vi "FIB MICROSCOPE VIEWER.vi"() -> ()   [LabVIEW 2018]
uses:
  <vilib>/userdefined/High Color/IMAQdx.ctl
  <vilib>/vision/driver/IMAQdx.llb/IMAQdx Attribute Type.ctl
  Mikrodaq/Microdaq FPGA Development/IBA METHODS.ctl
  <vilib>/vision/driver/IMAQdx.llb/IMAQdx Camera Control Mode.ctl
  <vilib>/vision/driver/IMAQdx.llb/IMAQdx Buffer Number Mode.ctl
  <vilib>/Utility/file.llb/Read From Spreadsheet File (string).vi
  <vilib>/Utility/file.llb/Write To Spreadsheet File (DBL).vi
  <vilib>/vision/driver/NI_Vision_Acquisition_Software.lvlib
  <resource>/objmgr/imaqdx.rc
  <vilib>/vision/NI_Vision_Development_Module.lvlib
panel:
  out "CURRENT ZOOM CAL":dbl
  in  "GOTO COMBO":bool=TRUE
  out "QUEU TOGGLE":bool[](array[boolean])
  out "SCAN LIST ARRAY":T2(array[cluster]) {"dQ" format="%_4g"; "DOSE NORM" items=["DWELL TIME", "TOTAL CHARGE", "STEPX"]; "SCAN ORIGIN"."Z" format="%_5g"; "SCAN ORIGIN"."Y" format="%_5g"; "SCAN ORIGIN"."X" format="%_5g"; "SCANNING"."X-AMP" format="%_4f"; "SCANNING"."dX" min=1e-07 max=9.999999999999999e-05 step=1e-07 format="%#_3g"; "SCANNING"."dY" min=1e-07 max=9.999999999999999e-05 step=1e-07 format="%#_3g"; "SCANNING"."Y-AMP" format="%_4f"; "MODE & METHOD"."SCANNING METH" items=["RASTER", "SNAKE RASTER", "SPIRAL RASTER"]; "MODE & METHOD"."SCAN MODE" items=["XY-BEAM", "STEP", "XY-STAGE", "POINT", "SHAPE"]; "Q" format="%_4g"}
  out "POINT":T3={"X"=-0.005539110651703474, "Y"=-0.004695478539077235, "Z"=0.0001} {"Z" format="%_4g"; "X" format="%#_4g"; "Y" format="%#_4g"}
  out "Horizontal Graduated Bar":sgl(slide) scale=0.0..1.0
  in  "SCANNING DIMENSIONS":cluster{"XPIXELS":i32, "YPIXELS":i32}={"XPIXELS"=51, "YPIXELS"=51}
  in  "BUFFERED PIXELS":u32
  out "EXT POINTS ROW":i32
  out "Image Area:Size:All Elements":cluster{"Width":u32, "Height":u32}
  out "NEW ROI":T4
  out "BEAM OFFSET":cluster{"X":dbl[unit], "Y":dbl[unit]}
  out "IMAGE YCENTRE":dbl
  out "IMAGE XCENTRE":dbl
  in  "BINNING":i64=1
  in  "MAPS":enum32{"PIXE", "PIGE"}(tab)
  in  "EXCHANGE":bool
  in  "RECORD AVI VIDEO":bool
  in  "QUESTAR":i32(ring) items=["HOLE", "ZOOM 1", "ZOOM 2", "ZOOM 3"]
  in  "SAMPLE HOLDER":u16(ring)=1 items=["SLIDE HOLDER #1", "GEOSTUB #1", "GEOSTUB #2", "TOMOSTAGE"]
  in  "SCALE BAR":bool
  in  "GRID I":bool
  in  "QUARTZ":bool
  in  "RUBY":bool
  in  "YAG":bool
  in  "YAP":bool
  out "TRANS POINT ARRAY":T5(array[cluster]) {"Z" format="%_4g"; "X" format="%_6g"; "Y" format="%_6f"}
  out "EXT POINTS ARRAY":T5(array[cluster]) {"Z" format="%_4g"; "X" format="%_6g"; "Y" format="%_6f"}
  in  "REFLECTIVITY":bool
  out "ANGLE 2":sgl=1.5516903
  in  "ANGLE":sgl format="%.2f"
  in  "EXPOSURE":dbl(slide)=106.26827541712952 min=1.0 max=2500.0 step=10.0 scale=5.0..5000.0 scale format="%#_3f"
  in  "SCAN QUEU ARRAY":T6(array[cluster]) {"SCANNING MODE AND METHOD"."SCANNING METH" items=["RASTER", "SNAKE RASTER", "SPIRAL RASTER"]; "SCANNING MODE AND METHOD"."SCAN MODE" items=["XY", "STEP", "SHAPE", "STAGE", "COMBO", "POINT", "LINE"]; "DOSE NORM" items=["DWELL TIME", "TOTAL CHARGE", "LIVE CHARGE", "STEPPER PIXELATION"]; "Q PER PULSE" items=["1pC", "0.1pC", "0.01pC"]; "BEAMSCANNING"."dX" min=1e-07 max=9.999999999999999e-05 step=1e-07 format="%_3g"; "BEAMSCANNING"."dY" min=1e-07 max=9.999999999999999e-05 step=1e-07 format="%_3g"; "IBA METHODS" items=["LEFT PIXE", "RIGHT PIXE", "PIGE", "RBS", "HS-IONOLUMINESCENCE", "PIL", "SECONDARY ELECTRONS", "NONE"]; "SCAN ORIGIN"."Z" format="%_6f"; "SCAN ORIGIN"."X" format="%_6f"; "SCAN ORIGIN"."Y" format="%_6f"}
  in  "TOMO POINT":bool
  out "REL XYZ STAGE":T7={"X"=0.005497, "Y"=0.00465, "Z"=-0.0001} {"Z" format="%#_6f"; "X" format="%#_6f"; "Y" format="%#_6f"}
  out "FIB SAMPLE":T8="CSIRO-SAMPLE" caption="Session Out"
  in  "Tab Control 2":T9(tab)
  out "SCAN COMPLETE":bool
  in  "GOTO SCAN ORIGIN":bool
  in  "POSITION":T3 {"Z" format="%_5g"; "Y" format="%_5g"; "X" format="%_5g"}
  in  "START":bool
  in  "PAUSE DATA COLLECTION":bool
  in  "Tab Control 4":T10(tab)
  out "SCAN ROW 2":i32
  in  "START SEQ":bool
  in  "LOAD NMP LIST":bool
  in  "SAVE LIST":bool
  in  "RESET POINTS":bool
  in  "MINUS POINT":bool
  in  "ADD POINT TO LIST":bool
  in  "ION ENERGY":dbl[unit]=4.80652926e-13 format="%_2g"
  in  "BEAM":i8(ring) items=["Protons", "Molecular Hydrogen", "Alpha", "Carbon"]
  in  "NAME":string="test"
  in  "USER":string="jslaird"
  in  "COMMENT":string
  out "SCAN LIST":string[][](table)
  in  "X":bool=TRUE
  in  "Y":bool=TRUE
  in  "Z":bool=TRUE
  in  "GOTO LIST POINT":bool
  in  "SET SCAN FROM LIST":bool
  out "SCAN ROW":i32
  in  "QUEU":bool
  in  "Q":dbl[unit]=2e-09 format="%#_4g"
  in  "DWELL":sgl[unit]=0.1
  in  "PIXEL DEPTH":bool
  in  "dQ":sgl[unit]=1e-10 format="%#_6f"
  in  "dt":sgl[unit]=0.1 caption="dDWELL"
  in  "MIN DWELL":sgl[unit]=0.1
  out "TIME":dbl[unit]=399.9999910593033
  out "CHARGE":dbl[unit]=1.5999999642372133e-06
  in  "LINE PASSES":i32=1
  in  "OVERSCAN":i32=1 min=1 max=100 step=1
  in  "OPTIMISE BEAM":bool
  in  "OBJECT RANGE":i32(ring) items=["100um", "150um", "200um", "250um", "300um", "500um ", "0-1mm Variable", "1mm Aperture", "2mm Aperture", "5mm Aperture", "OPEN"]
  out "Q per PIXEL":dbl[unit] format="%_3g"
  out "TOP  STOP":T3={"X"=-0.005999838337298367, "Y"=-0.004138182607217211, "Z"=9.999999747378752e-05} {"X" format="%_4g"; "Y" format="%#_4g"}
  out "BOTTOM START":T3={"X"=-0.005999838337298367, "Y"=-0.004138182607217211, "Z"=9.999999747378752e-05} {"X" format="%#_4g"; "Y" format="%#_4g"}
  out "DIRECTION":u8(ring) items=["MINUS", "PLUS"]
  out "XAMP":dbl[unit]=0.00044297647174286817 format="%_4g"
  out "XORIGIN":dbl[unit]=-0.02202153716924597 format="%_5g"
  in  "STOP":bool
  in  "START":bool
  out "BOTTOM STOP":T3={"X"=-0.005999838337298367, "Y"=-0.004138182607217211, "Z"=9.999999747378752e-05} {"X" format="%_4g"; "Y" format="%#_4g"}
  out "TOP START":T3={"X"=-0.005999838337298367, "Y"=-0.004138182607217211, "Z"=9.999999747378752e-05} {"X" format="%#_4g"; "Y" format="%#_4g"}
  out "YORIGIN":dbl[unit]
  out "YAMP":dbl[unit]=0.00044297647174286817 format="%_4g"
  out "XAMP":dbl[unit]=0.00044297647174286817 format="%_4g"
  out "XORIGIN":dbl[unit]=-0.02202153716924597 format="%_5g"
  out "YORIGIN":dbl[unit]
  out "YAMP":dbl[unit]=0.00044297647174286817 format="%_4g"
  in  "STOP ROI":bool
  in  "START ROI":bool
  out "BOTTOM RIGHT":T3={"X"=-0.005539110651703474, "Y"=-0.004695478539077235, "Z"=0.0001} {"Z" format="%#_5g"; "X" format="%#_5g"; "Y" format="%#_5g"}
  out "TOP LEFT":T3={"X"=-0.005539110651703474, "Y"=-0.004695478539077235, "Z"=0.0001} {"Z" format="%#_5g"; "X" format="%#_5g"; "Y" format="%#_5g"}
  in  "STAGE VELOCITIES":T11={"XS VEL"=0.002, "YS VEL"=0.002, "Z VEL"=0.001} {"XS VEL" format="%_2f"}
  in  "SCAN CALIBRATIONS":cluster{"XB CAL":dbl[unit], "YB CAL":dbl[unit]}={"XB CAL"=0.00035, "YB CAL"=9.999999999999999e-05}
  in  "SCANNING":T12={"X-AMP"=0.1, "dX"=1e-06, "Y-AMP"=9.999999999999999e-05, "dY"=5e-07, "X-SHIFT"=0.0, "Y-SHIFT"=0.0, "THETA"=0.0, "PHI"=0.0} {"X-AMP" format="%_4f"; "dX" min=1e-07 max=9.999999999999999e-05 step=1e-07 format="%#_3g"; "dY" min=1e-07 max=9.999999999999999e-05 step=1e-07 format="%#_3g"; "Y-AMP" format="%_4f"}
  in  "REPEAT LINE":bool
  in  "MODE & METHOD":cluster{"SCAN MODE":u16, "SCANNING METH":u16}={"SCAN MODE"=2, "SCANNING METH"=1} {"SCANNING METH" items=["RASTER", "SNAKE RASTER", "SPIRAL RASTER"]; "SCAN MODE" items=["XY-BEAM", "STEP", "XY-STAGE", "POINT", "SHAPE"]}
  in  "BEAM CENTRE":bool
  in  "CENTRE STAGE":bool
  in  "SHOW MIRROR":bool=TRUE
  in  "SHOW POSITION":bool=TRUE
  in  "CLEAR ROI":bool
  in  "SHOW BEAM":bool=TRUE
  in  "SHOW SCALE BAR":bool=TRUE
  in  "CAMERA CENTRE":bool=TRUE
  in  "Tab Control":T13(tab)
  in  "RELATIVE":bool
  in  "GOTO GEOSTUB #1 APERTURE":bool=TRUE
  in  "DEFINE APERTURE":bool=TRUE
  in  "RELATIVE MOVE":T3={"X"=-0.004777999999999999, "Y"=-0.0063197, "Z"=9.999999999999999e-05} {"Z" format="%#_5g"; "X" format="%#_5g"; "Y" format="%#_5g"}
  in  "WOBBLEZ":bool
  in  "DOWN":bool
  in  "UP":bool
  in  "DX":dbl[unit]=9.999999999999999e-06 format="%_4f"
  in  "SPEED":u16(ring)=1 items=["SNAIL PACE", "SLOW", "NORMAL", "FAST", "RAPID", "CUSTOM", ""]
  in  "LEFT":bool
  in  "RIGHT":bool
  in  "DZ":dbl[unit]=9.999999999999999e-06 format="%_3f"
  in  "DY":dbl[unit]=9.999999999999999e-06 format="%_3f"
  in  "OUT":bool
  in  "IN":bool
  in  "ABORT":bool
  in  "GOTO POSITION":T3={"X"=-0.004777999999999999, "Y"=-0.0063197, "Z"=9.999999999999999e-05} {"Z" format="%#_5g"; "X" format="%#_5g"; "Y" format="%#_5g"}
  out "SCAN ORIGIN":T3={"X"=-0.005539110651703474, "Y"=-0.004695478539077235, "Z"=0.0001} {"Z" format="%#_5g"; "X" format="%#_5g"; "Y" format="%#_5g"}
  out "LOST CONNECTION?":bool
  in  "BEAM  SCANNER":bool=TRUE
  in  "FARADAY CUP":bool
  in  "Tab Control 5":enum32{"EXTERNAL TRANSLATION", "NOTES"}(tab)
  in  "SET ACCURATE LANDMARK":bool
  in  "TRANS":bool
  out "NMP ORDER OK ?":bool
  in  "GOTOF2":bool
  in  "REF#1":T3={"X"=0.035034294595390356, "Y"=-0.0014485573931861046, "Z"=-0.0018100000000000002} {"Z" format="%#_5g"; "X" format="%#_5g"; "Y" format="%#_5g"}
  in  "REF#2":T3={"X"=0.011754294595390355, "Y"=-0.012118557393186105, "Z"=-0.0015600000000000002} {"Z" format="%#_5g"; "X" format="%#_5g"; "Y" format="%#_5g"}
  in  "GOTOF1":bool
  in  "SET FIDUCIAL 2":bool
  in  "SET FIDUCIAL 1":bool
  in  "LOAD":bool
  in  "SWAP REF#1/REF#2":bool
  in  "SCAN POINT LIST":path=path "C:/Users/jslaird/Dropbox/Working Data/Test Points on Pearce Gold.txt"
  out "EXTERNAL/TRANSLATED LIST":string[][](table)
  in  "GOTO LIST POINT 2":bool
  out "LANDMARKS FOR HOLDERS":T14(array[cluster])=[{"X"=0.0, "Y"=0.0, "Z"=0.0}, {"X"=-0.002142, "Y"=-0.00863, "Z"=0.00093}, {"X"=0.0, "Y"=0.0, "Z"=0.0}, {"X"=0.0, "Y"=0.0, "Z"=0.0}] {"Z" format="%_5g"; "Y" format="%_5g"; "X" format="%_5g"}
  out "XOFFSET":dbl[unit]
  out "YOFFSET":dbl[unit]
  in  "LOAD ROI":bool
  in  "DOSE NORM":i8(ring) items=["DWELL TIME", "TOTAL CHARGE", "STEPX"]
  in  "GLOBAL STOP":bool
  in  "BEAM CURRENT":dbl[unit]=1.0049748420715333e-12 format="%_4f"
  in  "USE CALIBRATION":bool
  in  "CALIBRATE VIEW":bool
  in  "LENGTH 2":bool
  in  "ROTATE VIEW":bool
  in  "SYMMETRY":bool
  in  "DSP ROI":T15
  in  "GAIN METHOD":u16(ring)=2 items=["OFF", "ONCE", "CONTINOUS"]
  in  "GAIN":sgl=1.0 min=0 max=31 step=1
  out "IP ADDRESS":string="192.168.1.10"
  out "CALIBRATION FACTOR":dbl=2.9930842685328876 format="%_4g"
  in  "CONFIGS":u16(ring) items=["MANUAL", "BEAM FOCUS", "SAMPLE VIEWING"]
  in  "IMAGE SYMMETRY":u32(ring)=2 items=["Horizontal", "Vertical", "CENTRAL", "1st Diagonal", "2nd Diagonal"]
  in  "HSCALEBAR POSITION TEXT":cluster{"X":i32, "Y":i32}={"X"=620, "Y"=995}
  in  "VSCALEBAR POSITION":cluster{"X":i32, "Y":i32}={"X"=50, "Y"=250}
  in  "HSCALEBAR POSITION":cluster{"X":i32, "Y":i32}={"X"=440, "Y"=970}
  in  "ZOOM CALIBRATION FACTORS":dbl[](array[numeric])=[1.0, 1.0, 0.8168558457268784, 1.0] format="%_4g"
  in  "ROI ZOOM":bool
  in  "ENABLE VIDEO LOOP":bool=TRUE
  in  "BRIGHT,CONT,GAMMA":cluster{"B":dbl, "C":dbl, "G":dbl}={"B"=250.0, "C"=67.0, "G"=1.6000000000000005} {"G" format="%_4g"; "C" format="%_4g"; "B" format="%_4g"}
  out "LENGTH":dbl=111.88537792376064
  in  "ENABLE STAGE AND DAQ LOOP":bool=TRUE
  out "XBCENTRE":sgl=679.0
  out "YBCENTRE":sgl=512.0
  out "BEAM TO STAGE OFFSETS":cluster{"X":dbl[unit], "Y":dbl[unit]}[](array[cluster])=[{"X"=0.0, "Y"=0.0}, {"X"=-0.00019428571428571433, "Y"=2.8571428571427717e-06}, {"X"=0.0, "Y"=0.0}, {"X"=0.0, "Y"=0.0}] {"X" format="%#_3g"; "Y" format="%#_3g"}
  out "MIRROR HOLE":T16={"Left"=478, "Top"=310, "Right"=546, "Bottom"=372}
  out "ERROR":string
  in  "AVI Path":path=path "C:/Users/jslaird/Desktop/test.avi"
  out "Attribute Information Array":T18(array[cluster])=[{"Attribute Type"=enum."DBL", "Readable"=TRUE, "Writable"=FALSE, "Attribute Name"="AcquisitionAttributes::AdvancedEthernet::BandwidthControl::ActualPeakBandwidth"}, {"Attribute Type"=enum."DBL", "Readable"=TRUE, "Writable"=TRUE, "Attribute Name"="AcquisitionAttributes::AdvancedEthernet::BandwidthControl::DesiredPeakBandwidth"}, {"Attribute Type"=enum."Enum", "Readable"=TRUE, "Writable"=TRUE, "Attribute Name"="AcquisitionAttributes::AdvancedEthernet::Controller::DestinationMode"}, {"Attribute Type"=enum."String", "Readable"=TRUE, "Writable"=TRUE, "Attribute Name"="AcquisitionAttributes::AdvancedEthernet::Controller::DestinationMulticastAddress"}, {"Attribute Type"=enum."Bool", "Readable"=TRUE, "Writable"=TRUE, "Attribute Name"="AcquisitionAttributes::AdvancedEthernet::EventParameters::EventsEnabled"}, {"Attribute Type"=enum."U32", "Readable"=TRUE, "Writable"=TRUE, "Attribute Name"="AcquisitionAttributes::AdvancedEthernet::EventParameters::MaxOutstandingEvents"}, {"Attribute Type"=enum."Bool", "Readable"=TRUE, "Writable"=TRUE, "Attribute Name"="AcquisitionAttributes::AdvancedEthernet::FirewallTraversal::Enabled"}, {"Attribute Type"=enum."U32", "Readable"=TRUE, "Writable"=TRUE, "Attribute Name"="AcquisitionAttributes::AdvancedEthernet::FirewallTraversal::KeepAliveTime"}, {"Attribute Type"=enum."Bool", "Readable"=TRUE, "Writable"=FALSE, "Attribute Name"="AcquisitionAttributes::AdvancedEthernet::FirewallTraversal::Supported"}, {"Attribute Type"=enum."U32", "Readable"=TRUE, "Writable"=TRUE, "Attribute Name"="AcquisitionAttributes::AdvancedEthernet::ResendParameters::MaxResendsPerPacket"}, {"Attribute Type"=enum."U32", "Readable"=TRUE, "Writable"=TRUE, "Attribute Name"="AcquisitionAttributes::AdvancedEthernet::ResendParameters::MemoryWindowSize"}, {"Attribute Type"=enum."U32", "Readable"=TRUE, "Writable"=TRUE, "Attribute Name"="AcquisitionAttributes::AdvancedEthernet::ResendParameters::MissingPacketTimeout"}, {"Attribute Type"=enum."U32", "Readable"=TRUE, "Writable"=TRUE, "Attribute Name"="AcquisitionAttributes::AdvancedEthernet::ResendParameters::NewPacketTimeout"}, {"Attribute Type"=enum."U32", "Readable"=TRUE, "Writable"=TRUE, "Attribute Name"="AcquisitionAttributes::AdvancedEthernet::ResendParameters::ResendBatchingPercentage"}, {"Attribute Type"=enum."U32", "Readable"=TRUE, "Writable"=TRUE, "Attribute Name"="AcquisitionAttributes::AdvancedEthernet::ResendParameters::ResendResponseTimeout"}, {"Attribute Type"=enum."U32", "Readable"=TRUE, "Writable"=TRUE, "Attribute Name"="AcquisitionAttributes::AdvancedEthernet::ResendParameters::ResendThresholdPercentage"}, {"Attribute Type"=enum."U32", "Readable"=TRUE, "Writable"=TRUE, "Attribute Name"="AcquisitionAttributes::AdvancedEthernet::ResendParameters::ResendTimerResolution"}, {"Attribute Type"=enum."Bool", "Readable"=TRUE, "Writable"=TRUE, "Attribute Name"="AcquisitionAttributes::AdvancedEthernet::ResendParameters::ResendsEnabled"}, {"Attribute Type"=enum."U32", "Readable"=TRUE, "Writable"=TRUE, "Attribute Name"="AcquisitionAttributes::AdvancedEthernet::TestPacketParameters::MaxTestPacketRetries"}, {"Attribute Type"=enum."Bool", "Readable"=TRUE, "Writable"=TRUE, "Attribute Name"="AcquisitionAttributes::AdvancedEthernet::TestPacketParameters::TestPacketEnabled"}, {"Attribute Type"=enum."U32", "Readable"=TRUE, "Writable"=TRUE, "Attribute Name"="AcquisitionAttributes::AdvancedEthernet::TestPacketParameters::TestPacketTimeout"}, {"Attribute Type"=enum."Enum", "Readable"=TRUE, "Writable"=TRUE, "Attribute Name"="CameraAttributes::GigE::StreamHold::StreamHoldEnable"}, {"Attribute Type"=enum."I64", "Readable"=TRUE, "Writable"=FALSE, "Attribute Name"="CameraAttributes::GigE::StreamHold::StreamHoldCapacity"}, {"Attribute Type"=enum."I64", "Readable"=TRUE, "Writable"=FALSE, "Attribute Name"="CameraAttributes::GigE::Timestamp::GevTimestampTickFrequency"}, {"Attribute Type"=enum."Command", "Readable"=FALSE, "Writable"=TRUE, "Attribute Name"="CameraAttributes::GigE::Timestamp::GevTimestampControlReset"}, {"Attribute Type"=enum."Enum", "Readable"=TRUE, "Writable"=TRUE, "Attribute Name"="CameraAttributes::GigE::PTP::PtpMode"}, {"Attribute Type"=enum."Enum", "Readable"=TRUE, "Writable"=FALSE, "Attribute Name"="CameraAttributes::GigE::PTP::PtpStatus"}, {"Attribute Type"=enum."I64", "Readable"=TRUE, "Writable"=TRUE, "Attribute Name"="CameraAttributes::GigE::PTP::PtpAcquisitionGateTime"}, {"Attribute Type"=enum."Enum", "Readable"=TRUE, "Writable"=TRUE, "Attribute Name"="CameraAttributes::Acquisition::Trigger::TriggerSelector"}, {"Attribute Type"=enum."Enum", "Readable"=TRUE, "Writable"=TRUE, "Attribute Name"="CameraAttributes::Acquisition::Trigger::TriggerMode"}, {"Attribute Type"=enum."Command", "Readable"=FALSE, "Writable"=TRUE, "Attribute Name"="CameraAttributes::Acquisition::Trigger::TriggerSoftware"}, {"Attribute Type"=enum."Enum", "Readable"=TRUE, "Writable"=TRUE, "Attribute Name"="CameraAttributes::Acquisition::Trigger::TriggerSource"}, {"Attribute Type"=enum."Enum", "Readable"=TRUE, "Writable"=TRUE, "Attribute Name"="CameraAttributes::Acquisition::Trigger::TriggerActivation"}, {"Attribute Type"=enum."Enum", "Readable"=TRUE, "Writable"=TRUE, "Attribute Name"="CameraAttributes::Acquisition::Trigger::TriggerOverlap"}, {"Attribute Type"=enum."DBL", "Readable"=TRUE, "Writable"=TRUE, "Attribute Name"="CameraAttributes::Acquisition::Trigger::TriggerDelayAbs"}, {"Attribute Type"=enum."I64", "Readable"=TRUE, "Writable"=TRUE, "Attribute Name"="CameraAttributes::Controls::DSPSubregion::DSPSubregionLeft"}, {"Attribute Type"=enum."I64", "Readable"=TRUE, "Writable"=TRUE, "Attribute Name"="CameraAttributes::Controls::DSPSubregion::DSPSubregionTop"}, {"Attribute Type"=enum."I64", "Readable"=TRUE, "Writable"=TRUE, "Attribute Name"="CameraAttributes::Controls::DSPSubregion::DSPSubregionRight"}, {"Attribute Type"=enum."I64", "Readable"=TRUE, "Writable"=TRUE, "Attribute Name"="CameraAttributes::Controls::DSPSubregion::DSPSubregionBottom"}, {"Attribute Type"=enum."Enum", "Readable"=TRUE, "Writable"=TRUE, "Attribute Name"="CameraAttributes::Controls::Exposure::ExposureMode"}, {"Attribute Type"=enum."DBL", "Readable"=TRUE, "Writable"=TRUE, "Attribute Name"="CameraAttributes::Controls::Exposure::ExposureTimeAbs"}, {"Attribute Type"=enum."Enum", "Readable"=TRUE, "Writable"=TRUE, "Attribute Name"="CameraAttributes::Controls::Exposure::ExposureAuto"}, {"Attribute Type"=enum."I64", "Readable"=TRUE, "Writable"=TRUE, "Attribute Name"="CameraAttributes::Controls::Exposure::ExposureAutoControl::ExposureAutoTarget"}, {"Attribute Type"=enum."Enum", "Readable"=TRUE, "Writable"=TRUE, "Attribute Name"="CameraAttributes::Controls::Exposure::ExposureAutoControl::ExposureAutoAlg"}, {"Attribute Type"=enum."I64", "Readable"=TRUE, "Writable"=TRUE, "Attribute Name"="CameraAttributes::Controls::Exposure::ExposureAutoControl::ExposureAutoMin"}, {"Attribute Type"=enum."I64", "Readable"=TRUE, "Writable"=TRUE, "Attribute Name"="CameraAttributes::Controls::Exposure::ExposureAutoControl::ExposureAutoMax"}, {"Attribute Type"=enum."I64", "Readable"=TRUE, "Writable"=TRUE, "Attribute Name"="CameraAttributes::Controls::Exposure::ExposureAutoControl::ExposureAutoRate"}, {"Attribute Type"=enum."I64", "Readable"=TRUE, "Writable"=TRUE, "Attribute Name"="CameraAttributes::Controls::Exposure::ExposureAutoControl::ExposureAutoOutliers"}, {"Attribute Type"=enum."I64", "Readable"=TRUE, "Writable"=TRUE, "Attribute Name"="CameraAttributes::Controls::Exposure::ExposureAutoControl::ExposureAutoAdjustTol"}, {"Attribute Type"=enum."Enum", "Readable"=TRUE, "Writable"=TRUE, "Attribute Name"="CameraAttributes::Controls::GainControl::GainSelector"}, {"Attribute Type"=enum."I64", "Readable"=TRUE, "Writable"=TRUE, "Attribute Name"="CameraAttributes::Controls::GainControl::GainRaw"}, {"Attribute Type"=enum."Enum", "Readable"=TRUE, "Writable"=TRUE, "Attribute Name"="CameraAttributes::Controls::GainControl::GainAuto"}, {"Attribute Type"=enum."I64", "Readable"=TRUE, "Writable"=TRUE, "Attribute Name"="CameraAttributes::Controls::GainControl::GainAutoControl::GainAutoTarget"}, {"Attribute Type"=enum."I64", "Readable"=TRUE, "Writable"=TRUE, "Attribute Name"="CameraAttributes::Controls::GainControl::GainAutoControl::GainAutoMin"}, {"Attribute Type"=enum."I64", "Readable"=TRUE, "Writable"=TRUE, "Attribute Name"="CameraAttributes::Controls::GainControl::GainAutoControl::GainAutoMax"}, {"Attribute Type"=enum."I64", "Readable"=TRUE, "Writable"=TRUE, "Attribute Name"="CameraAttributes::Controls::GainControl::GainAutoControl::GainAutoRate"}, {"Attribute Type"=enum."I64", "Readable"=TRUE, "Writable"=TRUE, "Attribute Name"="CameraAttributes::Controls::GainControl::GainAutoControl::GainAutoOutliers"}, {"Attribute Type"=enum."I64", "Readable"=TRUE, "Writable"=TRUE, "Attribute Name"="CameraAttributes::Controls::GainControl::GainAutoControl::GainAutoAdjustTol"}, {"Attribute Type"=enum."Enum", "Readable"=TRUE, "Writable"=TRUE, "Attribute Name"="CameraAttributes::Controls::BlackLevelControl::BlackLevelSelector"}, {"Attribute Type"=enum."Enum", "Readable"=TRUE, "Writable"=TRUE, "Attribute Name"="CameraAttributes::Controls::Iris::IrisMode"}, {"Attribute Type"=enum."I64", "Readable"=TRUE, "Writable"=TRUE, "Attribute Name"="CameraAttributes::Controls::Iris::IrisAutoTarget"}, {"Attribute Type"=enum."I64", "Readable"=TRUE, "Writable"=FALSE, "Attribute Name"="CameraAttributes::Controls::Iris::IrisVideoLevel"}, {"Attribute Type"=enum."I64", "Readable"=TRUE, "Writable"=TRUE, "Attribute Name"="CameraAttributes::Controls::Iris::IrisVideoLevelMin"}, {"Attribute Type"=enum."I64", "Readable"=TRUE, "Writable"=TRUE, "Attribute Name"="CameraAttributes::Controls::Iris::IrisVideoLevelMax"}, {"Attribute Type"=enum."I64", "Readable"=FALSE, "Writable"=FALSE, "Attribute Name"="CameraAttributes::Controls::LUTControl::LUTValue"}, {"Attribute Type"=enum."I64", "Readable"=TRUE, "Writable"=FALSE, "Attribute Name"="CameraAttributes::IO::SyncIn::SyncInLevels"}, {"Attribute Type"=enum."Enum", "Readable"=TRUE, "Writable"=TRUE, "Attribute Name"="CameraAttributes::IO::SyncIn::SyncInSelector"}, {"Attribute Type"=enum."I64", "Readable"=TRUE, "Writable"=TRUE, "Attribute Name"="CameraAttributes::IO::SyncIn::SyncInGlitchFilter"}, {"Attribute Type"=enum."I64", "Readable"=TRUE, "Writable"=TRUE, "Attribute Name"="CameraAttributes::IO::SyncOut::SyncOutLevels"}, {"Attribute Type"=enum."Enum", "Readable"=TRUE, "Writable"=TRUE, "Attribute Name"="CameraAttributes::IO::SyncOut::SyncOutSelector"}, {"Attribute Type"=enum."Enum", "Readable"=TRUE, "Writable"=TRUE, "Attribute Name"="CameraAttributes::IO::SyncOut::SyncOutSource"}, {"Attribute Type"=enum."Enum", "Readable"=TRUE, "Writable"=TRUE, "Attribute Name"="CameraAttributes::IO::SyncOut::SyncOutPolarity"}, {"Attribute Type"=enum."Enum", "Readable"=TRUE, "Writable"=TRUE, "Attribute Name"="CameraAttributes::IO::Strobe::StrobeSource"}, {"Attribute Type"=enum."Enum", "Readable"=TRUE, "Writable"=TRUE, "Attribute Name"="CameraAttributes::IO::Strobe::StrobeDurationMode"}, {"Attribute Type"=enum."I64", "Readable"=TRUE, "Writable"=TRUE, "Attribute Name"="CameraAttributes::IO::Strobe::StrobeDelay"}, {"Attribute Type"=enum."I64", "Readable"=TRUE, "Writable"=TRUE, "Attribute Name"="CameraAttributes::IO::Strobe::StrobeDuration"}, {"Attribute Type"=enum."I64", "Readable"=TRUE, "Writable"=FALSE, "Attribute Name"="CameraAttributes::EventControl::EventID::EventAcquisitionStart"}, {"Attribute Type"=enum."I64", "Readable"=TRUE, "Writable"=FALSE, "Attribute Name"="CameraAttributes::EventControl::EventID::EventAcquisitionEnd"}, {"Attribute Type"=enum."I64", "Readable"=TRUE, "Writable"=FALSE, "Attribute Name"="CameraAttributes::EventControl::EventID::EventFrameTrigger"}, {"Attribute Type"=enum."I64", "Readable"=TRUE, "Writable"=FALSE, "Attribute Name"="CameraAttributes::EventControl::EventID::EventExposureEnd"}, {"Attribute Type"=enum."I64", "Readable"=TRUE, "Writable"=FALSE, "Attribute Name"="CameraAttributes::EventControl::EventID::EventAcquisitionRecordTrigger"}, {"Attribute Type"=enum."I64", "Readable"=TRUE, "Writable"=FALSE, "Attribute Name"="CameraAttributes::EventControl::EventID::EventLine1RisingEdge"}, {"Attribute Type"=enum."I64", "Readable"=TRUE, "Writable"=FALSE, "Attribute Name"="CameraAttributes::EventControl::EventID::EventLine1FallingEdge"}, {"Attribute Type"=enum."I64", "Readable"=TRUE, "Writable"=FALSE, "Attribute Name"="CameraAttributes::EventControl::EventID::EventLine2RisingEdge"}, {"Attribute Type"=enum."I64", "Readable"=TRUE, "Writable"=FALSE, "Attribute Name"="CameraAttributes::EventControl::EventID::EventLine2FallingEdge"}, {"Attribute Type"=enum."I64", "Readable"=TRUE, "Writable"=FALSE, "Attribute Name"="CameraAttributes::EventControl::EventID::EventLine3RisingEdge"}, {"Attribute Type"=enum."I64", "Readable"=TRUE, "Writable"=FALSE, "Attribute Name"="CameraAttributes::EventControl::EventID::EventLine3FallingEdge"}, {"Attribute Type"=enum."I64", "Readable"=TRUE, "Writable"=FALSE, "Attribute Name"="CameraAttributes::EventControl::EventID::EventLine4RisingEdge"}, {"Attribute Type"=enum."I64", "Readable"=TRUE, "Writable"=FALSE, "Attribute Name"="CameraAttributes::EventControl::EventID::EventLine4FallingEdge"}, {"Attribute Type"=enum."I64", "Readable"=TRUE, "Writable"=FALSE, "Attribute Name"="CameraAttributes::EventControl::EventID::EventFrameTriggerReady"}, {"Attribute Type"=enum."I64", "Readable"=TRUE, "Writable"=FALSE, "Attribute Name"="CameraAttributes::EventControl::EventID::EventPtpSyncLost"}, {"Attribute Type"=enum."I64", "Readable"=TRUE, "Writable"=FALSE, "Attribute Name"="CameraAttributes::EventControl::EventID::EventPtpSyncLocked"}, {"Attribute Type"=enum."I64", "Readable"=TRUE, "Writable"=FALSE, "Attribute Name"="CameraAttributes::EventControl::EventID::EventOverflow"}, {"Attribute Type"=enum."I64", "Readable"=TRUE, "Writable"=FALSE, "Attribute Name"="CameraAttributes::EventControl::EventID::EventError"}, {"Attribute Type"=enum."U32", "Readable"=TRUE, "Writable"=TRUE, "Attribute Name"="AcquisitionAttributes::AdvancedGenicam::CommandTimeout"}, {"Attribute Type"=enum."Bool", "Readable"=TRUE, "Writable"=TRUE, "Attribute Name"="AcquisitionAttributes::AdvancedGenicam::IgnoreCameraValidationErrors"}, {"Attribute Type"=enum."Enum", "Readable"=TRUE, "Writable"=TRUE, "Attribute Name"="AcquisitionAttributes::Bayer::Algorithm"}, {"Attribute Type"=enum."DBL", "Readable"=TRUE, "Writable"=TRUE, "Attribute Name"="AcquisitionAttributes::Bayer::GainB"}, {"Attribute Type"=enum."DBL", "Readable"=TRUE, "Writable"=TRUE, "Attribute Name"="AcquisitionAttributes::Bayer::GainG"}, {"Attribute Type"=enum."DBL", "Readable"=TRUE, "Writable"=TRUE, "Attribute Name"="AcquisitionAttributes::Bayer::GainR"}, {"Attribute Type"=enum."Enum", "Readable"=TRUE, "Writable"=TRUE, "Attribute Name"="AcquisitionAttributes::Bayer::Pattern"}, {"Attribute Type"=enum."Bool", "Readable"=TRUE, "Writable"=TRUE, "Attribute Name"="AcquisitionAttributes::ChunkDataDecoding::ChunkDataDecodingEnabled"}, {"Attribute Type"=enum."U32", "Readable"=TRUE, "Writable"=TRUE, "Attribute Name"="AcquisitionAttributes::ChunkDataDecoding::MaximumChunkCopySize"}, {"Attribute Type"=enum."I64", "Readable"=TRUE, "Writable"=FALSE, "Attribute Name"="CameraAttributes::Info::FirmwareVerMajor"}, {"Attribute Type"=enum."I64", "Readable"=TRUE, "Writable"=FALSE, "Attribute Name"="CameraAttributes::Info::FirmwareVerMinor"}, {"Attribute Type"=enum."I64", "Readable"=TRUE, "Writable"=FALSE, "Attribute Name"="CameraAttributes::Info::FirmwareVerBuild"}, {"Attribute Type"=enum."Enum", "Readable"=TRUE, "Writable"=FALSE, "Attribute Name"="CameraAttributes::Info::SensorType"}, {"Attribute Type"=enum."I64", "Readable"=TRUE, "Writable"=FALSE, "Attribute Name"="CameraAttributes::Info::SensorBits"}, {"Attribute Type"=enum."String", "Readable"=TRUE, "Writable"=FALSE, "Attribute Name"="CameraAttributes::Info::DeviceVendorName"}, {"Attribute Type"=enum."String", "Readable"=TRUE, "Writable"=FALSE, "Attribute Name"="CameraAttributes::Info::DeviceModelName"}, {"Attribute Type"=enum."String", "Readable"=TRUE, "Writable"=FALSE, "Attribute Name"="CameraAttributes::Info::DeviceFirmwareVersion"}, {"Attribute Type"=enum."String", "Readable"=TRUE, "Writable"=FALSE, "Attribute Name"="CameraAttributes::Info::DeviceID"}, {"Attribute Type"=enum."String", "Readable"=TRUE, "Writable"=FALSE, "Attribute Name"="CameraAttributes::Info::DevicePartNumber"}, {"Attribute Type"=enum."Enum", "Readable"=TRUE, "Writable"=FALSE, "Attribute Name"="CameraAttributes::Info::DeviceScanType"}, {"Attribute Type"=enum."I64", "Readable"=TRUE, "Writable"=TRUE, "Attribute Name"="CameraAttributes::GigE::StreamBytesPerSecond"}, {"Attribute Type"=enum."Enum", "Readable"=TRUE, "Writable"=TRUE, "Attribute Name"="CameraAttributes::GigE::BandwidthControlMode"}, {"Attribute Type"=enum."Bool", "Readable"=TRUE, "Writable"=TRUE, "Attribute Name"="CameraAttributes::GigE::ChunkModeActive"}, {"Attribute Type"=enum."I64", "Readable"=TRUE, "Writable"=FALSE, "Attribute Name"="CameraAttributes::GigE::PayloadSize"}, {"Attribute Type"=enum."I64", "Readable"=TRUE, "Writable"=FALSE, "Attribute Name"="CameraAttributes::GigE::NonImagePayloadSize"}, {"Attribute Type"=enum."Bool", "Readable"=TRUE, "Writable"=TRUE, "Attribute Name"="CameraAttributes::GigE::StreamFrameRateConstrain"}, {"Attribute Type"=enum."Enum", "Readable"=TRUE, "Writable"=TRUE, "Attribute Name"="CameraAttributes::Acquisition::AcquisitionMode"}, {"Attribute Type"=enum."I64", "Readable"=TRUE, "Writable"=TRUE, "Attribute Name"="CameraAttributes::Acquisition::AcquisitionFrameCount"}, {"Attribute Type"=enum."DBL", "Readable"=TRUE, "Writable"=TRUE, "Attribute Name"="CameraAttributes::Acquisition::AcquisitionFrameRateAbs"}, {"Attribute Type"=enum."DBL", "Readable"=TRUE, "Writable"=FALSE, "Attribute Name"="CameraAttributes::Acquisition::AcquisitionFrameRateLimit"}, {"Attribute Type"=enum."I64", "Readable"=TRUE, "Writable"=TRUE, "Attribute Name"="CameraAttributes::Acquisition::RecorderPreEventCount"}, {"Attribute Type"=enum."I64", "Readable"=TRUE, "Writable"=FALSE, "Attribute Name"="CameraAttributes::ImageMode::SensorWidth"}, {"Attribute Type"=enum."I64", "Readable"=TRUE, "Writable"=FALSE, "Attribute Name"="CameraAttributes::ImageMode::SensorHeight"}, {"Attribute Type"=enum."I64", "Readable"=TRUE, "Writable"=TRUE, "Attribute Name"="CameraAttributes::ImageMode::BinningHorizontal"}, {"Attribute Type"=enum."I64", "Readable"=TRUE, "Writable"=TRUE, "Attribute Name"="CameraAttributes::ImageMode::BinningVertical"}, {"Attribute Type"=enum."I64", "Readable"=TRUE, "Writable"=FALSE, "Attribute Name"="CameraAttributes::ImageFormat::WidthMax"}, {"Attribute Type"=enum."I64", "Readable"=TRUE, "Writable"=FALSE, "Attribute Name"="CameraAttributes::ImageFormat::HeightMax"}, {"Attribute Type"=enum."Enum", "Readable"=TRUE, "Writable"=TRUE, "Attribute Name"="CameraAttributes::ImageFormat::PixelFormat"}, {"Attribute Type"=enum."I64", "Readable"=TRUE, "Writable"=TRUE, "Attribute Name"="CameraAttributes::ImageFormat::Width"}, {"Attribute Type"=enum."I64", "Readable"=TRUE, "Writable"=TRUE, "Attribute Name"="CameraAttributes::ImageFormat::Height"}, {"Attribute Type"=enum."I64", "Readable"=TRUE, "Writable"=TRUE, "Attribute Name"="CameraAttributes::ImageFormat::OffsetX"}, {"Attribute Type"=enum."I64", "Readable"=TRUE, "Writable"=TRUE, "Attribute Name"="CameraAttributes::ImageFormat::OffsetY"}, {"Attribute Type"=enum."I64", "Readable"=TRUE, "Writable"=FALSE, "Attribute Name"="CameraAttributes::ImageFormat::ImageSize"}, {"Attribute Type"=enum."Enum", "Readable"=TRUE, "Writable"=TRUE, "Attribute Name"="CameraAttributes::EventControl::EventSelector"}, {"Attribute Type"=enum."Enum", "Readable"=TRUE, "Writable"=TRUE, "Attribute Name"="CameraAttributes::EventControl::EventNotification"}, {"Attribute Type"=enum."I64", "Readable"=TRUE, "Writable"=TRUE, "Attribute Name"="CameraAttributes::EventControl::EventsEnable1"}, {"Attribute Type"=enum."Enum", "Readable"=TRUE, "Writable"=TRUE, "Attribute Name"="CameraAttributes::SavedUserSets::UserSetSelector"}, {"Attribute Type"=enum."Command", "Readable"=FALSE, "Writable"=TRUE, "Attribute Name"="CameraAttributes::SavedUserSets::UserSetLoad"}, {"Attribute Type"=enum."Command", "Readable"=FALSE, "Writable"=TRUE, "Attribute Name"="CameraAttributes::SavedUserSets::UserSetSave"}, {"Attribute Type"=enum."Enum", "Readable"=TRUE, "Writable"=TRUE, "Attribute Name"="CameraAttributes::SavedUserSets::UserSetDefaultSelector"}, {"Attribute Type"=enum."Enum", "Readable"=TRUE, "Writable"=TRUE, "Attribute Name"="AcquisitionAttributes::BitsPerPixel"}, {"Attribute Type"=enum."Enum", "Readable"=TRUE, "Writable"=TRUE, "Attribute Name"="AcquisitionAttributes::ImageDecoderCopyMode"}, {"Attribute Type"=enum."Enum", "Readable"=TRUE, "Writable"=TRUE, "Attribute Name"="AcquisitionAttributes::IncompleteBufferMode"}, {"Attribute Type"=enum."Enum", "Readable"=TRUE, "Writable"=TRUE, "Attribute Name"="AcquisitionAttributes::OutputImageType"}, {"Attribute Type"=enum."Enum", "Readable"=TRUE, "Writable"=TRUE, "Attribute Name"="AcquisitionAttributes::OverwriteMode"}, {"Attribute Type"=enum."U32", "Readable"=TRUE, "Writable"=TRUE, "Attribute Name"="AcquisitionAttributes::PacketSize"}, {"Attribute Type"=enum."Enum", "Readable"=TRUE, "Writable"=TRUE, "Attribute Name"="AcquisitionAttributes::ReceiveTimestampMode"}, {"Attribute Type"=enum."Bool", "Readable"=TRUE, "Writable"=TRUE, "Attribute Name"="AcquisitionAttributes::ShiftPixelBits"}, {"Attribute Type"=enum."Bool", "Readable"=TRUE, "Writable"=TRUE, "Attribute Name"="AcquisitionAttributes::SwapPixelBytes"}, {"Attribute Type"=enum."U32", "Readable"=TRUE, "Writable"=TRUE, "Attribute Name"="AcquisitionAttributes::Timeout"}, {"Attribute Type"=enum."U32", "Readable"=TRUE, "Writable"=FALSE, "Attribute Name"="CameraInformation::BaseAddress"}, {"Attribute Type"=enum."Enum", "Readable"=TRUE, "Writable"=FALSE, "Attribute Name"="CameraInformation::BusType"}, {"Attribute Type"=enum."String", "Readable"=TRUE, "Writable"=FALSE, "Attribute Name"="CameraInformation::HostIPAddress"}, {"Attribute Type"=enum."String", "Readable"=TRUE, "Writable"=FALSE, "Attribute Name"="CameraInformation::HostMACAddress"}, {"Attribute Type"=enum."String", "Readable"=TRUE, "Writable"=FALSE, "Attribute Name"="CameraInformation::IPAddress"}, {"Attribute Type"=enum."String", "Readable"=TRUE, "Writable"=FALSE, "Attribute Name"="CameraInformation::ModelName"}, {"Attribute Type"=enum."String", "Readable"=TRUE, "Writable"=FALSE, "Attribute Name"="CameraInformation::PrimaryURLString"}, {"Attribute Type"=enum."String", "Readable"=TRUE, "Writable"=FALSE, "Attribute Name"="CameraInformation::SecondaryURLString"}, {"Attribute Type"=enum."U32", "Readable"=TRUE, "Writable"=FALSE, "Attribute Name"="CameraInformation::SerialNumberHigh"}, {"Attribute Type"=enum."U32", "Readable"=TRUE, "Writable"=FALSE, "Attribute Name"="CameraInformation::SerialNumberLow"}, {"Attribute Type"=enum."String", "Readable"=TRUE, "Writable"=FALSE, "Attribute Name"="CameraInformation::VendorName"}, {"Attribute Type"=enum."Bool", "Readable"=TRUE, "Writable"=FALSE, "Attribute Name"="StatusInformation::AcqInProgress"}, {"Attribute Type"=enum."I64", "Readable"=TRUE, "Writable"=FALSE, "Attribute Name"="StatusInformation::HandledEventCount"}, {"Attribute Type"=enum."I64", "Readable"=TRUE, "Writable"=FALSE, "Attribute Name"="StatusInformation::IncompleteBufferCount"}, {"Attribute Type"=enum."I64", "Readable"=TRUE, "Writable"=FALSE, "Attribute Name"="StatusInformation::LastBufferCount"}, {"Attribute Type"=enum."U32", "Readable"=TRUE, "Writable"=FALSE, "Attribute Name"="StatusInformation::LastBufferNumber"}, {"Attribute Type"=enum."I64", "Readable"=TRUE, "Writable"=FALSE, "Attribute Name"="StatusInformation::LostBufferCount"}, {"Attribute Type"=enum."I64", "Readable"=TRUE, "Writable"=FALSE, "Attribute Name"="StatusInformation::LostEventCount"}, {"Attribute Type"=enum."I64", "Readable"=TRUE, "Writable"=FALSE, "Attribute Name"="StatusInformation::LostPacketCount"}, {"Attribute Type"=enum."I64", "Readable"=TRUE, "Writable"=FALSE, "Attribute Name"="StatusInformation::ReceivedResendPackets"}, {"Attribute Type"=enum."I64", "Readable"=TRUE, "Writable"=FALSE, "Attribute Name"="StatusInformation::RequestedResendPacketCount"}]
  in  "BEAM CENTRE MARK":cluster{"L":i32, "T":i32, "R":i32, "B":i32}[](array[cluster])=[{"L"=674, "T"=517, "R"=684, "B"=507}, {"L"=640, "T"=479, "R"=660, "B"=459}, {"L"=591, "T"=438, "R"=611, "B"=418}, {"L"=669, "T"=529, "R"=689, "B"=509}]
  out "YC":dbl[unit]
  out "XC":dbl[unit]
  out "BOTTOMY":i32=341
  out "BOTTOMX":i32=512
  out "TOPX":i32=512
  out "TOPY":i32=341
  out "Contours":T19(array[cluster])=[{"Contour Type"=0, "ROI Type"=3, "Points"=[478, 310, 546, 372]}]
  out "CENTRE CAMERA FOV":T20={"Numeric Control"=677, "Numeric Control"=510}
  in  "SCAN ROI":T4={"Global Rectangle"=[682, 277, 710, 307], "Contours"=[{"Contour Type"=0, "ROI Type"=3, "Points"=[682, 277, 710, 307]}]}
  out "ActualPeakBandwidth":dbl=1000.0
  out "YCENTRE":sgl=488.0
  out "XCENTRE":sgl=612.0
  out "IMAGE XPIXELS":u32=1360
  out "IMAGE YPIXELS":u32=1024
  in  "QUEU PATH":path
  out "VI REFERENCE":refnum<vi>
  out "DisplayName":string
  out "VSCALEBAR":u32[][](array[colorbox])
  out "HSCALEBAR":u32[][](array[colorbox])
  out "MICROSCOPE":T21(plugin-control)
  # "0.1pC ---MAX i ~ 30nA"
  # "0.01pC ---MAX i ~ 3nA"
  # "per pass"
  # "LHS = X1 (x,y) < XII (x,y) for both x and y"
  # "RHS"
  # "LHS"
  # "+Xs"
  # "+Ys"
  # "+Ys"
  # "+Xs"
  # "+Zs"
  # "um/pixel"
  # "Zoom 2 cal on 1000 mesh"
  # "Zero distance b/w ZERO on GeLi \ni.e electrical touch is at -3.257mm"
types:
  T1 = typedef "IBA METHODS.ctl" = cluster{"CHARGE":bool, "PIXE":bool, "PIGE":bool, "RBS":bool, "IBIC":bool, "HSIL":bool}
  T2 = cluster{"POINT":string, "COMMENT":string, "DWELL":sgl[unit], "LINE PASSES":i32, "Q":dbl[unit], "MODE & METHOD":cluster{"SCAN MODE":u16, "SCANNING METH":u16}, "IBA CHANNELS 2":T1, "OVERSCAN ":i32, "SCANNING":cluster{"X-AMP":dbl[unit], "dX":dbl[unit], "Y-AMP":dbl[unit], "dY":dbl[unit], "X-SHIFT":dbl[unit], "Y-SHIFT":dbl[unit], "THETA":dbl, "PHI":dbl}, "SCAN ORIGIN ":cluster{"X":dbl[unit], "Y":dbl[unit], "Z":dbl[unit]}, "PIXEL DEPTH":bool, "DOSE NORM":i8, "dQ":dbl[unit], "dt":sgl[unit], "FLY MODE":bool}[]
  T3 = cluster{"X":dbl[unit], "Y":dbl[unit], "Z":dbl[unit]}
  T4 = cluster{"Global Rectangle":i32[], "Contours":cluster{"Contour Type":u32, "ROI Type":u32, "Points":i32[]}[]}
  T5 = cluster{"POINT":string, "X":dbl[unit], "Y":dbl[unit], "Z":dbl[unit], "COMMENT":string}[]
  T6 = cluster{"NAME":string, "IBA METHODS":i8[], "SCAN ORIGIN":cluster{"X":dbl[unit], "Y":dbl[unit], "Z":dbl[unit]}, " STAGE SCANNING":cluster{"X-AMP":dbl[unit], "Y-AMP":dbl[unit], "dY":dbl[unit], "dX":dbl[unit], "Y-SHIFT":dbl[unit], "X-SHIFT":dbl[unit]}, "BEAMSCANNING":cluster{"X-AMP":dbl[unit], "dX":dbl[unit], "Y-AMP":dbl[unit], "dY":dbl[unit], "X-SHIFT":dbl[unit], "Y-SHIFT":dbl[unit], "CORR":bool, "THETA":dbl, "PHI":dbl, "X I":i32, "Y I":i32}, "COMMENT":string, "Q PER PULSE":u16, "DWELL":sgl[unit], "Q PER PIXEL":dbl[unit], "DOSE NORM":i8, "NO PASSES":i32, "SCANNING MODE AND METHOD":cluster{"SCAN MODE":u16, "SCANNING METH":u16}}[]
  T7 = cluster{"X":sgl[unit], "Y":sgl[unit], "Z":sgl[unit]}
  T8 = typedef "IMAQdx.ctl" = refnum<k21>
  T9 = enum32{"MIKRODAQ", "CAMERA", "STAGE DEFINITIONS"}
  T10 = enum32{"SCAN LIST", "MODES", "STEP", "ROI", "SCAN PARAMETERS"}
  T11 = cluster{"XS VEL":sgl[unit], "YS VEL":sgl[unit], "Z VEL":sgl[unit]}
  T12 = cluster{"X-AMP":dbl[unit], "dX":dbl[unit], "Y-AMP":dbl[unit], "dY":dbl[unit], "X-SHIFT":dbl[unit], "Y-SHIFT":dbl[unit], "THETA":dbl, "PHI":dbl}
  T13 = enum32{"XYZ STAGE ", "GEOMETRY", "RRULER CALIBRATION"}
  T14 = cluster{"X":dbl[unit], "Y":dbl[unit], "Z":dbl[unit]}[]
  T15 = cluster{"LEFT":u32, "RIGHT":u32, "TOP":u32, "BOTTOM":u32}
  T16 = cluster{"Left":i32, "Top":i32, "Right":i32, "Bottom":i32}
  T17 = typedef "NI_Vision_Acquisition_Software.lvlib/IMAQdx Attribute Type.ctl" = enum32{"U32", "I64", "DBL", "String", "Enum", "Bool", "Command"}
  T18 = cluster{"Attribute Type":T17, "Readable":bool, "Writable":bool, "Attribute Name":string}[]
  T19 = cluster{"Contour Type":u32, "ROI Type":u32, "Points":i32[]}[]
  T20 = cluster{"Numeric Control":i32, "Numeric Control":i32}
  T21 = typedef "IMAQ Image.ctl" = refnum<image>
  T22 = typedef "NI_Vision_Acquisition_Software.lvlib/IMAQdx Camera Control Mode.ctl" = enum32{"Controller", "Listener"}
  T23 = typedef "NI_Vision_Acquisition_Software.lvlib/IMAQdx Buffer Number Mode.ctl" = enum32{"Next", "Last", "Buffer Number", "Every", "Last New"}
  T24 = typedef "Image Unit" = enum32{"Undefined", "Angström", "Micrometer", "Millimeter", "Centimeter", "Meter", "Kilometer", "Microinch", "Inch", "Feet", "Nautical miles", "Standard miles", "Steps"}
  T25 = cluster{"Desired Font (Application)":enum16{"User-specified Font", "Application Font", "System Font", "Dialog Font"}, "[User-specified Font]":cluster{"Font Name":string, "Size":i16, "Strikeout?":bool, "Italic?":bool, "Underline?":bool, "Outline?":bool, "Shadow?":bool, "Bold?":bool, "Rotation Angle":dbl}, "Horizontal Alignment":i16, "Vertical Alignment":i16}
  T26 = enum16{"None", "On Hover", "On Key Focus", "On Hover or Key Focus"}
  T27 = enum8{"Enabled", "Disabled", "Disabled and Grayed Out"}
  T28 = typedef "LVAllMonitorsDisplayTypeDef.ctl" = cluster{"Bounds":cluster{"Left":i16, "Top":i16, "Right":i16, "Bottom":i16}, "Depth":i16}[]
  T29 = cluster{"Disp.AllMonitors[0]":cluster{"Bounds":cluster{"Left":i16, "Top":i16, "Right":i16, "Bottom":i16}, "Depth":i16}, "Disp.AllMonitors[1]":cluster{"Bounds":cluster{"Left":i16, "Top":i16, "Right":i16, "Bottom":i16}, "Depth":i16}, "Disp.AllMonitors[2]":cluster{"Bounds":cluster{"Left":i16, "Top":i16, "Right":i16, "Bottom":i16}, "Depth":i16}, "Disp.AllMonitors[3]":cluster{"Bounds":cluster{"Left":i16, "Top":i16, "Right":i16, "Bottom":i16}, "Depth":i16}, "Disp.AllMonitors[4]":cluster{"Bounds":cluster{"Left":i16, "Top":i16, "Right":i16, "Bottom":i16}, "Depth":i16}, "Disp.AllMonitors[5]":cluster{"Bounds":cluster{"Left":i16, "Top":i16, "Right":i16, "Bottom":i16}, "Depth":i16}, "Disp.AllMonitors[6]":cluster{"Bounds":cluster{"Left":i16, "Top":i16, "Right":i16, "Bottom":i16}, "Depth":i16}, "Disp.AllMonitors[7]":cluster{"Bounds":cluster{"Left":i16, "Top":i16, "Right":i16, "Bottom":i16}, "Depth":i16}, "Disp.AllMonitors[8]":cluster{"Bounds":cluster{"Left":i16, "Top":i16, "Right":i16, "Bottom":i16}, "Depth":i16}}
  T30 = cluster{"Bounds":cluster{"Left":i16, "Top":i16, "Right":i16, "Bottom":i16}, "Depth":i16}
  T31 = cluster{"Left":i16, "Top":i16, "Right":i16, "Bottom":i16}
  T32 = typedef "Image Type" = u32
  T33 = cluster{"Attribute Type":T17, "Readable":bool, "Writable":bool, "Attribute Name":string}
  T34 = typedef "IMAQ AVI2 Refnum.ctl" = refnum<k20>
  T35 = cluster{"CALI FACTOR ":dbl, "CALI FACTOR ":dbl, "Unit":T24}
  T36 = cluster{"Contour Type":u32, "ROI Type":u32, "Points":i32[]}
  T37 = cluster{"Numeric Control":i32, "Numeric Control":i32, "Numeric Control":i32, "Numeric Control":i32}
  T38 = typedef "LVRowAndColumnTypeDef.ctl" = cluster{"Row":i32, "Column":i32}
  T39 = cluster{"POINT":string, "COMMENT":string, "DWELL":sgl[unit], "LINE PASSES":i32, "Q":dbl[unit], "MODE & METHOD":cluster{"SCAN MODE":u16, "SCANNING METH":u16}, "IBA CHANNELS 2":T1, "OVERSCAN ":i32, "SCANNING":cluster{"X-AMP":dbl[unit], "dX":dbl[unit], "Y-AMP":dbl[unit], "dY":dbl[unit], "X-SHIFT":dbl[unit], "Y-SHIFT":dbl[unit], "THETA":dbl, "PHI":dbl}, "SCAN ORIGIN ":cluster{"X":dbl[unit], "Y":dbl[unit], "Z":dbl[unit]}, "PIXEL DEPTH":bool, "DOSE NORM":i8, "dQ":dbl[unit], "dt":sgl[unit], "FLY MODE":bool}
  T40 = cluster{"POINT":string, "X":dbl[unit], "Y":dbl[unit], "Z":dbl[unit], "COMMENT":string}
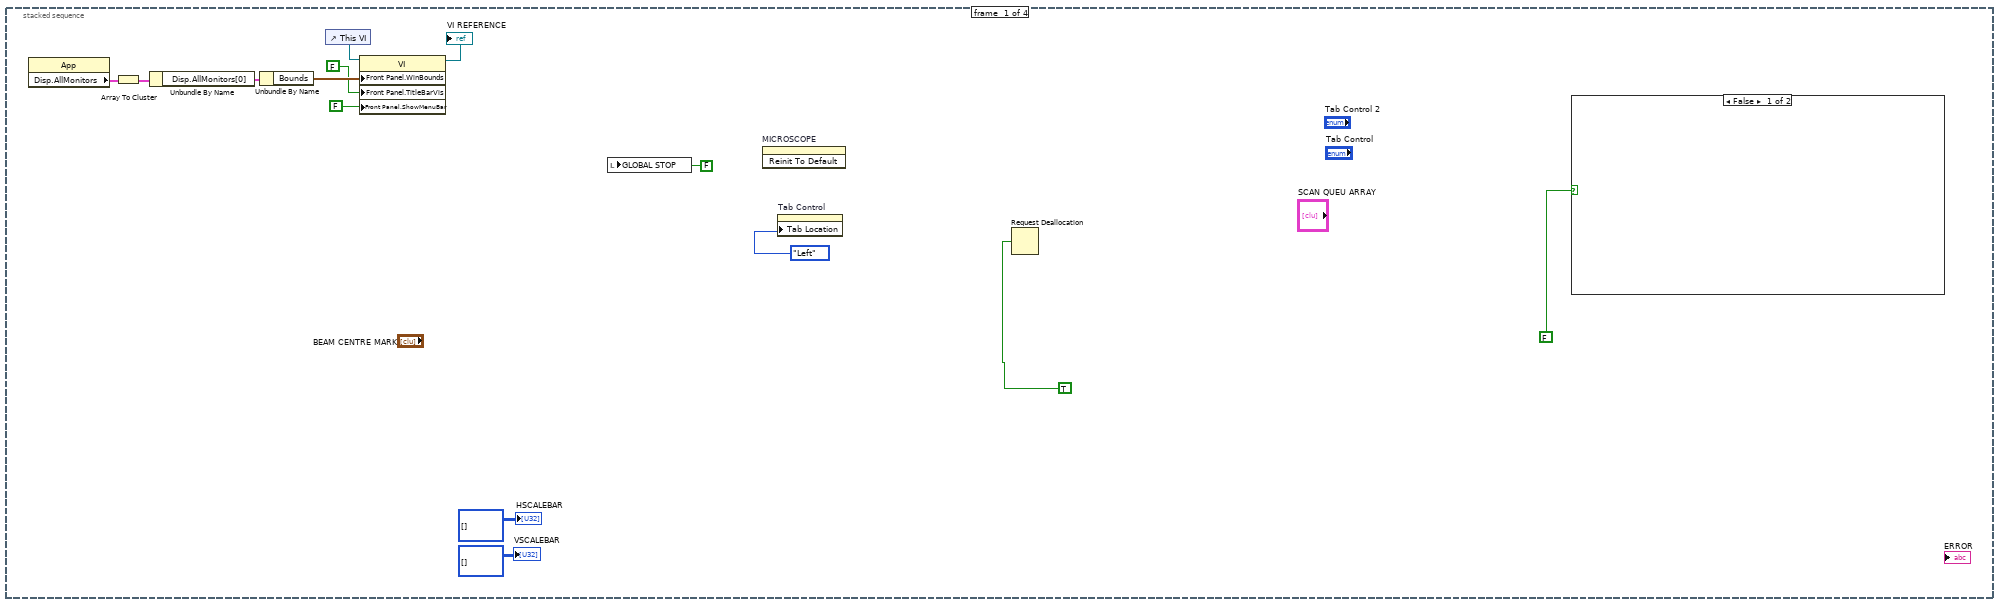
[diagram p2: hidden frame]
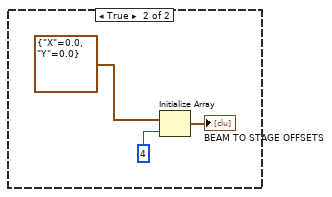
[diagram p3: hidden frame]
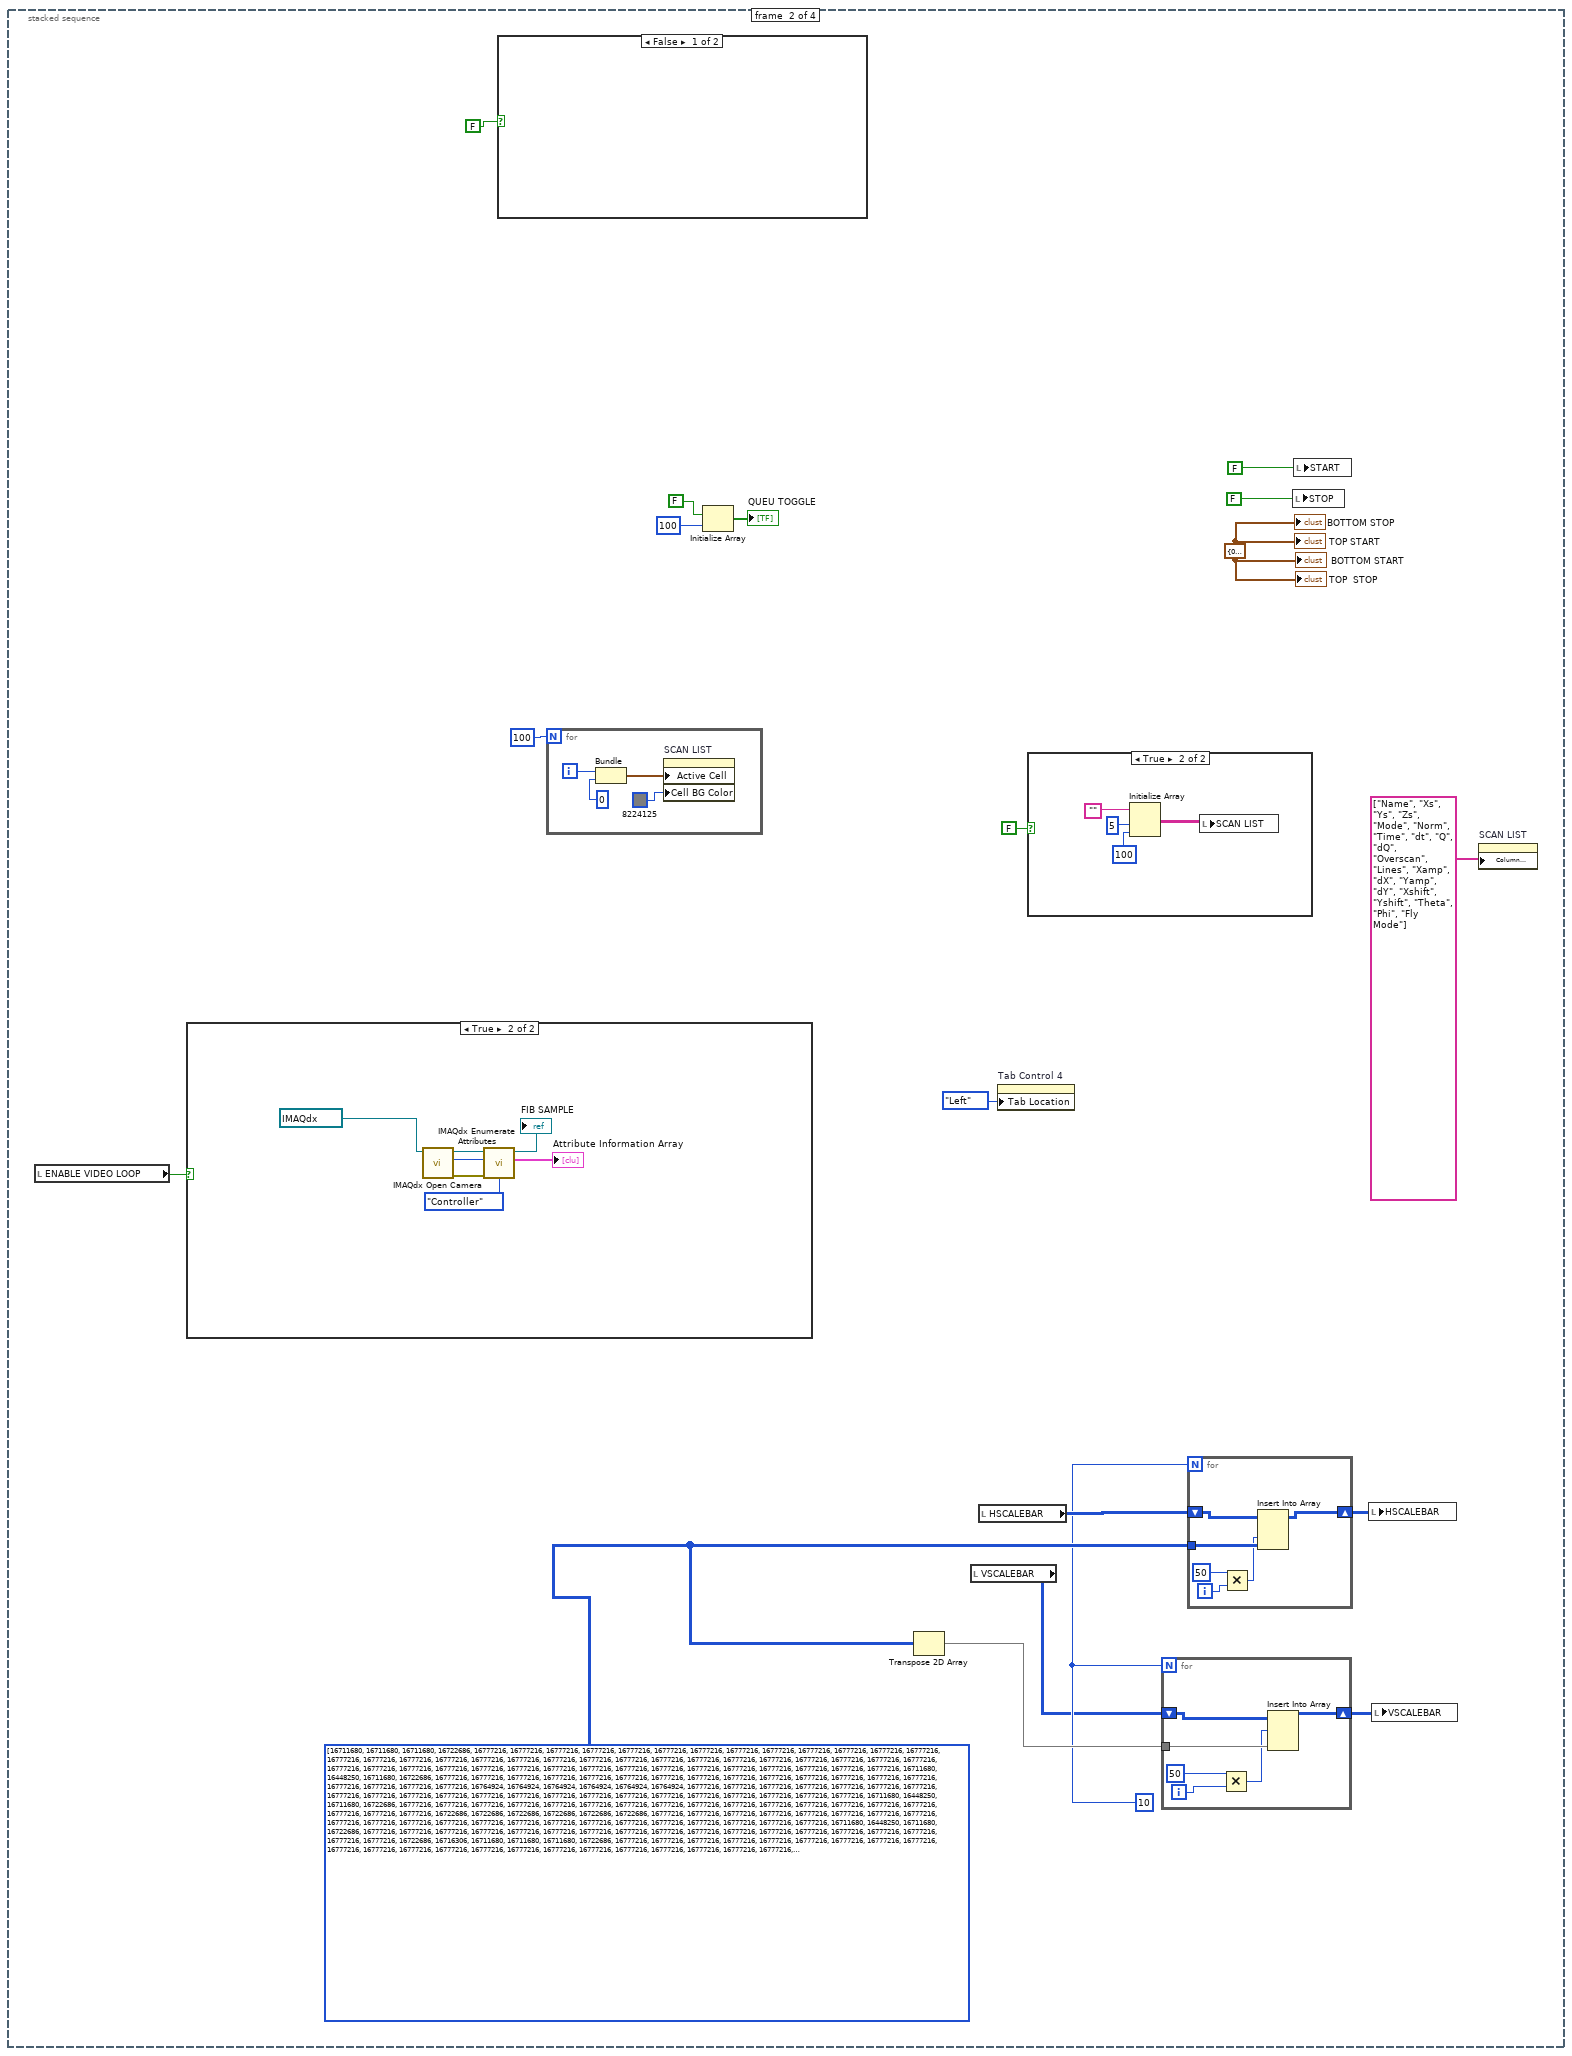
[diagram p4: hidden frame]
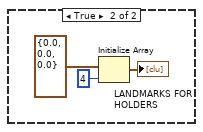
[diagram p6: hidden frame]
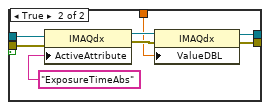
[diagram p9: hidden frame]
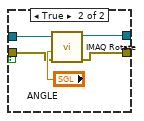
[diagram p12: hidden frame]
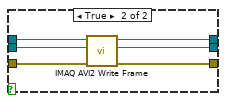
[diagram p15: hidden frame]
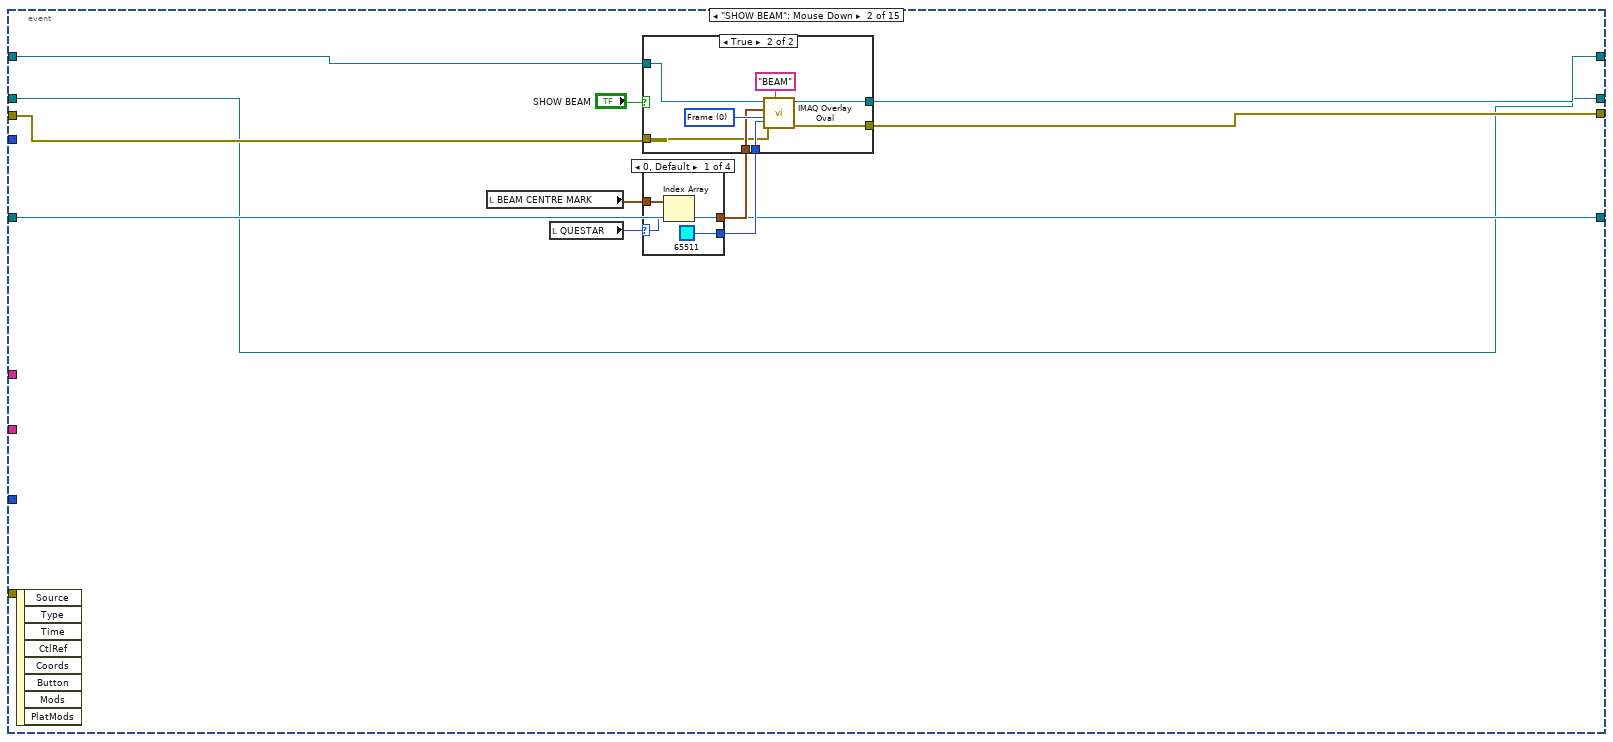
[diagram p16: hidden frame]
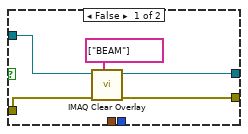
[diagram p17: hidden frame]
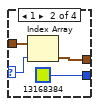
[diagram p18: hidden frame]
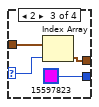
[diagram p19: hidden frame]
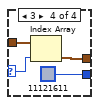
[diagram p20: hidden frame]
diagram:
  n1 = stacked-sequence {
    frame #0 {
      n2 = property class="App"() -> ("Disp.AllMonitors"=w11:T28)  [unwired: 2 in, 2 out]
      n3 = Array To Cluster(array=w11) -> (cluster=w10:T29)
      n4 = Unbundle By Name(w10) -> ("Disp.AllMonitors[0]"=w5:T30)
      n5 = Unbundle By Name(w5) -> ("Bounds"=w8:T31)
      n6 = control-ref of="This VI"() -> (w9:refnum<vi>)
      n7 = property class="VI"(reference=w9, "Front Panel.WinBounds"=w8, "Front Panel.TitleBarVis"=FALSE ("Front Panel Window:Title Bar Visible"), "Front Panel.ShowMenuBar"=FALSE ("Front Panel Window:Show Menu Bar")) -> (reference out=→"VI REFERENCE":refnum<vi>)  [unwired: 1 in, 1 out]
      n8 = local write "GLOBAL STOP"(FALSE ("GLOBAL STOP")) -> ()
      n9 = invoke on="MICROSCOPE" class="ImageControl" method="Reinit To Default"() -> ()  [unwired: 3 in, 3 out]
      n10 = property on="Tab Control" class="TabCtl (strict)"("Tab Location"=enum32{"Top", "Bottom", "Left", "Right"}."Left") -> ()  [unwired: 2 in, 2 out]
      n11 = Request Deallocation(TRUE ("flag")) -> ()
      n12 = case shown="False" FALSE {
        frame False {
        }
        frame True {
          n13 = Initialize Array(cluster{"X":dbl[unit], "Y":dbl[unit]} {"X"=0.0, "Y"=0.0}, 4 ("dimension size")) -> (→"BEAM TO STAGE OFFSETS":cluster{"X":dbl[unit], "Y":dbl[unit]}[])
        }
      }
      "HSCALEBAR" <- u32[][] [] ("SCALEBAR")
      "VSCALEBAR" <- u32[][] [] ("SCALEBAR")
    }
    frame #1 {
      w28 = T3 {"X"=0.0, "Y"=0.0, "Z"=0.0} ("TOP START")
      w32 = 10
      w34 = u32[][] [[16711680, 16711680, 16711680, 16722686, 16777216, 16777216, 16777216, 16777216, 16777216, 16777216, 16777216, 16777216, 16777216, 16777216, 16777216, 16777216, 16777216, 16777216, 16777216, 16777216, 16777216, 16777216, 16777216, 16777216, 16777216, 16777216, 16777216, 16777216, 16777216, 16777216, 16777216, 16777216, 16777216, 16777216, 16777216, 16777216, 16777216, 16777216, 16777216, 16777216, 16777216, 16777216, 16777216, 16777216, 16777216, 16777216, 16777216, 16777216, 16777216, 16777216], [16711680, 16448250, 16711680, 16722686, 16777216, 16777216, 16777216, 16777216, 16777216, 16777216, 16777216, 16777216, 16777216, 16777216, 16777216, 16777216, 16777216, 16777216, 16777216, 16777216, 16777216, 16777216, 16764924, 16764924, 16764924, 16764924, 16764924, 16764924, 16777216, 16777216, 16777216, 16777216, 16777216, 16777216, 16777216, 16777216, 16777216, 16777216, 16777216, 16777216, 16777216, 16777216, 16777216, 16777216, 16777216, 16777216, 16777216, 16777216, 16777216, 16777216], [16711680, 16448250, 16711680, 16722686, 16777216, 16777216, 16777216, 16777216, 16777216, 16777216, 16777216, 16777216, 16777216, 16777216, 16777216, 16777216, 16777216, 16777216, 16777216, 16777216, 16777216, 16777216, 16722686, 16722686, 16722686, 16722686, 16722686, 16722686, 16777216, 16777216, 16777216, 16777216, 16777216, 16777216, 16777216, 16777216, 16777216, 16777216, 16777216, 16777216, 16777216, 16777216, 16777216, 16777216, 16777216, 16777216, 16777216, 16777216, 16777216, 16777216], [16711680, 16448250, 16711680, 16722686, 16777216, 16777216, 16777216, 16777216, 16777216, 16777216, 16777216, 16777216, 16777216, 16777216, 16777216, 16777216, 16777216, 16777216, 16777216, 16777216, 16777216, 16777216, 16722686, 16716306, 16711680, 16711680, 16711680, 16722686, 16777216, 16777216, 16777216, 16777216, 16777216, 16777216, 16777216, 16777216, 16777216, 16777216, 16777216, 16777216, 16777216, 16777216, 16777216, 16777216, 16777216, 16777216, 16777216, 16777216, 16777216, 16777216], [16711680, 16448250, 16711680, 16722686, 16777216, 16777216, 16777216, 16777216, 16777216, 16777216, 16777216, 16777216, 16777216, 16777216, 16777216, 16777216, 16777216, 16777216, 16777216, 16777216, 16777216, 16777216, 16722686, 16716306, 16448250, 16448250, 16711680, 16722686, 16777216, 16777216, 16777216, 16777216, 16777216, 16777216, 16777216, 16777216, 16777216, 16777216, 16777216, 16777216, 16777216, 16777216, 16777216, 16777216, 16777216, 16777216, 16777216, 16777216, 16777216, 16777216], [16711680, 16448250, 16711680, 16722686, 16722686, 16722686, 16722686, 16722686, 16722686, 16722686, 16722686, 16722686, 16722686, 16722686, 16722686, 16722686, 16722686, 16722686, 16722686, 16722686, 16722686, 16722686, 16722686, 16711680, 16448250, 16448250, 16711680, 16722686, 16722686, 16722686, 16722686, 16722686, 16722686, 16722686, 16722686, 16722686, 16722686, 16722686, 16722686, 16722686, 16722686, 16722686, 16722686, 16722686, 16722686, 16722686, 16722686, 16722686, 16722686, 16722686], [16711680, 16448250, 16711680, 16711680, 16711680, 16716306, 16716306, 16716306, 16711680, 16711680, 16711680, 16711680, 16711680, 16711680, 16711680, 16711680, 16711680, 16711680, 16711680, 16711680, 16711680, 16711680, 16711680, 16711680, 16448250, 16448250, 16711680, 16711680, 16711680, 16711680, 16711680, 16711680, 16711680, 16711680, 16711680, 16711680, 16711680, 16711680, 16711680, 16711680, 16711680, 16711680, 16711680, 16711680, 16711680, 16711680, 16711680, 16711680, 16711680, 16711680], [16711680, 16448250, 16448250, 16448250, 16448250, 16448250, 16448250, 16448250, 16448250, 16448250, 16448250, 16448250, 16448250, 16448250, 16448250, 16448250, 16448250, 16448250, 16448250, 16448250, 16448250, 16448250, 16448250, 16448250, 16448250, 16448250, 16448250, 16448250, 16448250, 16448250, 16448250, 16448250, 16448250, 16448250, 16448250, 16448250, 16448250, 16448250, 16448250, 16448250, 16448250, 16448250, 16448250, 16448250, 16448250, 16448250, 16448250, 16448250, 16448250, 16448250], [16711680, 16448250, 16448250, 16448250, 16448250, 16448250, 16448250, 16448250, 16448250, 16448250, 16448250, 16448250, 16448250, 16448250, 16448250, 16448250, 16448250, 16448250, 16448250, 16448250, 16448250, 16448250, 16448250, 16448250, 16448250, 16448250, 16448250, 16448250, 16448250, 16448250, 16448250, 16448250, 16448250, 16448250, 16448250, 16448250, 16448250, 16448250, 16448250, 16448250, 16448250, 16448250, 16448250, 16448250, 16448250, 16448250, 16448250, 16448250, 16448250, 16448250], [16711680, 16448250, 16711680, 16716306, 16716306, 16716306, 16716306, 16716306, 16711680, 16711680, 16711680, 16711680, 16711680, 16711680, 16711680, 16711680, 16711680, 16711680, 16711680, 16711680, 16711680, 16711680, 16711680, 16711680, 16448250, 16448250, 16711680, 16711680, 16711680, 16711680, 16711680, 16711680, 16711680, 16711680, 16711680, 16711680, 16711680, 16711680, 16711680, 16711680, 16711680, 16711680, 16711680, 16711680, 16711680, 16711680, 16711680, 16711680, 16711680, 16711680], [16711680, 16448250, 16711680, 16722686, 16722686, 16722686, 16722686, 16722686, 16722686, 16722686, 16722686, 16722686, 16722686, 16722686, 16722686, 16722686, 16722686, 16722686, 16722686, 16722686, 16722686, 16722686, 16722686, 16711680, 16448250, 16448250, 16711680, 16722686, 16722686, 16722686, 16722686, 16722686, 16722686, 16722686, 16722686, 16722686, 16722686, 16722686, 16722686, 16722686, 16722686, 16722686, 16722686, 16722686, 16722686, 16722686, 16722686, 16722686, 16722686, 16722686], [16711680, 16448250, 16711680, 16722686, 16777216, 16777216, 16777216, 16777216, 16777216, 16777216, 16777216, 16777216, 16777216, 16777216, 16777216, 16777216, 16777216, 16777216, 16777216, 16777216, 16777216, 16777216, 16722686, 16711680, 16448250, 16448250, 16711680, 16722686, 16777216, 16777216, 16777216, 16777216, 16777216, 16777216, 16777216, 16777216, 16777216, 16777216, 16777216, 16777216, 16777216, 16777216, 16777216, 16777216, 16777216, 16777216, 16777216, 16777216, 16777216, 16777216], [16711680, 16448250, 16711680, 16722686, 16777216, 16777216, 16777216, 16777216, 16777216, 16777216, 16777216, 16777216, 16777216, 16777216, 16777216, 16777216, 16777216, 16777216, 16777216, 16777216, 16777216, 16777216, 16722686, 16711680, 16711680, 16711680, 16711680, 16722686, 16777216, 16777216, 16777216, 16777216, 16777216, 16777216, 16777216, 16777216, 16777216, 16777216, 16777216, 16777216, 16777216, 16777216, 16777216, 16777216, 16777216, 16777216, 16777216, 16777216, 16777216, 16777216], [16711680, 16448250, 16711680, 16722686, 16777216, 16777216, 16777216, 16777216, 16777216, 16777216, 16777216, 16777216, 16777216, 16777216, 16777216, 16777216, 16777216, 16777216, 16777216, 16777216, 16777216, 16777216, 16722686, 16722686, 16722686, 16722686, 16722686, 16722686, 16777216, 16777216, 16777216, 16777216, 16777216, 16777216, 16777216, 16777216, 16777216, 16777216, 16777216, 16777216, 16777216, 16777216, 16777216, 16777216, 16777216, 16777216, 16777216, 16777216, 16777216, 16777216], [16711680, 16448250, 16711680, 16722686, 16777216, 16777216, 16777216, 16777216, 16777216, 16777216, 16777216, 16777216, 16777216, 16777216, 16777216, 16777216, 16777216, 16777216, 16777216, 16777216, 16777216, 16777216, 16764924, 16764924, 16764924, 16764924, 16764924, 16764924, 16777216, 16777216, 16777216, 16777216, 16777216, 16777216, 16777216, 16777216, 16777216, 16777216, 16777216, 16777216, 16777216, 16777216, 16777216, 16777216, 16777216, 16777216, 16777216, 16777216, 16777216, 16777216], [16711680, 16448250, 16711680, 16722686, 16777216, 16777216, 16777216, 16777216, 16777216, 16777216, 16777216, 16777216, 16777216, 16777216, 16777216, 16777216, 16777216, 16777216, 16777216, 16777216, 16777216, 16777216, 16777216, 16777216, 16777216, 16777216, 16777216, 16777216, 16777216, 16777216, 16777216, 16777216, 16777216, 16777216, 16777216, 16777216, 16777216, 16777216, 16777216, 16777216, 16777216, 16777216, 16777216, 16777216, 16777216, 16777216, 16777216, 16777216, 16777216, 16777216], [16711680, 16711680, 16711680, 16722686, 16777216, 16777216, 16777216, 16777216, 16777216, 16777216, 16777216, 16777216, 16777216, 16777216, 16777216, 16777216, 16777216, 16777216, 16777216, 16777216, 16777216, 16777216, 16777216, 16777216, 16777216, 16777216, 16777216, 16777216, 16777216, 16777216, 16777216, 16777216, 16777216, 16777216, 16777216, 16777216, 16777216, 16777216, 16777216, 16777216, 16777216, 16777216, 16777216, 16777216, 16777216, 16777216, 16777216, 16777216, 16777216, 16777216], [16764924, 16764924, 16764924, 16764924, 16777216, 16777216, 16777216, 16777216, 16777216, 16777216, 16777216, 16777216, 16777216, 16777216, 16777216, 16777216, 16777216, 16777216, 16777216, 16777216, 16777216, 16777216, 16777216, 16777216, 16777216, 16777216, 16777216, 16777216, 16777216, 16777216, 16777216, 16777216, 16777216, 16777216, 16777216, 16777216, 16777216, 16777216, 16777216, 16777216, 16777216, 16777216, 16777216, 16777216, 16777216, 16777216, 16777216, 16777216, 16777216, 16777216]] ("Bitmap")
      n14 = local read "ENABLE VIDEO LOOP"() -> (w18:bool)
      n15 = case shown="True" w18 {
        frame False {
        }
        frame True {
          n16 = call <vilib>:"IMAQdx Open Camera.vi"("Camera Control Mode"=IMAQdx_Camera_Control_Mode."Controller", "Session In"=T8 "MAKO") -> ("error out"=w42:errorcluster, "Session Out"=w41:T8)  [unwired: 8 in]
          n17 = call <vilib>:"IMAQdx Enumerate Attributes.vi"("error in"=w42, "Session In"=w41) -> ("Attribute Information Array"=→"Attribute Information Array":T18, "Session Out"=→"FIB SAMPLE":T8)  [unwired: 7 in, 1 out]
        }
      }
      n18 = case shown="False" FALSE {
        frame False {
        }
        frame True {
          n19 = Initialize Array(T3 {"X"=0.0, "Y"=0.0, "Z"=0.0} ("APERTURE POSITION"), 4 ("dimension size")) -> (→"LANDMARKS FOR HOLDERS":T14)
        }
      }
      n20 = for {
        N: 100 -> [_]
        i -> [w45]
        n21 = Bundle(w45, 0) -> (w46:cluster{i32, i32})  [unwired: 1 in]
        n22 = property on="SCAN LIST" class="Tbl (strict)"("Active Cell"=w46, "Cell BG Color"=u32 8224125) -> ()  [unwired: 2 in, 2 out]
      }
      n23 = Initialize Array(FALSE, 100 ("dimension size")) -> (→"QUEU TOGGLE":bool[])
      n24 = Transpose 2D Array(2D array=w34) -> (transposed array=w33:u32[][])
      n25 = local read "VSCALEBAR"() -> (w31:u32[][])
      n26 = local read "HSCALEBAR"() -> (w36:u32[][])
      n27 = property on="Tab Control 4" class="TabCtl (strict)"("Tab Location"=enum32{"Top", "Bottom", "Left", "Right"}."Left") -> ()  [unwired: 2 in, 2 out]
      n28 = case shown="True" FALSE {
        frame False {
        }
        frame True {
          n29 = Initialize Array("", 5 ("dimension size"), 100 ("dimension size")) -> (w50:string[][])
          n30 = local write "SCAN LIST"(w50) -> ()
        }
      }
      n31 = for {
        N: w32 -> [_]
        shift-right: [w58] -> w30
        shift-left: w31 -> [w59]
        tunnel: w33 -> [w55]
        i -> [w57]
        n32 = Multiply(x=50, y=w57) -> (x*y=w54:i32)
        n33 = Insert Into Array(array=w59, index (row)=w54, new element=w55) -> (w58:u32[][])  [unwired: 1 in]
      }
      n34 = for {
        N: w32 -> [_]
        shift-right: [w64] -> w35
        shift-left: w36 -> [w65]
        tunnel: w34 -> [w61]
        i -> [w63]
        n35 = Multiply(x=50, y=w63) -> (x*y=w60:i32)
        n36 = Insert Into Array(array=w65, index (col)=w60, new element=w61) -> (w64:u32[][])  [unwired: 1 in]
      }
      n37 = local write "STOP"(FALSE ("STOP")) -> ()
      n38 = local write "START"(FALSE ("START")) -> ()
      n39 = local write "HSCALEBAR"(w35) -> ()
      n40 = local write "VSCALEBAR"(w30) -> ()
      n41 = property on="SCAN LIST" class="Tbl (strict)"("Column Headers[]"=string[] ["Name", "Xs", "Ys", "Zs", "Mode", "Norm", "Time", "dt", "Q", "dQ", "Overscan", "Lines", "Xamp", "dX", "Yamp", "dY", "Xshift", "Yshift", "Theta", "Phi", "Fly Mode"] ("Column Header Strings[]")) -> ()  [unwired: 2 in, 2 out]
      "TOP START" <- w28
      "BOTTOM START" <- w28
      "TOP  STOP" <- w28
      "BOTTOM STOP" <- w28
    }
    frame #2 {
      n42 = case shown="True" "ENABLE VIDEO LOOP" {
        frame False {
        }
        frame True {
          w78 = 2.0
          w86 = u32[][] [[16777216, 16777216, 16777216, 16777216, 16777216, 16777216, 16777216, 16777216, 16777216, 16777216, 16777216, 12189440, 16777216, 16777216, 16777216, 16777216, 16777216, 16777216, 16777216, 16777216, 16777216, 16777216, 16777216], [16777216, 16777216, 16777216, 16777216, 16777216, 16777216, 16777216, 16777216, 16777216, 16777216, 16777216, 12189440, 16777216, 16777216, 16777216, 16777216, 16777216, 16777216, 16777216, 16777216, 16777216, 16777216, 16777216], [16777216, 16777216, 16777216, 16777216, 16777216, 16777216, 16777216, 16777216, 16777216, 16777216, 15859456, 12189440, 15859456, 16777216, 16777216, 16777216, 16777216, 16777216, 16777216, 16777216, 16777216, 16777216, 16777216], [16777216, 16777216, 16777216, 16777216, 16777216, 16777216, 16777216, 16777216, 16777216, 16777216, 15859456, 12189440, 15859456, 16777216, 16777216, 16777216, 16777216, 16777216, 16777216, 16777216, 16777216, 16777216, 16777216], [16777216, 16777216, 16777216, 16777216, 16777216, 16777216, 16777216, 16777216, 16777216, 16777216, 15859456, 12189440, 15859456, 16777216, 16777216, 16777216, 16777216, 16777216, 16777216, 16777216, 16777216, 16777216, 16777216], [16777216, 16777216, 16777216, 16777216, 16777216, 16777216, 16777216, 16777216, 16777216, 16777216, 15859456, 12189440, 15859456, 16777216, 16777216, 16777216, 16777216, 16777216, 16777216, 16777216, 16777216, 16777216, 16777216], [16777216, 16777216, 16777216, 16777216, 16777216, 16777216, 16777216, 16777216, 16777216, 16777216, 15859456, 12189440, 15859456, 16777216, 16777216, 16777216, 16777216, 16777216, 16777216, 16777216, 16777216, 16777216, 16777216], [16777216, 16777216, 16777216, 16777216, 16777216, 16777216, 16777216, 16777216, 16777216, 16777216, 16777216, 12189440, 16777216, 16777216, 16777216, 16777216, 16777216, 16777216, 16777216, 16777216, 16777216, 16777216, 16777216], [16777216, 16777216, 16777216, 16777216, 16777216, 16777216, 16777216, 16777216, 12189440, 16777216, 16777216, 12189440, 16777216, 16777216, 12189440, 16777216, 16777216, 16777216, 16777216, 16777216, 16777216, 16777216, 16777216], [16777216, 16777216, 16777216, 16777216, 16777216, 16777216, 16777216, 16777216, 16777216, 12189440, 16777216, 12189440, 16777216, 12189440, 16777216, 16777216, 16777216, 16777216, 16777216, 16777216, 16777216, 16777216, 16777216], [16777216, 16777216, 15859456, 15859456, 15859456, 15859456, 15859456, 16777216, 16777216, 16777216, 16777216, 12189440, 16777216, 16777216, 16777216, 16777216, 15859456, 15859456, 15859456, 15859456, 15859456, 16777216, 16777216], [12189440, 12189440, 12189440, 12189440, 12189440, 12189440, 12189440, 12189440, 12189440, 12189440, 12189440, 12189440, 12189440, 12189440, 12189440, 12189440, 12189440, 12189440, 12189440, 12189440, 12189440, 12189440, 12189440], [16777216, 16777216, 15859456, 15859456, 15859456, 15859456, 15859456, 16777216, 16777216, 16777216, 16777216, 12189440, 16777216, 16777216, 16777216, 16777216, 15859456, 15859456, 15859456, 15859456, 15859456, 16777216, 16777216], [16777216, 16777216, 16777216, 16777216, 16777216, 16777216, 16777216, 16777216, 16777216, 12189440, 16777216, 12189440, 16777216, 12189440, 16777216, 16777216, 16777216, 16777216, 16777216, 16777216, 16777216, 16777216, 16777216], [16777216, 16777216, 16777216, 16777216, 16777216, 16777216, 16777216, 16777216, 12189440, 16777216, 16777216, 12189440, 16777216, 16777216, 12189440, 16777216, 16777216, 16777216, 16777216, 16777216, 16777216, 16777216, 16777216], [16777216, 16777216, 16777216, 16777216, 16777216, 16777216, 16777216, 16777216, 16777216, 16777216, 16777216, 12189440, 16777216, 16777216, 16777216, 16777216, 16777216, 16777216, 16777216, 16777216, 16777216, 16777216, 16777216], [16777216, 16777216, 16777216, 16777216, 16777216, 16777216, 16777216, 16777216, 16777216, 16777216, 15859456, 12189440, 15859456, 16777216, 16777216, 16777216, 16777216, 16777216, 16777216, 16777216, 16777216, 16777216, 16777216], [16777216, 16777216, 16777216, 16777216, 16777216, 16777216, 16777216, 16777216, 16777216, 16777216, 15859456, 12189440, 15859456, 16777216, 16777216, 16777216, 16777216, 16777216, 16777216, 16777216, 16777216, 16777216, 16777216], [16777216, 16777216, 16777216, 16777216, 16777216, 16777216, 16777216, 16777216, 16777216, 16777216, 15859456, 12189440, 15859456, 16777216, 16777216, 16777216, 16777216, 16777216, 16777216, 16777216, 16777216, 16777216, 16777216], [16777216, 16777216, 16777216, 16777216, 16777216, 16777216, 16777216, 16777216, 16777216, 16777216, 15859456, 12189440, 15859456, 16777216, 16777216, 16777216, 16777216, 16777216, 16777216, 16777216, 16777216, 16777216, 16777216], [16777216, 16777216, 16777216, 16777216, 16777216, 16777216, 16777216, 16777216, 16777216, 16777216, 15859456, 12189440, 15859456, 16777216, 16777216, 16777216, 16777216, 16777216, 16777216, 16777216, 16777216, 16777216, 16777216], [16777216, 16777216, 16777216, 16777216, 16777216, 16777216, 16777216, 16777216, 16777216, 16777216, 16777216, 12189440, 16777216, 16777216, 16777216, 16777216, 16777216, 16777216, 16777216, 16777216, 16777216, 16777216, 16777216], [16777216, 16777216, 16777216, 16777216, 16777216, 16777216, 16777216, 16777216, 16777216, 16777216, 16777216, 12189440, 16777216, 16777216, 16777216, 16777216, 16777216, 16777216, 16777216, 16777216, 16777216, 16777216, 16777216]] ("Bitmap")
          w91 = T32 4 items=["Grayscale (U8)", "Grayscale (I16)", "Grayscale (SGL)", "Complex (CSG)", "RGB (U32)", "HSL (U32)", "RGB (U64)", "Grayscale (U16)"] ("Image Type")
          w103 = 2.0
          w112 = sgl 0.95 ("x")
          # "VIDEO EVENT LOOP"
          n43 = local read "FIB SAMPLE"() -> (w131:T8)
          n44 = property class="IMAQdx"(reference=w131) -> (reference out=w99:T8, "ActualPeakBandwidth"=→"ActualPeakBandwidth":dbl)  [unwired: 1 in, 1 out]
          n45 = property class="IMAQdx"(reference=w99) -> (reference out=w152:T8, error out=w151:errorcluster, "DisplayName"=→"DisplayName":string)  [unwired: 1 in]
          n46 = property class="IMAQdx"(reference=w152, error in=w151) -> (reference out=w83:T8, error out=w82:errorcluster, "IPAddress"=→"IP ADDRESS":string, "Width"=w77:u32, "Height"=w76:u32)
          "IMAGE XPIXELS" <- w77
          "IMAGE YPIXELS" <- w76
          n47 = Multiply(x=w77, y=w112) -> (x*y=w110:sgl)
          n48 = Multiply(x=w76, y=w112) -> (x*y=w111:sgl)
          n49 = To Double Precision Float(number=w77) -> (double precision float=w80:dbl)
          n50 = To Double Precision Float(number=w76) -> (double precision float=w79:dbl)
          n51 = Bundle(w110, w111) -> ()  [unwired: 1 in, 1 out]
          n52 = property class="IMAQdx"(reference=w83, error in=w82, "ActiveAttribute"="GainAuto") -> (reference out=w117:T8, error out=w116:errorcluster)
          n53 = Divide(x=w79, y=w78) -> (x/y=→"IMAGE YCENTRE":dbl)
          n54 = Divide(x=w80, y=w78) -> (x/y=→"IMAGE XCENTRE":dbl)
          n55 = property class="IMAQdx"(reference=w117, error in=w116, "ValueU32"="GAIN METHOD") -> (reference out=w115:T8, error out=w114:errorcluster)
          n56 = case shown="True" FALSE {
            frame False {
            }
            frame True {
              n57 = property on="MICROSCOPE" class="ImageControl"() -> ("Image Area Size"=→"Image Area:Size:All Elements":cluster{"Width":u32, "Height":u32})  [unwired: 2 in, 2 out]
            }
          }
          n58 = property class="IMAQdx"(reference=w115, error in=w114, "ActiveAttribute"="GainRaw") -> (reference out=w121:T8, error out=w120:errorcluster)
          n59 = property class="IMAQdx"(reference=w121, error in=w120, "ValueDBL"="GAIN") -> (reference out=w146:T8, error out=w145:errorcluster)
          n60 = property class="IMAQdx"(reference=w146, error in=w145, "ActiveAttribute"="ExposureAuto") -> (reference out=w144:T8, error out=w143:errorcluster)
          n61 = property class="IMAQdx"(reference=w144, error in=w143, "ValueU32"=u32 1) -> (reference out=w141:T8, error out=w140:errorcluster)
          n62 = case shown="0, Default" "CONFIGS" {
            tunnel: [10.0 ("EXPOSURE TIME") 20.0 ("EXPOSURE TIME") 5.0 ("EXPOSURE TIME")] -> w147
            tunnel: "EXPOSURE" -> [_ _ _]
            frame 0, Default {
            }
            frame 1 {
            }
            frame 2 {
            }
          }
          n63 = local write "EXPOSURE"(w147) -> ()
          n64 = local read "IMAGE YPIXELS"() -> (w104:u32)
          n65 = local read "IMAGE XPIXELS"() -> (w105:u32)
          n66 = Multiply(x=1000.0, y=w147) -> (x*y=w139:dbl)
          n67 = case shown="False" FALSE {
            tunnel: w141 -> [w164 w171]
            tunnel: w140 -> [w163 w170]
            tunnel: w139 -> [_ w167]
            tunnel: [w164 w166] -> w135
            tunnel: [w163 w165] -> w134
            frame False {
            }
            frame True {
              n68 = property class="IMAQdx"(reference=w171, error in=w170, "ActiveAttribute"="ExposureTimeAbs") -> (reference out=w169:T8, error out=w168:errorcluster)
              n69 = property class="IMAQdx"(reference=w169, error in=w168, "ValueDBL"=w167) -> (reference out=w166:T8, error out=w165:errorcluster)
            }
          }
          n70 = property class="IMAQdx"(reference=w135, error in=w134, "ActiveAttribute"="GainAuto") -> (reference out=w137:T8, error out=w136:errorcluster)
          n71 = property class="IMAQdx"(reference=w137, error in=w136, "ValueU32"=u32 2) -> (reference out=w133:T8, error out=w132:errorcluster)
          n72 = call <vilib>:"IMAQdx Configure Grab.vi"("error in"=w132, "Session In"=w133) -> ("error out"=w160:errorcluster, "Session Out"=w158:T8)  [unwired: 8 in]
          n73 = Divide(x=w105, y=w103) -> (x/y=w102:dbl)
          n74 = Divide(x=w104, y=w103) -> (x/y=w101:dbl)
          n75 = To Long Integer(number=w102) -> (32bit integer=w97:i32)
          n76 = To Long Integer(number=w101) -> (32bit integer=w95:i32)
          n77 = case shown="True" FALSE {
            tunnel: w158 -> [w629 w633]
            tunnel: [w629 w632] -> w72
            tunnel: w160 -> [w628 w631]
            tunnel: [w628 w630] -> w71
            frame False {
            }
            frame True {
              n78 = call <vilib>:"IMAQdx Read Attributes.vi"("error in"=w631, "Session In"=w633) -> ("error out"=w630:errorcluster, "Session Out"=w632:T8)  [unwired: 8 in]
            }
          }
          n79 = Subtract(x=w97, y=3) -> (x-y=w93:i32)
          n80 = Subtract(x=w95, y=2) -> (x-y=w94:i32)
          n81 = local read "Attribute Information Array"() -> (w130:T18)
          n82 = Index Array(array=w130, index #1=127 ("index"), index #2=128 ("index")) -> (element #1=w128:T33, element #2=w125:T33)
          n83 = Bundle(w93, w94) -> (w89:cluster{i32, i32})  [unwired: 1 in]
          "CENTRE CAMERA FOV" <- w89
          n84 = call "IMAQ Create"("Image Name"="TARGET", "Image Type"=w91, "error in (no error)"=w71) -> ("New Image"=w88:T21, "error out"=w81:errorcluster)  [unwired: 2 in]
          n85 = Unbundle(w128) -> ("Attribute Name"=w127:string)  [unwired: 3 out]
          n86 = Unbundle(w125) -> ("Attribute Name"=w124:string)  [unwired: 3 out]
          n87 = call "IMAQ AVI2 Create"("Quality"=1, "AVI Path"="AVI Path") -> ("error out"=w107:errorcluster, "AVI Refnum"=w106:T34)  [unwired: 8 in]
          n88 = call "IMAQ Overlay Bitmap"("Group"="FEATURES", "error in (no error)"=w81, "Bitmap"=w86, "Top Left Point"=w89, "Image"=w88) -> ("error out"=w85:errorcluster, "Image Out"=w73:T21)  [unwired: 5 in]
          n89 = call <vilib>:"IMAQdx Start Acquisition.vi"("error in"=w71, "Session In"=w72) -> ("Session Out"=w70:T8)  [unwired: 8 in, 1 out]
          n90 = while {
            tunnel: [w188] -> w162
            tunnel: w85 -> [w175]
            shift-right: [w187] -> w161
            shift-left: w70 -> [w176]
            tunnel: w127 -> [w186]
            tunnel: w124 -> [w185]
            tunnel: w107 -> [w183]
            shift-right: [w182] -> w87
            shift-left: w106 -> [w184]
            shift-right: [w180] -> w100
            shift-left: w73 -> [w181]
            tunnel: w86 -> [w177]
            i -> [w179]
            stop <- w174 stop-if-true
            n91 = event shown="[0] Timeout" {
              selector: _ -> [_ _ _ _ _ _ _ _ _ _ _ _ _ _ _]
              dyn-events: _ -> [_ _ _ _ _ _ _ _ _ _ _ _ _ _ _]
              timeout: 10 -> [_ _ _ _ _ _ _ _ _ _ _ _ _ _ _]
              tunnel: [w202 w270 w307 w359 w387 w417 w421 w434 w468 w505 w529 w546 w550 _ w618] -> w188
              tunnel: [w199 w267 w311 w363 w389 w418 w429 w435 w484 w506 w530 w547 w551 w566 w620] -> w187
              tunnel: w181 -> [w196 w273 w310 w362 w386 w420 w431 w437 w472 _ w536 w538 w549 w565 w619]
              tunnel: w176 -> [w197 w267 w311 w363 w389 w418 w429 w435 w484 w526 w532 w541 w563 w566 w620]
              tunnel: w175 -> [w201 w272 w309 w361 w385 w417 w422 w434 w470 w525 w531 w540 w562 _ w618]
              tunnel: [w189 w271 w308 w360 w388 w419 w426 w436 w469 _ w536 w538 w549 w565 w619] -> w180
              tunnel: w186 -> [_ _ _ _ _ _ _ _ _ _ _ _ _ _ _]
              tunnel: w185 -> [_ _ _ _ _ _ _ _ _ _ _ _ _ _ _]
              tunnel: w184 -> [w218 w268 w312 w364 w390 w416 w430 w432 w474 w499 w527 w537 w558 w564 w597]
              tunnel: w183 -> [_ _ _ _ _ _ _ _ _ _ _ _ _ _ _]
              tunnel: [w203 w268 w312 w364 w390 w416 w430 w432 w474 w499 w527 w537 w558 w564 w597] -> w182
              tunnel: w179 -> [_ _ _ _ _ _ _ _ _ _ _ _ _ _ _]
              tunnel: w177 -> [_ _ _ _ _ w415 _ _ _ _ _ _ _ _ _]
              event Timeout {
                n92 = event-data() -> ()  [unwired: 1 in, 2 out]
                n93 = local read "ZOOM CALIBRATION FACTORS"() -> (w223:dbl[])
                n94 = call <vilib>:"IMAQdx Get Image2.vi"("Timeout (ms)"=5000, "Buffer Number Mode (Next)"=IMAQdx_Buffer_Number_Mode."Next", "error in"=w201, "Image In"=w196, "Session In"=w197) -> ("error out"=w200:errorcluster, "Image Out"=w198:T21, "Session Out"=w199:T8)  [unwired: 3 in, 1 out]
                n95 = property on="ANGLE" class="DigNum (strict)"("Visible"="ROTATE VIEW") -> ()  [unwired: 2 in, 2 out]
                n96 = Index Array(array=w223, index="QUESTAR") -> (element=w213:dbl)
                n97 = case shown="False" "ROTATE VIEW" {
                  tunnel: w198 -> [w237 w241]
                  tunnel: w200 -> [w236 w240]
                  tunnel: [w236 w239] -> w208
                  tunnel: [w237 w238] -> w207
                  frame False {
                  }
                  frame True {
                    n98 = call "IMAQ Rotate"("error in (no error)"=w240, "Angle (degrees)"="ANGLE", "Image Src"=w241) -> ("error out"=w239:errorcluster, "Image Dst Out"=w238:T21)  [unwired: 7 in]
                  }
                }
                n99 = local write "CALIBRATION FACTOR"(w213) -> ()
                n100 = case shown="True" "SYMMETRY" {
                  tunnel: w207 -> [w251 w256]
                  tunnel: w208 -> [w250 w255]
                  tunnel: "IMAGE SYMMETRY" -> [_ w254]
                  tunnel: [w251 w253] -> w210
                  tunnel: [w250 w252] -> w209
                  frame False {
                  }
                  frame True {
                    n101 = call "IMAQ Symmetry"("error in (no error)"=w255, "Type of Symmetry"=w254, "Image Src"=w256) -> ("error out"=w252:errorcluster, "Image Dst Out"=w253:T21)  [unwired: 2 in]
                  }
                }
                n102 = Bundle("CALI FACTOR"=w213, "CALI FACTOR"=w213, "Unit"=Image_Unit."Micrometer") -> (w212:T35)  [unwired: 1 in]
                n103 = property on="MICROSCOPE" class="ImageControl"() -> ("ROI"=w220:T4)  [unwired: 2 in, 2 out]
                n104 = Unbundle By Name(w220) -> ("Contours"=→"Contours":T19)
                n105 = case shown="True" "USE CALIBRATION" {
                  tunnel: [w244 w248] -> w216
                  tunnel: w210 -> [w244 w249]
                  tunnel: [w243 w247] -> w215
                  tunnel: w209 -> [w243 w246]
                  tunnel: w212 -> [_ w245]
                  frame False {
                  }
                  frame True {
                    n106 = call "IMAQ Set Simple Calibration2"("error in (no error)"=w246, "Pixel Distances"=w245, "Image"=w249) -> ("error out"=w247:errorcluster, "Calibration Template Image"=w248:T21)  [unwired: 7 in]
                  }
                }
                n107 = case shown="False" "RECORD AVI VIDEO" {
                  tunnel: w218 -> [w259 w265]
                  tunnel: [w259 w264] -> w193
                  tunnel: w216 -> [w258 w263]
                  tunnel: [w258 w260] -> w192
                  tunnel: [w257 w262] -> w194
                  tunnel: w215 -> [w257 w261]
                  frame False {
                  }
                  frame True {
                    n108 = call "IMAQ AVI2 Write Frame"("error in (no error)"=w261, "Image"=w263, "AVI Refnum"=w265) -> ("error out"=w262:errorcluster, "Image Out (duplicate)"=w260:T21, "AVI Refnum (duplicate)"=w264:T34)  [unwired: 6 in]
                  }
                }
                n109 = property on="BRIGHT,CONT,GAMMA" class="Clust (strict)"("Visible"="REFLECTIVITY") -> ()  [unwired: 2 in, 2 out]
                n110 = case shown="True" "REFLECTIVITY" {
                  tunnel: w192 -> [w226 w231]
                  tunnel: [w226 w233] -> w189
                  tunnel: "BRIGHT,CONT,GAMMA" -> [_ w232]
                  tunnel: w193 -> [w225 w230]
                  tunnel: [w225 w230] -> w203
                  tunnel: w194 -> [w224 w229]
                  tunnel: [w224 w227] -> w202
                  frame False {
                  }
                  frame True {
                    w235 = T32 0 items=["Grayscale (U8)", "Grayscale (I16)", "Grayscale (SGL)", "Complex (CSG)", "RGB (U32)", "HSL (U32)", "RGB (U64)", "Grayscale (U16)"] ("Image Type")
                    n111 = call "IMAQ Cast Image"("Image Type"=w235, "error in (no error)"=w229, "Image Src"=w231) -> ("error out"=w228:errorcluster, "Image Dst Out"=w234:T21)  [unwired: 7 in]
                    n112 = call "IMAQ BCGLookup"("Image Src"=w234, "BCG Values"=w232, "error in (no error)"=w228) -> ("Image Dst Out"=w233:T21, "error out"=w227:errorcluster)  [unwired: 4 in]
                  }
                }
                "MICROSCOPE" <- w189
              }
              event "SHOW BEAM": Mouse Down {
                n113 = event-data() -> ()  [unwired: 1 in, 8 out]
                n114 = local read "BEAM CENTRE MARK"() -> (w275:cluster{"L":i32, "T":i32, "R":i32, "B":i32}[])
                n115 = local read "QUESTAR"() -> (w266:i32)
                n116 = case shown="0, Default" w266 {
                  selector: w266 -> [w291 w295 w300 w303]
                  tunnel: [u32 65511 ("Color") u32 13168384 ("Color") u32 15597823 ("Color") u32 11121611 ("Color")] -> w276
                  tunnel: w275 -> [w292 w296 w299 w304]
                  tunnel: [w290 w294 w298 w302] -> w274
                  frame 0, Default {
                    n117 = Index Array(array=w292, index=w291) -> (element=w290:cluster{"L":i32, "T":i32, "R":i32, "B":i32})
                  }
                  frame 1 {
                    n118 = Index Array(array=w296, index=w295) -> (element=w294:cluster{"L":i32, "T":i32, "R":i32, "B":i32})
                  }
                  frame 2 {
                    n119 = Index Array(array=w299, index=w300) -> (element=w298:cluster{"L":i32, "T":i32, "R":i32, "B":i32})
                  }
                  frame 3 {
                    n120 = Index Array(array=w304, index=w303) -> (element=w302:cluster{"L":i32, "T":i32, "R":i32, "B":i32})
                  }
                }
                n121 = case shown="True" "SHOW BEAM" {
                  tunnel: [w280 w289] -> w271
                  tunnel: w276 -> [_ w287]
                  tunnel: w274 -> [_ w286]
                  tunnel: [w279 w285] -> w270
                  tunnel: w273 -> [w281 w283]
                  tunnel: w272 -> [w278 w282]
                  frame False {
                    n122 = call "IMAQ Clear Overlay"("Groups"=string[] ["BEAM"], "error in (no error)"=w278, "Image"=w281) -> ("error out"=w279:errorcluster, "Image Out"=w280:T21)  [unwired: 7 in]
                  }
                  frame True {
                    w288 = u32 0 items=["Frame", "Fill"] ("Drawing Mode (Frame)")
                    n123 = call "IMAQ Overlay Oval"("Color"=w287, "Group"="BEAM", "error in (no error)"=w282, "Drawing Mode (Frame)"=w288, "Bounding Rectangle"=w286, "Image"=w283) -> ("error out"=w285:errorcluster, "Image Out"=w289:T21)  [unwired: 4 in]
                  }
                }
              }
              event "SHOW POSITION": Mouse Down {
                n124 = event-data() -> ()  [unwired: 1 in, 8 out]
                n125 = local read "SHOW POSITION"() -> (w306:bool)
                n126 = case shown="True" w306 {
                  tunnel: w310 -> [w317 w321]
                  tunnel: [w316 w320] -> w308
                  tunnel: w309 -> [w314 w319]
                  tunnel: [w313 w318] -> w307
                  frame False {
                    n127 = call "IMAQ Clear Overlay"("Groups"=string[] ["SCAN POSITION"], "error in (no error)"=w314, "Image"=w317) -> ("error out"=w313:errorcluster, "Image Out"=w316:T21)  [unwired: 7 in]
                  }
                  frame True {
                    n128 = stacked-sequence {
                      tunnel: w321 -> [_ w338]
                      tunnel: [_ w332] -> w320
                      tunnel: w319 -> [_ w327]
                      tunnel: [_ w326] -> w318
                      frame #0 {
                        n129 = Wait (ms)(milliseconds to wait=u32 150 ("millisecond timer value")) -> ()  [unwired: 1 out]
                      }
                      frame #1 {
                        n130 = Number To Fractional String(number=0.0, precision (6)=i16 4) -> (F-format string=w336:string)  [unwired: 2 in]
                        n131 = Number To Fractional String(number=0.0, precision (6)=i16 4) -> (F-format string=w337:string)  [unwired: 2 in]
                        n132 = call <vilib>:"Space Constant.vi"() -> ("String"=w335:string)
                        n133 = Concatenate Strings(w337, w335, w336) -> (w334:string)
                        n134 = call "IMAQ Overlay Text"("BG Color (Transparent)"=u32 16747264, "Group"="SCAN POSITION", "Font, Size & Style"=T25 {"Desired Font (Application)"=enum."Application Font", "[User-specified Font]"={"Font Name"="", "Size"=64, "Strikeout?"=FALSE, "Italic?"=FALSE, "Underline?"=FALSE, "Outline?"=FALSE, "Shadow?"=FALSE, "Bold?"=FALSE, "Rotation Angle"=0.0}, "Horizontal Alignment"=1, "Vertical Alignment"=2}, "error in (no error)"=w327, "String"=w334, "Origin"=cluster{"X":i32, "Y":i32} {"X"=0, "Y"=0}, "Image"=w338) -> ("error out"=w326:errorcluster, "Image Out"=w332:T21)  [unwired: 3 in]
                      }
                    }
                  }
                }
              }
              event "SET FIDUCIAL 1", "SET FIDUCIAL 2": Mouse Down {
                n135 = event-data() -> ()  [unwired: 1 in, 8 out]
                n136 = local read "SET FIDUCIAL 1"() -> (w358:bool)
                n137 = case shown="True" w358 {
                  tunnel: ["2 = " "1 = "] -> w357
                  tunnel: [w365 w367] -> w344
                  frame False {
                    n138 = local read "REF#2"() -> (w365:T3)
                  }
                  frame True {
                    n139 = local read "REF#1"() -> (w367:T3)
                  }
                }
                n140 = Unbundle(w344) -> ("X"=w356:dbl[unit], "Y"=w354:dbl[unit])  [unwired: 1 out]
                n141 = node(w356) -> (w355:dbl)
                n142 = node(w354) -> (w353:dbl)
                n143 = Number To Fractional String(number=w353, precision (6)=i16 4) -> (F-format string=w351:string)  [unwired: 2 in]
                n144 = Number To Fractional String(number=w355, precision (6)=i16 4) -> (F-format string=w352:string)  [unwired: 2 in]
                n145 = call <vilib>:"Space Constant.vi"() -> ("String"=w350:string)
                n146 = Concatenate Strings(w352, w350, w351) -> (w342:string)
                n147 = Concatenate Strings("REF" ("Group"), w357, w342) -> (w341:string)
                n148 = call "IMAQ Overlay Text"("BG Color (Transparent)"=u32 16777216, "Group"="FIDUCIALS", "Text Color (black)"=u32 16496895, "Font, Size & Style"=T25 {"Desired Font (Application)"=enum."Application Font", "[User-specified Font]"={"Font Name"="", "Size"=86, "Strikeout?"=FALSE, "Italic?"=FALSE, "Underline?"=FALSE, "Outline?"=FALSE, "Shadow?"=FALSE, "Bold?"=FALSE, "Rotation Angle"=0.0}, "Horizontal Alignment"=0, "Vertical Alignment"=2}, "error in (no error)"=w361, "String"=w341, "Origin"=cluster{"X":i32, "Y":i32} {"X"=0, "Y"=0}, "Image"=w362) -> ("error out"=w359:errorcluster, "Image Out"=w360:T21)  [unwired: 2 in]
              }
              event "SHOW SCALE BAR": Mouse Down {
                n149 = event-data() -> ()  [unwired: 1 in, 8 out]
                n150 = local read "ZOOM CALIBRATION FACTORS"() -> (w373:dbl[])
                n151 = local read "QUESTAR"() -> (w372:i32)
                n152 = Index Array(array=w373, index=w372) -> (element=w371:dbl)
                n153 = Multiply(x=500.0, y=w371) -> (x*y=w376:dbl)
                n154 = Divide(x=w376, y=1000.0) -> (x/y=w374:dbl)
                n155 = Number To Fractional String(number=w374, width (-)=i16 2, precision (6)=i16 2) -> (F-format string=w380:string)  [unwired: 1 in]
                n156 = Concatenate Strings(w380, " mm") -> (w370:string)
                n157 = case shown="True" "SHOW SCALE BAR" {
                  tunnel: w385 -> [w394 w412]
                  tunnel: w370 -> [_ w410]
                  tunnel: [w393 w402] -> w387
                  tunnel: [w395 w401] -> w388
                  tunnel: "HSCALEBAR POSITION" -> [_ w400]
                  tunnel: "VSCALEBAR POSITION" -> [_ w399]
                  tunnel: "HSCALEBAR POSITION TEXT" -> [_ w398]
                  tunnel: w386 -> [w391 w396]
                  frame False {
                    n158 = call "IMAQ Clear Overlay"("Groups"=string[] ["SCALE"], "error in (no error)"=w394, "Image"=w391) -> ("error out"=w393:errorcluster, "Image Out"=w395:T21)  [unwired: 7 in]
                  }
                  frame True {
                    w397 = "SCALE" ("Group")
                    n159 = local read "HSCALEBAR"() -> (w411:u32[][])
                    n160 = call "IMAQ Overlay Bitmap"("Group"=w397, "error in (no error)"=w412, "Bitmap"=w411, "Top Left Point"=w400, "Image"=w396) -> ("error out"=w407:errorcluster, "Image Out"=w408:T21)  [unwired: 5 in]
                    n161 = local read "VSCALEBAR"() -> (w406:u32[][])
                    n162 = call "IMAQ Overlay Bitmap"("Group"=w397, "error in (no error)"=w407, "Bitmap"=w406, "Top Left Point"=w399, "Image"=w408) -> ("error out"=w404:errorcluster, "Image Out"=w405:T21)  [unwired: 5 in]
                    n163 = call "IMAQ Overlay Text"("Group"=w397, "Text Color (black)"=u32 16722686, "Font, Size & Style"=T25 {"Desired Font (Application)"=enum."User-specified Font", "[User-specified Font]"={"Font Name"="calibri", "Size"=48, "Strikeout?"=FALSE, "Italic?"=FALSE, "Underline?"=FALSE, "Outline?"=FALSE, "Shadow?"=FALSE, "Bold?"=FALSE, "Rotation Angle"=0.0}, "Horizontal Alignment"=0, "Vertical Alignment"=0}, "error in (no error)"=w404, "String"=w410, "Origin"=w398, "Image"=w405) -> ("error out"=w402:errorcluster, "Image Out"=w401:T21)  [unwired: 3 in]
                  }
                }
              }
              event "CAMERA CENTRE": Mouse Down {
                n164 = event-data() -> ()  [unwired: 1 in, 8 out]
                n165 = local read "CENTRE CAMERA FOV"() -> (w413:T20)
                n166 = call "IMAQ Overlay Bitmap"("Group"="FEATURES", "Bitmap"=w415, "Top Left Point"=w413, "Image"=w420) -> ("Image Out"=w419:T21)  [unwired: 6 in, 1 out]
              }
              event "CLEAR ROI": Mouse Down {
                n167 = event-data() -> ()  [unwired: 1 in, 8 out]
                n168 = call "IMAQ Clear Overlay"("Groups"=string[] ["SCAN SHAPES"], "error in (no error)"=w422, "Image"=w431) -> ("error out"=w424:errorcluster, "Image Out"=w427:T21)  [unwired: 7 in]
                n169 = call "IMAQ Clear Overlay"("Groups"=string[] ["FIDUCIALS"], "error in (no error)"=w424, "Image"=w427) -> ("error out"=w423:errorcluster, "Image Out"=w426:T21)  [unwired: 7 in]
                n170 = call <vilib>:"Clear Errors.vi"("error in (no error)"=w423) -> ("error out"=w421:errorcluster)  [unwired: 5 in, 1 out]
              }
              event "LOAD ROI": Mouse Down {
                n171 = event-data() -> ()  [unwired: 1 in, 8 out]
                n172 = flat-sequence {
                  tunnel: w437 -> [w439]
                  tunnel: [w439] -> w433
                  tunnel: [w442] -> w436
                  tunnel: w433 -> [w443]
                  frame #0 {
                    n173 = Wait (ms)(milliseconds to wait=u32 200) -> ()  [unwired: 1 out]
                  }
                  frame #1 {
                    n174 = local read "SCAN ROI"() -> (w440:T4)
                    n175 = Unbundle By Name(w440) -> ("Contours"=w441:T19)
                    n176 = for {
                      shift-right: [w450] -> w442
                      shift-left: w443 -> [w451]
                      tunnel: w441 -> [w449] mode=indexing
                      tunnel: w440 -> [w445]
                      n177 = Unbundle By Name(w449) -> ("ROI Type"=w447:u32, "Points"=w444:i32[])
                      n178 = Equal?(x=w447, y=u32 3) -> (x = y?=w448:bool)
                      n179 = case shown="True" w448 {
                        tunnel: w451 -> [w452 w466]
                        tunnel: [w452 w462] -> w450
                        tunnel: w445 -> [_ w465]
                        tunnel: w444 -> [_ w460]
                        frame False {
                        }
                        frame True {
                          w461 = "SCAN SHAPES" ("Group")
                          n180 = Index Array(array=w460, index #1=0 ("index"), index #2=1 ("index")) -> (element #1=w457:i32, element #2=w456:i32)
                          n181 = call "IMAQ Overlay ROI"("Group"=w461, "ROI Descriptor"=w465, "Image"=w466) -> ("error out"=w463:errorcluster, "Image Out"=w464:T21)  [unwired: 7 in]
                          n182 = Bundle("Numeric Control"=w457, "Numeric Control"=w456) -> (w455:T20)  [unwired: 1 in]
                          n183 = local read "NAME"() -> (w454:string)
                          n184 = call "IMAQ Overlay Text"("Group"=w461, "Text Color (black)"=u32 16496895, "error in (no error)"=w463, "String"=w454, "Origin"=w455, "Image"=w464) -> ("Image Out"=w462:T21)  [unwired: 4 in, 1 out]
                        }
                      }
                    }
                  }
                }
              }
              event "SHOW MIRROR": Mouse Down {
                n185 = event-data() -> ()  [unwired: 1 in, 7 out]
                n186 = local read "Contours"() -> (w473:T19)
                n187 = Index Array(array=w473, index=0) -> (element=w486:T36)
                n188 = Unbundle By Name(w486) -> ("Points"=w479:i32[])
                n189 = Index Array(array=w479, index #1=0 ("index"), index #2=1 ("index"), index #3=2 ("index"), index #4=3 ("index")) -> (element #1=w483:i32, element #2=w482:i32, element #3=w481:i32, element #4=w480:i32)
                n190 = Bundle("Numeric Control"=w483, "Numeric Control"=w482, "Numeric Control"=w481, "Numeric Control"=w480) -> (w467:T37)  [unwired: 1 in]
                "MIRROR HOLE" <- w467
                n191 = case shown="False" "SHOW MIRROR" {
                  tunnel: [w490 w498] -> w469
                  tunnel: w472 -> [w491 w495]
                  tunnel: w470 -> [w489 w496]
                  tunnel: [w488 w497] -> w468
                  tunnel: w467 -> [_ w493]
                  frame False {
                    n192 = call "IMAQ Clear Overlay"("Groups"=string[] ["MIRROR"], "error in (no error)"=w489, "Image"=w491) -> ("error out"=w488:errorcluster, "Image Out"=w490:T21)  [unwired: 7 in]
                  }
                  frame True {
                    w494 = u32 0 items=["Frame", "Fill"] ("Drawing Mode (Frame)")
                    n193 = call "IMAQ Overlay Oval"("Group"="MIRROR", "error in (no error)"=w496, "Drawing Mode (Frame)"=w494, "Bounding Rectangle"=w493, "Image"=w495) -> ("error out"=w497:errorcluster, "Image Out"=w498:T21)  [unwired: 5 in]
                  }
                }
              }
              event "ROI ZOOM": Value Change {
                n194 = event-data() -> ()  [unwired: 1 in, 5 out]
                n195 = property class="IMAQdx"(reference=w526, error in=w525, "ActiveAttribute"="DSPSubregionBottom") -> (reference out=w523:T8, error out=w522:errorcluster)
                n196 = Unbundle By Name("DSP ROI") -> ("LEFT"=w501:u32, "RIGHT"=w500:u32, "TOP"=w502:u32, "BOTTOM"=w503:u32)
                n197 = property class="IMAQdx"(reference=w523, error in=w522, "ValueU32"=w503) -> (reference out=w512:T8, error out=w511:errorcluster)
                n198 = property class="IMAQdx"(reference=w512, error in=w511, "ActiveAttribute"="DSPSubregionTop") -> (reference out=w520:T8, error out=w519:errorcluster)
                n199 = property class="IMAQdx"(reference=w520, error in=w519, "ValueU32"=w502) -> (reference out=w510:T8, error out=w509:errorcluster)
                n200 = property class="IMAQdx"(reference=w510, error in=w509, "ActiveAttribute"="DSPSubregionLeft") -> (reference out=w517:T8, error out=w516:errorcluster)
                n201 = property class="IMAQdx"(reference=w517, error in=w516, "ValueU32"=w501) -> (reference out=w508:T8, error out=w507:errorcluster)
                n202 = property class="IMAQdx"(reference=w508, error in=w507, "ActiveAttribute"="DSPSubregionRight") -> (reference out=w514:T8, error out=w513:errorcluster)
                n203 = property class="IMAQdx"(reference=w514, error in=w513, "ValueU32"=w500) -> (reference out=w506:T8, error out=w505:errorcluster)
              }
              event "GAIN": Value Change {
                n204 = event-data() -> ()  [unwired: 1 in, 5 out]
                n205 = property class="IMAQdx"(reference=w532, error in=w531, "ActiveAttribute"="Gain") -> (reference out=w535:T8, error out=w534:errorcluster)
                n206 = local read "GAIN"() -> (w528:sgl)
                n207 = property class="IMAQdx"(reference=w535, error in=w534, "ValueDBL"=w528) -> (reference out=w530:T8, error out=w529:errorcluster)
              }
              event "EXPOSURE": Value Change {
                n208 = event-data() -> ("OldVal"=w548:dbl)  [unwired: 1 in, 5 out]
                n209 = property class="IMAQdx"(reference=w541, error in=w540, "ActiveAttribute"="ExposureTimeAbs") -> (reference out=w543:T8, error out=w542:errorcluster)
                n210 = Multiply(x=w548, y=1000.0) -> (x*y=w545:dbl)
                n211 = property class="IMAQdx"(reference=w543, error in=w542, "ValueDBL"=w545) -> (reference out=w547:T8, error out=w546:errorcluster)
              }
              event "BINNING": Value Change {
                n212 = event-data() -> ()  [unwired: 1 in, 6 out]
                n213 = property class="IMAQdx"(reference=w563, error in=w562, "ActiveAttribute"="CameraAttributes::ImageMode::BinningVertical") -> (reference out=w561:T8, error out=w560:errorcluster)
                n214 = property class="IMAQdx"(reference=w561, error in=w560, "ValueI64"="BINNING") -> (reference out=w555:T8, error out=w554:errorcluster)
                n215 = property class="IMAQdx"(reference=w555, error in=w554, "ActiveAttribute"="CameraAttributes::ImageMode::BinningHorizontal") -> (reference out=w557:T8, error out=w556:errorcluster)
                n216 = property class="IMAQdx"(reference=w557, error in=w556, "ValueI64"="BINNING") -> (reference out=w551:T8, error out=w550:errorcluster)
              }
              event "CALIBRATE VIEW": Mouse Down {
                n217 = event-data() -> ()  [unwired: 1 in, 7 out]
                n218 = stacked-sequence {
                  seq-local: [w567 _] -> [_ w572]
                  frame #0 {
                    # "Microscope CalibrationReal Space Distance"
                    n219 = call "Microscope Calibration"() -> ("Distance"=w567:dbl)  [unwired: 17 in, 2 out]
                  }
                  frame #1 {
                    n220 = property on="MICROSCOPE" class="ImageControl"() -> ("ROI"=w593:T4)  [unwired: 2 in, 2 out]
                    n221 = Unbundle By Name(w593) -> ("Contours"=w595:T19)
                    n222 = local read "ZOOM CALIBRATION FACTORS"() -> (w570:dbl[])
                    n223 = Index Array(array=w595, index=0) -> (element=w594:T36)
                    n224 = Unbundle By Name(w594) -> ("Points"=w592:i32[])
                    n225 = To Single Precision Float(number=w592) -> (single precision float=w582:sgl[])
                    n226 = Index Array(array=w582, index #1=0 ("index"), index #2=2 ("index"), index #3=1 ("index"), index #4=3 ("index")) -> (element #1=w586:sgl, element #2=w585:sgl, element #3=w584:sgl, element #4=w583:sgl)
                    n227 = local read "QUESTAR"() -> (w587:i32)
                    n228 = Subtract(x=w586, y=w585) -> (x-y=w580:sgl)
                    n229 = Subtract(x=w584, y=w583) -> (x-y=w579:sgl)
                    n230 = Absolute Value(x=w580) -> (abs(x)=w575:sgl)
                    n231 = Absolute Value(x=w579) -> (abs(x)=w574:sgl)
                    n232 = Divide(x=w575, y=w574) -> (x/y=w581:sgl)
                    n233 = Multiply(x=w575, y=w575) -> (x*y=w577:sgl)
                    n234 = Multiply(x=w574, y=w574) -> (x*y=w576:sgl)
                    n235 = Inverse Tangent(1:w581) -> (0:→"ANGLE 2":sgl)
                    n236 = Add(x=w577, y=w576) -> (x+y=w573:sgl)
                    n237 = Square Root(x=w573) -> (sqrt(x)=w571:sgl)
                    n238 = Divide(x=w572, y=w571) -> (x/y=w569:dbl)
                    "CALIBRATION FACTOR" <- w569
                    n239 = Replace Array Subset(array=w570, new element=w569, index=w587) -> (w568:dbl[])
                    n240 = local write "ZOOM CALIBRATION FACTORS"(w568) -> ()
                  }
                }
              }
              event "LENGTH 2": Mouse Down {
                n241 = event-data() -> ()  [unwired: 1 in, 7 out]
                n242 = property on="MICROSCOPE" class="ImageControl"() -> ("ROI"=w621:T4)  [unwired: 2 in, 2 out]
                n243 = Unbundle By Name(w621) -> ("Contours"=w623:T19)
                n244 = Index Array(array=w623, index=0) -> (element=w624:T36)
                n245 = Unbundle By Name(w624) -> ("Points"=w617:i32[])
                n246 = Index Array(array=w617, index #1=0 ("index"), index #2=1 ("index"), index #3=2 ("index"), index #4=3 ("index")) -> (element #1=w612:i32, element #2=w610:i32, element #3=w611:i32, element #4=w609:i32)
                n247 = Subtract(x=w610, y=w609) -> (x-y=w607:i32)
                n248 = Subtract(x=w612, y=w611) -> (x-y=w608:i32)
                n249 = Absolute Value(x=w608) -> (abs(x)=w606:i32)
                n250 = Absolute Value(x=w607) -> (abs(x)=w605:i32)
                n251 = local read "CALIBRATION FACTOR"() -> (w600:dbl)
                n252 = Multiply(x=w606, y=w606) -> (x*y=w604:i32)
                n253 = Multiply(x=w605, y=w605) -> (x*y=w602:i32)
                n254 = Add(x=w604, y=w602) -> (x+y=w603:i32)
                n255 = To Double Precision Float(number=w603) -> (double precision float=w601:dbl)
                n256 = Square Root(x=w601) -> (sqrt(x)=w599:dbl)
                n257 = Multiply(x=w599, y=w600) -> (x*y=→"LENGTH":dbl)
              }
            }
            n258 = local read "GLOBAL STOP"() -> (w174:bool)
          }
          n259 = call "IMAQ AVI2 Close"("AVI Refnum"=w87) -> ()  [unwired: 10 in, 1 out]
          n260 = call <vilib>:"IMAQdx Close Camera.vi"("error in"=w162, "Session In"=w161) -> ("error out"=w154:errorcluster)  [unwired: 9 in]
          n261 = call "IMAQ Dispose"("All Images? (No)"=TRUE, "Image"=w100, "error in (no error)"=w154) -> ()  [unwired: 3 in, 1 out]
        }
      }
      n262 = case shown="True" "ENABLE STAGE AND DAQ LOOP" {
        frame False {
        }
        frame True {
          # "STAGE AND SCAN LOOP (SLOWER)"
          n263 = property on="REL XYZ STAGE" class="Clust (strict)"("Visible"=FALSE) -> ()  [unwired: 2 in, 2 out]
          n264 = while {
            shift-right: [w641] -> _
            shift-left: u32 0 -> [w643]
            tunnel: "QUEU PATH" -> [w642]
            shift-right: [w640] -> _
            shift-left: i16 0 -> [w639]
            stop <- w638 stop-if-true
            n265 = event shown="[12] \"START SEQ\": Mouse Down" {
              selector: _ -> [_ _ _ _ _ _ _ _ _ _ _ _ _ _ _ _ _ _ _ _ _ _ _ _ _ _ _ _ _ _ _ _ _ _ _ _ _ _ _ _ _ _ _ _]
              dyn-events: _ -> [_ _ _ _ _ _ _ _ _ _ _ _ _ _ _ _ _ _ _ _ _ _ _ _ _ _ _ _ _ _ _ _ _ _ _ _ _ _ _ _ _ _ _ _]
              timeout: 100 -> [_ _ _ _ _ _ _ _ _ _ _ _ _ _ _ _ _ _ _ _ _ _ _ _ _ _ _ _ _ _ _ _ _ _ _ _ _ _ _ _ _ _ _ _]
              tunnel: [w709 _ _ w775 w827 w862 w865 w904 w918 w939 w1014 w1037 w1043 w1083 w1086 w1114 _ w1273 _ _ _ _ _ _ _ _ w1319 w1323 w1328 w1330 w1331 w1335 w1339 w1348 w1349 w1364 w1372 w1382 w1390 w1398 w1407 w1410 _ _] -> w641
              tunnel: w643 -> [w709 _ _ w775 w827 w862 w865 w904 w918 w939 w1014 w1037 w1043 w1083 w1086 w1114 _ w1273 _ _ _ _ _ _ _ _ w1319 w1323 w1328 w1330 w1331 w1335 w1339 w1348 w1349 w1364 w1372 w1382 w1390 w1398 w1407 w1410 _ _]
              tunnel: w642 -> [_ _ _ _ _ _ _ _ _ _ _ _ _ _ _ _ _ _ _ _ _ _ _ _ _ _ _ _ _ _ _ _ _ _ _ _ _ _ _ _ _ _ _ _]
              tunnel: [w697 _ w757 _ _ _ _ _ _ _ _ w1028 w1040 w1080 _ _ w1240 w1272 _ _ _ _ _ _ _ _ _ _ _ _ _ _ _ _ _ _ _ _ _ _ _ _ _ _] -> w640
              tunnel: w639 -> [w696 _ w757 _ _ _ _ _ _ _ _ w1028 w1040 w1080 _ _ w1240 w1272 _ _ _ _ _ _ _ _ _ _ _ _ _ _ _ _ _ _ _ _ _ _ _ _ _ _]
              event Timeout {
                w671 = 1
                w706 = TRUE ("Visible")
                w707 = TRUE ("Visible")
                n266 = event-data() -> ()  [unwired: 1 in, 2 out]
                n267 = property on="EXTERNAL/TRANSLATED LIST" class="Tbl (strict)"() -> ("Selection Start"=w669:T38)  [unwired: 2 in, 2 out]
                n268 = property on="SCAN LIST" class="Tbl (strict)"() -> ("Selection Start"=w675:T38)  [unwired: 2 in, 2 out]
                n269 = Unbundle By Name(w675) -> ("Row"=→"SCAN ROW":i32)
                n270 = Unbundle By Name(w669) -> ("Row"=→"EXT POINTS ROW":i32)
                n271 = property on="IN" class="Bool (strict)"("Visible"=w707) -> ()  [unwired: 2 in, 2 out]
                n272 = property on="OUT" class="Bool (strict)"("Visible"=w707) -> ()  [unwired: 2 in, 2 out]
                n273 = property on="MICROSCOPE" class="ImageControl"() -> ("ROI"=w691:T4)  [unwired: 2 in, 2 out]
                n274 = local write "SCAN ROI"(w691) -> ()
                n275 = property on="RIGHT" class="Bool (strict)"("Visible"=w706) -> ()  [unwired: 2 in, 2 out]
                n276 = property on="LEFT" class="Bool (strict)"("Visible"=w706) -> ()  [unwired: 2 in, 2 out]
                n277 = property on="DOWN" class="Bool (strict)"("Visible"=w706) -> ()  [unwired: 2 in, 2 out]
                n278 = property on="UP" class="Bool (strict)"("Visible"=w706) -> ()  [unwired: 2 in, 2 out]
                n279 = property on="SCAN ROI" class="Clust (strict)"() -> ("Value"=w690:T4)  [unwired: 2 in, 2 out]
                n280 = property on="NEW ROI" class="Clust (strict)"("Val(Sgnl)"=w690) -> ()  [unwired: 2 in, 2 out]
                n281 = property on="SCANNING METH" class="Ring (strict)"("DisabledEnum"=T27."Enabled" ("Disabled")) -> ()  [unwired: 2 in, 2 out]
                n282 = local read "BEAM TO STAGE OFFSETS"() -> (w698:cluster{"X":dbl[unit], "Y":dbl[unit]}[])
                n283 = local read "QUESTAR"() -> (w658:i32)
                n284 = Compound Arithmetic op=MULTIPLY("Q", "LINE PASSES", "OVERSCAN") -> (→"Q per PIXEL":dbl[unit])
                n285 = Index Array(array="ZOOM CALIBRATION FACTORS", index=w658) -> (element=→"CURRENT ZOOM CAL":dbl)
                n286 = Index Array(array=w698, index=w658) -> (element=→"BEAM OFFSET":cluster{"X":dbl[unit], "Y":dbl[unit]})
                n287 = Unbundle By Name("MODE & METHOD") -> ("SCAN MODE"=w663:u16)
                n288 = Unbundle By Name("SCANNING") -> ("X-AMP"=w689:dbl[unit], "dX"=w688:dbl[unit], "Y-AMP"=w687:dbl[unit], "dY"=w686:dbl[unit])
                n289 = case shown="1" w663 {
                  tunnel: "SCANNING DIMENSIONS" -> [w715 w717 w720]
                  tunnel: [w714 w716 w719] -> w665
                  frame 0, Default {
                    n290 = Unbundle By Name(w715) -> ("XPIXELS"=w714:i32)
                  }
                  frame 1 {
                    n291 = Unbundle By Name(w717) -> ("YPIXELS"=w716:i32)
                  }
                  frame 2 {
                    w718 = i8 2 items=["DWELL TIME", "TOTAL CHARGE", "STEPX"] ("DOSE NORM")
                    n292 = local write "DOSE NORM"(w718) -> ()
                    n293 = Unbundle By Name(w720) -> ("XPIXELS"=w719:i32)
                  }
                }
                n294 = Divide(x=w687, y=w686) -> (x/y=w684:dbl)
                n295 = Divide(x=w689, y=w688) -> (x/y=w685:dbl)
                n296 = Round To Nearest(number=w684) -> (nearest integer value=w682:dbl)
                n297 = Round To Nearest(number=w685) -> (nearest integer value=w683:dbl)
                n298 = Multiply(x=w683, y=w682) -> (x*y=w681:dbl)
                n299 = case shown="False" "PIXEL DEPTH" {
                  tunnel: [FALSE ("Visible") TRUE ("Visible")] -> w703
                  frame False {
                    n300 = local read "DWELL"() -> (w725:sgl[unit])
                    n301 = local read "Q"() -> (w724:dbl[unit])
                    n302 = local write "dt"(w725) -> ()
                    n303 = local write "dQ"(w724) -> ()
                  }
                  frame True {
                  }
                }
                n304 = case shown="2" "SPEED" {
                  tunnel: [dbl[unit] 1e-06 ("DX") dbl[unit] 9.999999999999999e-06 ("DX") dbl[unit] 9.999999999999999e-05 ("DX") dbl[unit] 0.0005 ("DX") dbl[unit] 0.002 ("DX") "DX"] -> w712
                  tunnel: [dbl[unit] 1e-06 ("DY") dbl[unit] 9.999999999999999e-06 ("DY") dbl[unit] 9.999999999999999e-05 ("DY") dbl[unit] 0.0005 ("DY") dbl[unit] 0.002 ("DY") "DY"] -> w711
                  tunnel: [dbl[unit] 1e-06 ("DZ") dbl[unit] 9.999999999999999e-06 ("DZ") dbl[unit] 9.999999999999999e-05 ("DZ") dbl[unit] 9.999999999999999e-05 ("DZ") dbl[unit] 0.00025 ("DZ") "DZ"] -> w710
                  frame 0, Default {
                  }
                  frame 1 {
                  }
                  frame 2 {
                  }
                  frame 3 {
                  }
                  frame 4 {
                  }
                  frame 5 {
                  }
                }
                n305 = Unbundle By Name("POSITION") -> ("X"=w655:dbl[unit], "Y"=w654:dbl[unit], "Z"=w653:dbl[unit])
                n306 = Multiply(x=w681, y="DWELL") -> (x*y=w680:dbl[unit])
                "TIME" <- w680
                n307 = call "Show_Cursor.vi"("show?"=TRUE) -> ()
                n308 = Multiply(x=w680, y="BEAM CURRENT") -> (x*y=→"CHARGE":dbl[unit])
                n309 = node(w655) -> (w652:dbl)
                n310 = node(w654) -> (w651:dbl)
                n311 = node(w653) -> (w650:dbl)
                n312 = Divide(x="BUFFERED PIXELS", y=w665) -> (x/y=→"Horizontal Graduated Bar":dbl)
                n313 = local write "DX"(w712) -> ()
                n314 = local write "DY"(w711) -> ()
                n315 = local write "DZ"(w710) -> ()
                n316 = Equal To 0?(x=w652) -> (x = 0?=w649:bool)
                n317 = Equal To 0?(x=w651) -> (x = 0?=w648:bool)
                n318 = Equal To 0?(x=w650) -> (x = 0?=w647:bool)
                n319 = Compound Arithmetic op=AND(w649, w648, w647) -> (w646:bool)
                "LOST CONNECTION?" <- w646
                n320 = property on="dQ" class="DigNum (strict)"("Visible"=w703) -> ()  [unwired: 2 in, 2 out]
                n321 = property on="dt" class="DigNum (strict)"("Visible"=w703) -> ()  [unwired: 2 in, 2 out]
                n322 = property on="EXPOSURE" class="Slide (strict)"("BuiltInMouseWheelSupport"=T26."On Hover or Key Focus" ("Built-In Mouse Wheel Support")) -> ()  [unwired: 2 in, 2 out]
                n323 = Boolean To (0,1)(Boolean=w646) -> (0, 1=w645:i16)
                n324 = local read "BEAM CURRENT"() -> (w702:dbl[unit])
                n325 = Add(x=w645, y=w696) -> (x+y=w697:i16)
                n326 = property on="SCAN LIST" class="Tbl (strict)"("SmoothHScroll"=TRUE ("Smooth Horizontal Scrolling")) -> ()  [unwired: 2 in, 2 out]
                n327 = Bundle(w671, w671) -> (w672:cluster{i32, i32})  [unwired: 1 in]
                n328 = node(w702) -> (w701:dbl)
                n329 = property on="SCAN LIST" class="Tbl (strict)"("Selection Color"=u32 6618880, "Selection Size"=w672) -> ()  [unwired: 2 in, 2 out]
                n330 = Equal To 0?(x=w701) -> (x = 0?=w699:bool)
                n331 = case shown="True" w699 {
                  tunnel: [FALSE TRUE] -> w700
                  frame False {
                  }
                  frame True {
                  }
                }
                n332 = property on="BEAM CURRENT" class="DigNum (strict)"("Blinking"=w700) -> ()  [unwired: 2 in, 2 out]
              }
              event "SAMPLE HOLDER": Mouse Down {
                n333 = event-data() -> ()  [unwired: 1 in, 8 out]
                n334 = case shown="2" "SAMPLE HOLDER" {
                  tunnel: [FALSE TRUE FALSE FALSE] -> w745
                  frame 0, Default {
                  }
                  frame 1 {
                  }
                  frame 2 {
                  }
                  frame 3 {
                  }
                }
                n335 = property on="SCALE BAR" class="Bool (strict)"("Visible"=w745) -> ()  [unwired: 2 in, 2 out]
                n336 = property on="RUBY" class="Bool (strict)"("Visible"=w745) -> ()  [unwired: 2 in, 2 out]
                n337 = property on="YAG" class="Bool (strict)"("Visible"=w745) -> ()  [unwired: 2 in, 2 out]
                n338 = property on="YAP" class="Bool (strict)"("Visible"=w745) -> ()  [unwired: 2 in, 2 out]
              }
              event "MODE & METHOD.SCAN MODE": Value Change {
                n339 = event-data() -> ("NewVal"=w756:u16)  [unwired: 1 in, 5 out]
                n340 = case shown="4" w756 {
                  tunnel: [3 2 3 0 0] -> w755
                  tunnel: [w760 w763 w767 w770 w773] -> w754
                  tunnel: [w760 w763 w767 w770 w773] -> w753
                  tunnel: [TRUE w763 TRUE w770 w773] -> w752
                  tunnel: [w760 w763 w767 w770 w773] -> w751
                  frame 0, Default {
                    w758 = u32 3 items=["No Selection", "Point", "Line", "Rectangle", "Oval", "Polygon", "Freehand Region", "Annulus", "Zoom", "Pan", "Broken Line", "Freehand Line", "Rotated Rectangle"] ("Tool (Point)")
                    w760 = FALSE
                    n341 = call "IMAQ WindToolsSelect"("Tool (Point)"=w758) -> ()  [unwired: 4 in, 2 out]
                  }
                  frame 1 {
                    w762 = u32 2 items=["No Selection", "Point", "Line", "Rectangle", "Oval", "Polygon", "Freehand Region", "Annulus", "Zoom", "Pan", "Broken Line", "Freehand Line", "Rotated Rectangle"] ("Tool (Point)")
                    w763 = FALSE
                    n342 = call "IMAQ WindToolsSelect"("Tool (Point)"=w762) -> ()  [unwired: 4 in, 2 out]
                  }
                  frame 2 {
                    w765 = u32 3 items=["No Selection", "Point", "Line", "Rectangle", "Oval", "Polygon", "Freehand Region", "Annulus", "Zoom", "Pan", "Broken Line", "Freehand Line", "Rotated Rectangle"] ("Tool (Point)")
                    w767 = FALSE
                    n343 = call "IMAQ WindToolsSelect"("Tool (Point)"=w765) -> ()  [unwired: 4 in, 2 out]
                  }
                  frame 4 {
                    w769 = u32 5 items=["No Selection", "Point", "Line", "Rectangle", "Oval", "Polygon", "Freehand Region", "Annulus", "Zoom", "Pan", "Broken Line", "Freehand Line", "Rotated Rectangle"] ("Tool (Point)")
                    w770 = FALSE
                    n344 = call "IMAQ WindToolsSelect"("Tool (Point)"=w769) -> ()  [unwired: 4 in, 2 out]
                  }
                  frame 3 {
                    w772 = u32 1 items=["No Selection", "Point", "Line", "Rectangle", "Oval", "Polygon", "Freehand Region", "Annulus", "Zoom", "Pan", "Broken Line", "Freehand Line", "Rotated Rectangle"] ("Tool (Point)")
                    w773 = FALSE
                    n345 = call "IMAQ WindToolsSelect"("Tool (Point)"=w772) -> ()  [unwired: 4 in, 2 out]
                  }
                }
                n346 = property on="MICROSCOPE" class="ImageControl"("Polygon Tool Button Visible"=w754, "Polyline Tool Button Visible"=w753, "Rectangle Tool Button Visible"=w752, "Rotated Rectangle Tool Button Visible"=w751) -> ()  [unwired: 2 in, 2 out]
                n347 = local write "Tab Control 4"(w755) -> ()
              }
              event "BEAM CENTRE": Mouse Down {
                n348 = event-data() -> ()  [unwired: 1 in, 7 out]
                n349 = stacked-sequence {
                  frame #0 {
                    n350 = property on="MICROSCOPE" class="ImageControl"() -> ("ROI"=w778:T4)  [unwired: 2 in, 2 out]
                    n351 = Unbundle By Name(w778) -> ("Contours"=w776:T19)
                    n352 = Array Size(array=w776) -> (size(s)=w777:i32)
                    n353 = for {
                      N: w777 -> [_]
                      tunnel: w776 -> [w785]
                      i -> [w784]
                      n354 = Index Array(array=w785, index=w784) -> (element=w783:T36)
                      n355 = Unbundle(w783) -> ("Contour Type"=w782:u32, "Points"=w781:i32[])  [unwired: 1 out]
                      n356 = Equal?(x=u32 0, y=w782) -> (x = y?=w780:bool)
                      n357 = case shown="True" w780 {
                        tunnel: w781 -> [_ w794]
                        frame False {
                          n358 = local write "XBCENTRE"(sgl 0.0 ("XCENTRE")) -> ()
                          n359 = local write "YBCENTRE"(sgl 0.0 ("YCENTRE")) -> ()
                        }
                        frame True {
                          n360 = Index Array(array=w794, index #1=0 ("index"), index #2=1 ("index")) -> (element #1=w791:i32, element #2=w790:i32)
                          n361 = To Single Precision Float(number=w791) -> (single precision float=→"XBCENTRE":sgl)
                          n362 = To Single Precision Float(number=w790) -> (single precision float=→"YBCENTRE":sgl)
                        }
                      }
                    }
                  }
                  frame #1 {
                    w816 = 5 ("y")
                    # "+ve x offset means Xb is right of Xc\n+ve y offset means Yb is below Yc"
                    # "Convert to Stage Space"
                    # "Image Space"
                    # "Beam centre is referenced to middle of camera FOV"
                    # "OFFSETS"
                    n363 = local read "CURRENT ZOOM CAL"() -> (w795:dbl)
                    n364 = node(w795) -> (w811:dbl[unit])
                    n365 = local read "IMAGE XCENTRE"() -> (w797:dbl)
                    n366 = local read "IMAGE YCENTRE"() -> (w796:dbl)
                    n367 = Multiply(x=w797, y=w795) -> (x*y=w813:dbl)
                    n368 = Multiply(x=w796, y=w795) -> (x*y=w812:dbl)
                    n369 = node(w813) -> (w803:dbl[unit])
                    "XC" <- w803
                    n370 = node(w812) -> (w801:dbl[unit])
                    "YC" <- w801
                    n371 = local read "XBCENTRE"() -> (w807:sgl)
                    n372 = local read "YBCENTRE"() -> (w806:sgl)
                    n373 = Multiply(x=w807, y=w811) -> (x*y=w804:dbl[unit])
                    n374 = Multiply(x=w806, y=w811) -> (x*y=w802:dbl[unit])
                    n375 = Subtract(x=w804, y=w803) -> (x-y=w799:dbl[unit])
                    n376 = Subtract(x=w802, y=w801) -> (x-y=w800:dbl[unit])
                    n377 = Add(x=w806, y=w816) -> (x+y=w818:sgl)
                    n378 = Subtract(x=w806, y=w816) -> (x-y=w820:sgl)
                    n379 = Add(x=w807, y=w816) -> (x+y=w819:sgl)
                    n380 = Subtract(x=w807, y=w816) -> (x-y=w817:sgl)
                    n381 = Negate(x=w800) -> (-x=w798:dbl[unit])
                    n382 = local read "BEAM CENTRE MARK"() -> (w815:cluster{"L":i32, "T":i32, "R":i32, "B":i32}[])
                    n383 = local read "BEAM TO STAGE OFFSETS"() -> (w810:cluster{"X":dbl[unit], "Y":dbl[unit]}[])
                    n384 = Bundle(w817, w818, w819, w820) -> (w821:cluster{sgl, sgl, sgl, sgl})  [unwired: 1 in]
                    n385 = Bundle(w799, w798) -> (w808:cluster{dbl[unit], dbl[unit]})  [unwired: 1 in]
                    n386 = local read "QUESTAR"() -> (w805:i32)
                    n387 = Replace Array Subset(array=w810, new element=w808, index=w805) -> (w809:cluster{"X":dbl[unit], "Y":dbl[unit]}[])
                    n388 = local write "BEAM TO STAGE OFFSETS"(w809) -> ()
                    n389 = Replace Array Subset(array=w815, new element=w821, index=w805) -> (w814:cluster{"L":i32, "T":i32, "R":i32, "B":i32}[])
                    n390 = local write "BEAM CENTRE MARK"(w814) -> ()
                  }
                }
              }
              event "LOAD NMP LIST": Value Change {
                n391 = event-data() -> ()  [unwired: 1 in, 6 out]
                n392 = call-poly <vilib>:"Read From Spreadsheet File.vi"("transpose (no:F)"=FALSE) -> ("all rows"=w825:string[][])  [unwired: 6 in, 4 out]
                n393 = local read "SCAN LIST ARRAY"() -> (w824:T2)
                n394 = Index Array(array=w824, index=0) -> (element=w822:T39)
                n395 = for {
                  tunnel: w825 -> [w841] mode=indexing
                  tunnel: w822 -> [w828]
                  n396 = Index Array(array=w841, index #1=0 ("index"), index #2=1 ("index"), index #3=2 ("index"), index #4=3 ("index")) -> (element #2=w839:string, element #3=w838:string, element #4=w834:string)  [unwired: 1 in, 2 out]
                  n397 = Fract/Exp String To Number(string=w839) -> (number=w833:dbl)  [unwired: 3 in, 1 out]
                  n398 = Fract/Exp String To Number(string=w838) -> (number=w832:dbl)  [unwired: 3 in, 1 out]
                  n399 = Fract/Exp String To Number(string=w834) -> (number=w831:dbl)  [unwired: 3 in, 1 out]
                  n400 = node(w833) -> ()  [unwired: 1 out]
                  n401 = node(w832) -> ()  [unwired: 1 out]
                  n402 = node(w831) -> ()  [unwired: 1 out]
                  n403 = local read "SCAN LIST ARRAY"() -> (w830:T2)
                  n404 = Build Array (concatenate)(w830, w828) -> (w829:T2)
                  n405 = local write "SCAN LIST ARRAY"(w829) -> ()
                }
              }
              event "LOAD": Mouse Down {
                # "LANDMARK"
                n406 = event-data() -> ()  [unwired: 1 in, 8 out]
                n407 = call "Transform External Geometry from Optical Microscope.vi"("SCAN POINT LIST"="SCAN POINT LIST") -> ("EXT POINTS ARRAY"=→"EXT POINTS ARRAY":T5, "EXTERNAL POINT LIST"=w842:string[][])  [unwired: 10 in, 7 out]
                n408 = local read "LANDMARKS FOR HOLDERS"() -> (w859:T14)
                n409 = local read "SAMPLE HOLDER"() -> (w858:u16)
                n410 = local write "EXTERNAL/TRANSLATED LIST"(w842) -> ()
                n411 = Index Array(array=w842, index (row)=0, index (col)=1 ("disabled index (col)")) -> (element=w853:string)
                n412 = Index Array(array=w842, index (row)=0, index (col)=2 ("disabled index (col)")) -> (element=w849:string)
                n413 = Fract/Exp String To Number(string=w853) -> (number=w851:dbl)  [unwired: 3 in, 1 out]
                n414 = Fract/Exp String To Number(string=w849) -> (number=w848:dbl)  [unwired: 3 in, 1 out]
                n415 = node(w851) -> (w847:dbl[unit])
                n416 = node(w848) -> (w844:dbl[unit])
                n417 = Index Array(array=w859, index=w858) -> (element=w854:T3)
                n418 = Unbundle By Name(w854) -> ("X"=w852:dbl[unit], "Y"=w843:dbl[unit])
                n419 = Subtract(x=w852, y=w847) -> (x-y=→"XOFFSET":dbl[unit])
                n420 = Subtract(x=w844, y=w843) -> (x-y=→"YOFFSET":dbl[unit])
              }
              event "SET ACCURATE LANDMARK": Mouse Down {
                n421 = event-data() -> ()  [unwired: 1 in, 8 out]
                n422 = local read "EXTERNAL/TRANSLATED LIST"() -> (w864:string[][])
                n423 = case shown="True" "SET ACCURATE LANDMARK" {
                  tunnel: w864 -> [_ w868]
                  frame False {
                  }
                  frame True {
                    # "R2"
                    # "R1"
                    n424 = Index Array(array=w868, index (row)=1, index (col)=1 ("disabled index (col)")) -> (element=w893:string)
                    n425 = Index Array(array=w868, index (row)=1, index (col)=2 ("disabled index (col)")) -> (element=w890:string)
                    n426 = Index Array(array=w868, index (row)=2, index (col)=1 ("disabled index (col)")) -> (element=w885:string)
                    n427 = Index Array(array=w868, index (row)=2, index (col)=2 ("disabled index (col)")) -> (element=w882:string)
                    n428 = local read "XOFFSET"() -> (w867:dbl[unit])
                    n429 = local read "YOFFSET"() -> (w866:dbl[unit])
                    n430 = Fract/Exp String To Number(string=w893) -> (number=w892:dbl)  [unwired: 3 in, 1 out]
                    n431 = Fract/Exp String To Number(string=w890) -> (number=w889:dbl)  [unwired: 3 in, 1 out]
                    n432 = Fract/Exp String To Number(string=w885) -> (number=w884:dbl)  [unwired: 3 in, 1 out]
                    n433 = Fract/Exp String To Number(string=w882) -> (number=w881:dbl)  [unwired: 3 in, 1 out]
                    n434 = node(w892) -> (w880:dbl[unit])
                    n435 = node(w889) -> (w879:dbl[unit])
                    n436 = node(w884) -> (w878:dbl[unit])
                    n437 = node(w881) -> (w877:dbl[unit])
                    n438 = local read "POSITION"() -> (w874:T3)
                    n439 = Add(x=w867, y=w880) -> (x+y=w876:dbl[unit])
                    n440 = Add(x=w866, y=w879) -> (x+y=w875:dbl[unit])
                    n441 = Add(x=w867, y=w878) -> (x+y=w871:dbl[unit])
                    n442 = Add(x=w866, y=w877) -> (x+y=w870:dbl[unit])
                    n443 = Unbundle By Name(w874) -> ("Z"=w869:dbl[unit])
                    n444 = Bundle(w876, w875, "Z"=w869) -> (w873:cluster{dbl[unit], dbl[unit], "Z":dbl[unit]})  [unwired: 1 in]
                    n445 = Bundle(w871, w870, "Z"=w869) -> (w872:cluster{dbl[unit], dbl[unit], "Z":dbl[unit]})  [unwired: 1 in]
                    n446 = local write "REF#1"(w873) -> ()
                    n447 = local write "REF#2"(w872) -> ()
                  }
                }
              }
              event "TRANS": Mouse Down {
                n448 = event-data() -> ()  [unwired: 1 in, 8 out]
                n449 = local read "SCAN POINT LIST"() -> (w901:path)
                n450 = local read "REF#1"() -> (w902:T3)
                n451 = local read "REF#2"() -> (w903:T3)
                n452 = call "Transform External Geometry from Optical Microscope.vi"("NMP R1"=w902, "NMP R2"=w903, "SCAN POINT LIST"=w901, "SWAP REF#1/REF#2"="SWAP REF#1/REF#2") -> ("TRANS POINT ARRAY"=w898:T5, "NMP OK"=→"NMP ORDER OK ?":bool)  [unwired: 7 in, 7 out]
                "TRANS POINT ARRAY" <- w898
                n453 = for {
                  tunnel: w898 -> [w914] mode=indexing
                  tunnel: [w905] -> w897 mode=indexing
                  n454 = Unbundle By Name(w914) -> ("POINT"=w907:string, "X"=w913:dbl[unit], "Y"=w911:dbl[unit], "Z"=w910:dbl[unit], "COMMENT"=w906:string)
                  n455 = node(w913) -> (w912:dbl)
                  n456 = node(w911) -> (w909:dbl)
                  n457 = node(w910) -> (w908:dbl)
                  n458 = Number To Fractional String(number=w912) -> (F-format string=w917:string)  [unwired: 3 in]
                  n459 = Number To Fractional String(number=w909) -> (F-format string=w916:string)  [unwired: 3 in]
                  n460 = Number To Fractional String(number=w908) -> (F-format string=w915:string)  [unwired: 3 in]
                  n461 = Build Array(w907, w917, w916, w915, w906) -> (w905:string[])
                }
                "EXTERNAL/TRANSLATED LIST" <- w897
              }
              event "SAVE LIST": Mouse Down {
                n462 = event-data() -> ()  [unwired: 1 in, 8 out]
                n463 = call-poly <vilib>:"Write To Spreadsheet File.vi"() -> ()  [unwired: 8 in, 1 out]
              }
              event "ADD POINT TO LIST": Mouse Down {
                (unwired) string[] ["Name", "Xs", "Ys", "Zs", "Mode", "Norm", "Time", "dt", "Q", "dQ", "Overscan", "Lines", "Xamp", "dX", "Yamp", "dY", "Xshift", "Yshift", "Theta", "Phi", "Fly Mode"] ("Column Header Strings[]")
                n464 = event-data() -> ()  [unwired: 1 in, 8 out]
                n465 = local read "MODE & METHOD"() -> (w927:cluster{"SCAN MODE":u16, "SCANNING METH":u16})
                n466 = Unbundle By Name(w927) -> ("SCAN MODE"=w926:u16)
                n467 = case shown="3" w926 {
                  tunnel: [w940 w941] -> w932
                  frame 1, Default {
                    n468 = local read "SCAN ORIGIN"() -> (w940:T3)
                  }
                  frame 3 {
                    n469 = local read "POSITION"() -> (w941:T3)
                  }
                }
                n470 = local read "DOSE NORM"() -> (w934:i8)
                n471 = local read "PIXEL DEPTH"() -> (w935:bool)
                n472 = local read "LINE PASSES"() -> (w937:i32)
                n473 = local read "COMMENT"() -> (w924:string)
                n474 = local read "OVERSCAN"() -> (w936:i32)
                n475 = local read "SCANNING"() -> (w933:T12)
                n476 = local read "NAME"() -> (w925:string)
                n477 = local read "DWELL"() -> (w931:sgl[unit])
                n478 = local read "dQ"() -> (w928:sgl[unit])
                n479 = local read "dt"() -> (w930:sgl[unit])
                n480 = local read "Q"() -> (w929:dbl[unit])
                n481 = local read "SCAN LIST ARRAY"() -> (w921:T2)
                n482 = Index Array(array=w921, index=0) -> (element=w938:T39)
                n483 = Bundle By Name(cluster=w938, "DOSE NORM"=w934, "POINT"=w925, "MODE & METHOD"=w927, "COMMENT"=w924, "OVERSCAN"=w936, "LINE PASSES"=w937, "SCANNING"=w933, "SCAN ORIGIN"=w932, "PIXEL DEPTH"=w935, "DWELL"=w931, "dt"=w930, "Q"=w929, "dQ"=w928) -> (w920:T39)
                n484 = Build Array (concatenate)(w921, w920) -> (w919:T2)
                n485 = for {
                  tunnel: [w993] -> w923 mode=indexing
                  tunnel: w919 -> [w992] mode=indexing
                  w979 = i16 4 ("width (-)")
                  n486 = Unbundle By Name(w992) -> ("POINT"=w994:string, "SCAN ORIGIN.X"=w999:dbl[unit], "SCAN ORIGIN.Y"=w997:dbl[unit], "SCAN ORIGIN.Z"=w996:dbl[unit], "DWELL"=w989:sgl[unit], "Q"=w988:dbl[unit], "dQ"=w982:dbl[unit], "MODE & METHOD"=w991:cluster{"SCAN MODE":u16, "SCANNING METH":u16}, "dt"=w983:sgl[unit], "OVERSCAN"=w970:i32, "SCANNING"=w978:T12, "PIXEL DEPTH"=w946:bool, "DOSE NORM"=w984:i8, "LINE PASSES"=w968:i32)  [unwired: 1 out]
                  n487 = Unbundle By Name(w978) -> ("X-AMP"=w966:dbl[unit], "dX"=w965:dbl[unit], "Y-AMP"=w964:dbl[unit], "dY"=w953:dbl[unit], "X-SHIFT"=w952:dbl[unit], "Y-SHIFT"=w951:dbl[unit], "THETA"=w943:dbl, "PHI"=w942:dbl)
                  n488 = node(w999) -> (w998:dbl)
                  n489 = node(w997) -> (w995:dbl)
                  n490 = node(w996) -> (w985:dbl)
                  n491 = node(w989) -> (w987:sgl)
                  n492 = node(w988) -> (w986:dbl)
                  n493 = Unbundle By Name(w991) -> ("SCAN MODE"=w990:u16)
                  n494 = node(w983) -> (w981:sgl)
                  n495 = node(w982) -> (w980:dbl)
                  n496 = case shown="2" w984 {
                    tunnel: ["DWELL" "CHARGE" "STEPX" "(Xs,Ys)"] -> w975
                    frame 0, Default {
                    }
                    frame 1 {
                    }
                    frame 2 {
                    }
                    frame 3 {
                    }
                  }
                  n497 = case shown="3" w990 {
                    tunnel: ["Xb vs Yb" "Xs vs Yb" "Xs vs Ys" "(Xs,Ys)"] -> w976
                    frame 0, Default {
                    }
                    frame 1 {
                    }
                    frame 2 {
                    }
                    frame 3 {
                    }
                  }
                  n498 = node(w966) -> (w959:dbl)
                  n499 = node(w965) -> (w958:dbl)
                  n500 = node(w964) -> (w957:dbl)
                  n501 = node(w953) -> (w956:dbl)
                  n502 = node(w952) -> (w955:dbl)
                  n503 = node(w951) -> (w954:dbl)
                  n504 = Number To Fractional String(number=w998, width (-)=w979, precision (6)=w979) -> (F-format string=w1001:string)  [unwired: 1 in]
                  n505 = Number To Fractional String(number=w995, width (-)=w979, precision (6)=w979) -> (F-format string=w1000:string)  [unwired: 1 in]
                  n506 = Number To Fractional String(number=w985, width (-)=w979, precision (6)=w979) -> (F-format string=w977:string)  [unwired: 1 in]
                  n507 = Number To Fractional String(number=w987, width (-)=w979, precision (6)=w979) -> (F-format string=w974:string)  [unwired: 1 in]
                  n508 = Number To Fractional String(number=w986, width (-)=w979, precision (6)=w979) -> (F-format string=w972:string)  [unwired: 1 in]
                  n509 = Number To Fractional String(number=w981, width (-)=w979, precision (6)=w979) -> (F-format string=w973:string)  [unwired: 1 in]
                  n510 = Number To Fractional String(number=w980, width (-)=w979, precision (6)=w979) -> (F-format string=w971:string)  [unwired: 1 in]
                  n511 = Number To Decimal String(number=w970) -> (decimal integer string=w969:string)  [unwired: 1 in]
                  n512 = Number To Decimal String(number=w968) -> (decimal integer string=w967:string)  [unwired: 1 in]
                  n513 = Number To Fractional String(number=w959) -> (F-format string=w963:string)  [unwired: 3 in]
                  n514 = Number To Fractional String(number=w958) -> (F-format string=w962:string)  [unwired: 3 in]
                  n515 = Number To Fractional String(number=w957) -> (F-format string=w961:string)  [unwired: 3 in]
                  n516 = Number To Fractional String(number=w956) -> (F-format string=w960:string)  [unwired: 3 in]
                  n517 = Number To Fractional String(number=w955) -> (F-format string=w950:string)  [unwired: 3 in]
                  n518 = Number To Fractional String(number=w954) -> (F-format string=w949:string)  [unwired: 3 in]
                  n519 = Number To Fractional String(number=w943) -> (F-format string=w948:string)  [unwired: 3 in]
                  n520 = Number To Fractional String(number=w942) -> (F-format string=w947:string)  [unwired: 3 in]
                  n521 = Boolean To (0,1)(Boolean=w946) -> (0, 1=w945:i16)
                  n522 = Number To Decimal String(number=w945) -> (decimal integer string=w944:string)  [unwired: 1 in]
                  n523 = Build Array(w994, w1001, w1000, w977, w976, w975, w974, w973, w972, w971, w969, w967, w963, w962, w961, w960, w950, w949, w948, w947, w944) -> (w993:string[])
                }
                n524 = local write "SCAN LIST ARRAY"(w919) -> ()
                n525 = local write "SCAN LIST"(w923) -> ()
              }
              event "MINUS POINT": Mouse Down {
                n526 = event-data() -> ()  [unwired: 1 in, 8 out]
                n527 = local read "SCAN LIST ARRAY"() -> (w1013:T2)
                n528 = Delete From Array(array=w1013, length=1) -> (array with subset deleted=w1011:T2)  [unwired: 1 in, 1 out]
                n529 = local write "SCAN LIST ARRAY"(w1011) -> ()
                n530 = for {
                  tunnel: [w1016] -> w1010 mode=indexing
                  tunnel: w1011 -> [w1015] mode=indexing
                  n531 = Unbundle By Name(w1015) -> ("POINT"=w1018:string, "SCAN ORIGIN.X"=w1024:dbl[unit], "SCAN ORIGIN.Y"=w1022:dbl[unit], "SCAN ORIGIN.Z"=w1021:dbl[unit], "COMMENT"=w1017:string)
                  n532 = node(w1024) -> (w1023:dbl)
                  n533 = node(w1022) -> (w1020:dbl)
                  n534 = node(w1021) -> (w1019:dbl)
                  n535 = Number To Fractional String(number=w1023) -> (F-format string=w1027:string)  [unwired: 3 in]
                  n536 = Number To Fractional String(number=w1020) -> (F-format string=w1026:string)  [unwired: 3 in]
                  n537 = Number To Fractional String(number=w1019) -> (F-format string=w1025:string)  [unwired: 3 in]
                  n538 = Build Array(w1018, w1027, w1026, w1025, w1017) -> (w1016:string[])
                }
                n539 = local write "SCAN LIST"(w1010) -> ()
              }
              event "QUEU": Mouse Down {
                n540 = event-data() -> ()  [unwired: 1 in, 8 out]
                n541 = local read "QUEU TOGGLE"() -> (w1032:bool[])
                n542 = local read "SCAN ROW"() -> (w1031:i32)
                n543 = Bundle("SCAN ROW"=w1031, 0) -> (w1034:cluster{"SCAN ROW":i32, i32})  [unwired: 1 in]
                n544 = Index Array(array=w1032, index=w1031) -> (element=w1033:bool)
                n545 = Not(x=w1033) -> (.not. x?=w1030:bool)
                n546 = case shown="False" w1030 {
                  tunnel: [u32 16717824 u32 2817847] -> w1036
                  frame False {
                  }
                  frame True {
                  }
                }
                n547 = Replace Array Subset(array=w1032, new element=w1030, index=w1031) -> (w1029:bool[])
                n548 = local write "QUEU TOGGLE"(w1029) -> ()
                n549 = property on="SCAN LIST" class="Tbl (strict)"("Active Cell"=w1034, "Cell BG Color"=w1036) -> ()  [unwired: 2 in, 2 out]
              }
              event "START SEQ": Mouse Down {
                n550 = event-data() -> ()  [unwired: 1 in, 8 out]
                n551 = local read "SCAN LIST ARRAY"() -> (w1042:T2)
                n552 = local read "QUEU TOGGLE"() -> (w1041:bool[])
                n553 = for {
                  tunnel: w1042 -> [w1046] mode=indexing
                  tunnel: w1041 -> [w1045] mode=indexing
                  i -> [w1044]
                  n554 = case shown="True" w1045 {
                    tunnel: w1046 -> [_ w1057]
                    tunnel: w1044 -> [_ w1047]
                    frame False {
                    }
                    frame True {
                      n555 = flat-sequence {
                        tunnel: w1057 -> [w1069]
                        tunnel: [w1068] -> w1056
                        tunnel: [w1067] -> w1055
                        tunnel: [w1066] -> w1054
                        tunnel: [w1065] -> w1053
                        tunnel: [w1064] -> w1052
                        tunnel: [w1063] -> w1051
                        tunnel: [w1062] -> w1050
                        tunnel: [w1061] -> w1049
                        tunnel: [w1060] -> w1048
                        tunnel: w1047 -> [w1058]
                        tunnel: w1056 -> [w1070]
                        tunnel: w1055 -> [w1077]
                        tunnel: w1054 -> [w1076]
                        tunnel: w1053 -> [w1075]
                        tunnel: w1052 -> [w1074]
                        tunnel: w1051 -> [w1073]
                        tunnel: w1050 -> [_]
                        tunnel: w1049 -> [w1072]
                        tunnel: w1048 -> [w1071]
                        frame #0 {
                          n556 = property on="SCAN LIST" class="Tbl (strict)"("Cell BG Color"=u32 15204607) -> ()  [unwired: 2 in, 2 out]
                          n557 = Unbundle By Name(w1069) -> ("SCAN ORIGIN"=w1068:T3, "PIXEL DEPTH"=w1067:bool, "DOSE NORM"=w1066:i8, "MODE & METHOD"=w1065:cluster{"SCAN MODE":u16, "SCANNING METH":u16}, "Q"=w1064:dbl[unit], "DWELL"=w1063:sgl[unit], "SCANNING"=w1062:T12, "OVERSCAN"=w1061:i32, "LINE PASSES"=w1060:i32)  [unwired: 2 out]
                          "SCAN ROW 2" <- w1058
                        }
                        frame #1 {
                          n558 = local write "SCAN ORIGIN"(w1070) -> ()
                          n559 = local write "PIXEL DEPTH"(w1077) -> ()
                          n560 = local write "DOSE NORM"(w1076) -> ()
                          n561 = local write "MODE & METHOD"(w1075) -> ()
                          n562 = local write "Q"(w1074) -> ()
                          n563 = local write "DWELL"(w1073) -> ()
                          n564 = local write "OVERSCAN"(w1072) -> ()
                          n565 = local write "LINE PASSES"(w1071) -> ()
                        }
                        frame #2 {
                        }
                        frame #3 {
                        }
                        frame #4 {
                        }
                        frame #5 {
                          n566 = property on="SCAN LIST" class="Tbl (strict)"("Cell BG Color"=u32 23039) -> ()  [unwired: 2 in, 2 out]
                        }
                        frame #6 {
                          n567 = Wait (ms)(milliseconds to wait=u32 100) -> ()  [unwired: 1 out]
                        }
                      }
                    }
                  }
                }
              }
              event "RESET POINTS": Mouse Down {
                w1081 = string[][] [] ("Item Names")
                n568 = event-data() -> ()  [unwired: 1 in, 8 out]
                n569 = local write "EXTERNAL/TRANSLATED LIST"(w1081) -> ()
                n570 = local write "SCAN LIST"(w1081) -> ()
                "SCAN LIST ARRAY" <- T2 [] ("NMP SCAN ARRAY")
              }
              event "CENTRE STAGE": Mouse Down {
                n571 = event-data() -> ()  [unwired: 1 in, 7 out]
                n572 = local read "CALIBRATION FACTOR"() -> (w1087:dbl)
                n573 = local read "IMAGE XCENTRE"() -> (w1085:dbl)
                n574 = local read "IMAGE YCENTRE"() -> (w1084:dbl)
                n575 = stacked-sequence {
                  tunnel: w1087 -> [_ w1112]
                  tunnel: w1085 -> [_ w1108]
                  tunnel: w1084 -> [_ w1107]
                  frame #0 {
                    n576 = property on="MICROSCOPE" class="ImageControl"() -> ("ROI"=w1090:T4)  [unwired: 2 in, 2 out]
                    n577 = Unbundle By Name(w1090) -> ("Contours"=w1089:T19)
                    n578 = Array Size(array=w1089) -> (size(s)=w1088:i32)
                    n579 = for {
                      N: w1088 -> [_]
                      tunnel: w1089 -> [w1097]
                      i -> [w1096]
                      n580 = Index Array(array=w1097, index=w1096) -> (element=w1095:T36)
                      n581 = Unbundle(w1095) -> ("Contour Type"=w1094:u32, "Points"=w1093:i32[])  [unwired: 1 out]
                      n582 = Equal?(x=u32 0, y=w1094) -> (x = y?=w1092:bool)
                      n583 = case shown="True" w1092 {
                        tunnel: w1093 -> [_ w1106]
                        frame False {
                          n584 = local write "XCENTRE"(sgl 0.0 ("XCENTRE")) -> ()
                          n585 = local write "YCENTRE"(sgl 0.0 ("YCENTRE")) -> ()
                        }
                        frame True {
                          n586 = Index Array(array=w1106, index #1=0 ("index"), index #2=1 ("index")) -> (element #1=w1103:i32, element #2=w1102:i32)
                          n587 = To Single Precision Float(number=w1103) -> (single precision float=→"XCENTRE":sgl)
                          n588 = To Single Precision Float(number=w1102) -> (single precision float=→"YCENTRE":sgl)
                        }
                      }
                    }
                  }
                  frame #1 {
                    n589 = local read "POSITION"() -> (w1113:T3)
                    n590 = local read "XCENTRE"() -> (w1111:sgl)
                    n591 = local read "YCENTRE"() -> (w1110:sgl)
                    n592 = call "IMAGE 2 STAGE TRANSLATION.vi"("CENTREY"=w1107, "CENTREX"=w1108, "POSITION"=w1113, "CALIBRATION FACTOR"=w1112, "IMAGE Y"=w1110, "IMAGE X"=w1111) -> ("POINT POSITION"=w1109:cluster{dbl[unit], dbl[unit], "Z":dbl[unit]})  [unwired: 3 in, 2 out]
                    n593 = local write "GOTO POSITION"(w1109) -> ()
                  }
                }
              }
              event "START", "STOP": Mouse Down {
                n594 = event-data() -> ()  [unwired: 1 in, 8 out]
                n595 = flat-sequence {
                  frame #0 {
                    n596 = local read "CALIBRATION FACTOR"() -> (w1120:dbl)
                    n597 = local read "IMAGE XCENTRE"() -> (w1116:dbl)
                    n598 = local read "IMAGE YCENTRE"() -> (w1115:dbl)
                    n599 = local read "Contours"() -> (w1119:T19)
                    n600 = case shown="False" "START" {
                      tunnel: w1120 -> [w1122 w1188]
                      tunnel: w1116 -> [w1124 w1187]
                      tunnel: w1115 -> [w1123 w1186]
                      tunnel: w1119 -> [w1125 w1185]
                      tunnel: "STOP" -> [w1121 _]
                      frame False {
                        n601 = case shown="True" w1121 {
                          tunnel: w1125 -> [_ w1129]
                          tunnel: w1124 -> [_ w1128]
                          tunnel: w1123 -> [_ w1127]
                          tunnel: w1122 -> [_ w1126]
                          frame False {
                          }
                          frame True {
                            n602 = stacked-sequence {
                              tunnel: w1128 -> [_ w1148 w1155 _ _ _]
                              tunnel: w1127 -> [_ w1147 w1154 _ _ _]
                              tunnel: w1126 -> [_ w1149 w1156 _ _ _]
                              tunnel: w1129 -> [w1130 _ _ _ _ _]
                              frame #0 {
                                n603 = Array Size(array=w1130) -> (size(s)=w1131:i32)
                                n604 = for {
                                N: w1131 -> [_]
                                tunnel: w1130 -> [w1140]
                                i -> [w1139]
                                n605 = Index Array(array=w1140, index=w1139) -> (element=w1138:T36)
                                n606 = Unbundle(w1138) -> ("ROI Type"=w1136:u32, "Points"=w1137:i32[])  [unwired: 1 out]
                                n607 = case shown="2, Default" w1136 {
                                tunnel: w1137 -> [w1145]
                                tunnel: [w1144] -> w1135
                                tunnel: [w1143] -> w1134
                                tunnel: [w1142] -> w1133
                                tunnel: [w1141] -> w1132
                                frame 2, Default {
                                n608 = Index Array(array=w1145) -> (element #1=w1144:i32, element #2=w1143:i32, element #3=w1142:i32, element #4=w1141:i32)  [unwired: 4 in]
                                }
                                }
                                n609 = local write "TOPY"(w1134) -> ()
                                n610 = local write "BOTTOMX"(w1133) -> ()
                                n611 = local write "TOPX"(w1135) -> ()
                                n612 = local write "BOTTOMY"(w1132) -> ()
                                }
                              }
                              frame #1 {
                                n613 = local read "TOPX"() -> (w1151:i32)
                                n614 = local read "TOPY"() -> (w1150:i32)
                                n615 = local read "POSITION"() -> (w1152:T3)
                                n616 = call "IMAGE 2 STAGE TRANSLATION.vi"("CENTREY"=w1147, "CENTREX"=w1148, "POSITION"=w1152, "CALIBRATION FACTOR"=w1149, "IMAGE Y"=w1150, "IMAGE X"=w1151) -> ("POINT POSITION"=w1146:cluster{dbl[unit], dbl[unit], "Z":dbl[unit]})  [unwired: 3 in, 2 out]
                                n617 = local write "TOP  STOP"(w1146) -> ()
                              }
                              frame #2 {
                                n618 = local read "BOTTOMX"() -> (w1158:i32)
                                n619 = local read "BOTTOMY"() -> (w1157:i32)
                                n620 = local read "POSITION"() -> (w1159:T3)
                                n621 = call "IMAGE 2 STAGE TRANSLATION.vi"("CENTREY"=w1154, "CENTREX"=w1155, "POSITION"=w1159, "CALIBRATION FACTOR"=w1156, "IMAGE Y"=w1157, "IMAGE X"=w1158) -> ("POINT POSITION"=w1153:cluster{dbl[unit], dbl[unit], "Z":dbl[unit]})  [unwired: 3 in, 2 out]
                                n622 = local write "BOTTOM STOP"(w1153) -> ()
                              }
                              frame #3 {
                                w1166 = dbl[unit] 0.0 ("X-SHIFT")
                                w1167 = 0.0 ("PHI")
                                n623 = local read "BOTTOM STOP"() -> (w1164:T3)
                                n624 = local read "TOP START"() -> (w1174:T3)
                                n625 = local read "TOP  STOP"() -> (w1182:T3)
                                n626 = local read "TOP  STOP"() -> (w1165:T3)
                                n627 = Subtract(x=w1165, y=w1164) -> (x-y=w1163:T3)
                                n628 = Unbundle By Name(w1174) -> ("X"=→"XORIGIN":dbl[unit])
                                n629 = Absolute Value(x=w1163) -> (abs(x)=w1162:T3)
                                n630 = Subtract(x=w1182, y=w1174) -> (x-y=w1180:T3)
                                n631 = Absolute Value(x=w1180) -> (abs(x)=w1181:T3)
                                n632 = Unbundle By Name(w1180) -> ("X"=w1179:dbl[unit])
                                n633 = Unbundle By Name(w1181) -> ("X"=w1173:dbl[unit])
                                "XAMP" <- w1173
                                n634 = Unbundle By Name(w1162) -> ("Y"=w1161:dbl[unit])
                                "YAMP" <- w1161
                                n635 = node(w1179) -> (w1178:dbl)
                                n636 = Less Than 0?(x=w1178) -> (x < 0?=w1177:bool)
                                n637 = Select(t=u8 0, s=w1177, f=u8 1) -> (s? t:f=→"DIRECTION":u8)
                                n638 = Bundle By Name(cluster=T12 {"X-AMP"=0.000225, "dX"=1e-06, "Y-AMP"=0.000252, "dY"=1e-06, "X-SHIFT"=0.0, "Y-SHIFT"=0.0, "THETA"=0.0, "PHI"=0.0} ("SCANNING"), "X-AMP"=w1173, "dX"=dbl[unit] 1e-06, "Y-AMP"=w1161, "dY"=dbl[unit] 2.5e-07, "X-SHIFT"=w1166, "Y-SHIFT"=w1166, "PHI"=w1167, "THETA"=w1167) -> (w1169:T12)
                                n639 = local write "SCANNING"(w1169) -> ()
                              }
                              frame #4 {
                                n640 = Wait (ms)(milliseconds to wait=u32 500) -> ()  [unwired: 1 out]
                              }
                              frame #5 {
                                n641 = local write "STOP"(FALSE ("START")) -> ()
                              }
                            }
                          }
                        }
                      }
                      frame True {
                        n642 = stacked-sequence {
                          tunnel: w1187 -> [_ w1209 w1217 _ _ _]
                          tunnel: w1186 -> [_ w1208 w1216 _ _ _]
                          tunnel: w1188 -> [_ w1207 w1218 _ _ _]
                          tunnel: w1185 -> [w1189 _ _ _ _ _]
                          frame #0 {
                            n643 = Array Size(array=w1189) -> (size(s)=w1190:i32)
                            n644 = for {
                              N: w1190 -> [_]
                              tunnel: w1189 -> [w1199]
                              i -> [w1198]
                              n645 = Index Array(array=w1199, index=w1198) -> (element=w1197:T36)
                              n646 = Unbundle(w1197) -> ("ROI Type"=w1195:u32, "Points"=w1196:i32[])  [unwired: 1 out]
                              n647 = case shown="2" w1195 {
                                tunnel: w1196 -> [_ w1205]
                                tunnel: [w1200 w1204] -> w1194
                                tunnel: [w1200 w1203] -> w1193
                                tunnel: [w1200 w1202] -> w1192
                                tunnel: [w1200 w1201] -> w1191
                                frame 0, Default {
                                w1200 = 0 ("XCENTRE")
                                }
                                frame 2 {
                                n648 = Index Array(array=w1205) -> (element #1=w1204:i32, element #2=w1203:i32, element #3=w1202:i32, element #4=w1201:i32)  [unwired: 4 in]
                                }
                              }
                              "TOPX" <- w1194
                              "TOPY" <- w1193
                              "BOTTOMX" <- w1192
                              "BOTTOMY" <- w1191
                            }
                          }
                          frame #1 {
                            n649 = local read "POSITION"() -> (w1212:T3)
                            n650 = local read "TOPX"() -> (w1211:i32)
                            n651 = local read "TOPY"() -> (w1210:i32)
                            n652 = call "IMAGE 2 STAGE TRANSLATION.vi"("CENTREY"=w1208, "CENTREX"=w1209, "POSITION"=w1212, "CALIBRATION FACTOR"=w1207, "IMAGE Y"=w1210, "IMAGE X"=w1211) -> ("POINT POSITION"=w1206:cluster{dbl[unit], dbl[unit], "Z":dbl[unit]})  [unwired: 3 in, 2 out]
                            n653 = local write "TOP START"(w1206) -> ()
                          }
                          frame #2 {
                            n654 = local read "BOTTOMX"() -> (w1214:i32)
                            n655 = local read "BOTTOMY"() -> (w1215:i32)
                            n656 = local read "POSITION"() -> (w1219:T3)
                            n657 = call "IMAGE 2 STAGE TRANSLATION.vi"("CENTREY"=w1216, "CENTREX"=w1217, "POSITION"=w1219, "CALIBRATION FACTOR"=w1218, "IMAGE Y"=w1215, "IMAGE X"=w1214) -> ("POINT POSITION"=w1213:cluster{dbl[unit], dbl[unit], "Z":dbl[unit]})  [unwired: 3 in, 2 out]
                            n658 = local write "BOTTOM START"(w1213) -> ()
                          }
                          frame #3 {
                            n659 = local read "TOP START"() -> (w1227:T3)
                            n660 = local read "BOTTOM START"() -> (w1226:T3)
                            n661 = Subtract(x=w1227, y=w1226) -> (x-y=w1231:T3)
                            n662 = Add(x=w1227, y=w1226) -> (x+y=w1225:T3)
                            n663 = Unbundle By Name(w1231) -> ("Y"=w1230:dbl[unit])
                            n664 = Divide(x=w1225, y=2.0) -> (x/y=w1223:T3)
                            n665 = Absolute Value(x=w1230) -> (abs(x)=w1221:dbl[unit])
                            n666 = Unbundle By Name(w1223) -> ("Y"=→"YORIGIN":dbl[unit])
                            n667 = local read "SCANNING"() -> (w1229:T12)
                            n668 = Bundle By Name(cluster=w1229, "Y-AMP"=w1221, "dY"=dbl[unit] 2.5e-07) -> (w1228:T12)
                            n669 = local write "SCANNING"(w1228) -> ()
                          }
                          frame #4 {
                            n670 = Wait (ms)(milliseconds to wait=u32 500) -> ()  [unwired: 1 out]
                          }
                          frame #5 {
                            n671 = local write "START"(FALSE ("STOP")) -> ()
                          }
                        }
                      }
                    }
                  }
                  frame #1 {
                    n672 = local read "POSITION"() -> (w1235:T3)
                    n673 = local read "XORIGIN"() -> (w1237:dbl[unit])
                    n674 = local read "YORIGIN"() -> (w1238:dbl[unit])
                    n675 = local read "SCAN ORIGIN"() -> (w1234:T3)
                    n676 = Unbundle By Name(w1235) -> ("Z"=w1236:dbl[unit])
                    n677 = Bundle By Name(cluster=w1234, "X"=w1237, "Y"=w1238, "Z"=w1236) -> (w1239:T3)
                    n678 = local write "SCAN ORIGIN"(w1239) -> ()
                  }
                  frame #2 {
                  }
                }
              }
              event "START ROI", "STOP ROI": Mouse Down {
                n679 = event-data() -> ()  [unwired: 1 in, 8 out]
                n680 = invoke on="MICROSCOPE" class="ImageControl" method="Clear ROI"() -> ()  [unwired: 3 in, 3 out]
                n681 = flat-sequence {
                  frame #0 {
                    n682 = case shown="True" "START ROI" {
                      frame False {
                      }
                      frame True {
                        n683 = flat-sequence {
                          frame #0 {
                            n684 = local read "POSITION"() -> (w1245:T3)
                            n685 = local write "TOP LEFT"(w1245) -> ()
                          }
                          frame #1 {
                            n686 = local write "START ROI"(FALSE ("START ROI")) -> ()
                          }
                        }
                      }
                    }
                    n687 = case shown="True" "STOP ROI" {
                      frame False {
                      }
                      frame True {
                        n688 = flat-sequence {
                          frame #0 {
                            n689 = local read "POSITION"() -> (w1243:T3)
                            n690 = local write "BOTTOM RIGHT"(w1243) -> ()
                          }
                          frame #1 {
                            n691 = local write "STOP ROI"(FALSE ("STOP ROI")) -> ()
                          }
                        }
                      }
                    }
                  }
                  frame #1 {
                    n692 = local read "BOTTOM RIGHT"() -> (w1255:T3)
                    n693 = local read "TOP LEFT"() -> (w1256:T3)
                    n694 = Subtract(x=w1256, y=w1255) -> (x-y=w1258:T3)
                    n695 = Unbundle By Name(w1256) -> ("X"=w1266:dbl[unit], "Y"=w1270:dbl[unit])
                    n696 = Absolute Value(x=w1258) -> (abs(x)=w1259:T3)
                    n697 = Unbundle By Name(w1259) -> ("X"=w1264:dbl[unit], "Y"=w1268:dbl[unit])
                    n698 = local read "POSITION"() -> (w1251:T3)
                    n699 = Divide(x=w1268, y=2.0) -> (x/y=w1271:dbl[unit])
                    n700 = Divide(x=w1264, y=2.0) -> (x/y=w1265:dbl[unit])
                    n701 = node(w1264) -> (w1262:dbl)
                    n702 = node(w1268) -> (w1263:dbl)
                    n703 = Subtract(x=w1266, y=w1265) -> (x-y=w1248:dbl[unit])
                    "XORIGIN" <- w1248
                    n704 = Add(x=w1270, y=w1271) -> (x+y=w1247:dbl[unit])
                    "YORIGIN" <- w1247
                    n705 = Unbundle By Name(w1251) -> ("Z"=w1269:dbl[unit])
                    n706 = Round To Nearest(number=w1262) -> (nearest integer value=w1260:dbl)
                    n707 = Round To Nearest(number=w1263) -> (nearest integer value=w1261:dbl)
                    n708 = node(w1261) -> (w1249:dbl[unit])
                    "YAMP" <- w1249
                    n709 = node(w1260) -> (w1250:dbl[unit])
                    "XAMP" <- w1250
                    n710 = Bundle By Name(cluster=w1251, "X"=w1248, "Y"=w1247, "Z"=w1269) -> (w1254:T3)
                    n711 = local read "SCANNING"() -> (w1252:T12)
                    n712 = Bundle By Name(cluster=w1252, "X-AMP"=w1250, "Y-AMP"=w1249) -> (w1253:T12)
                    n713 = local write "SCAN ORIGIN"(w1254) -> ()
                    n714 = local write "SCANNING"(w1253) -> ()
                  }
                }
              }
              event "RELATIVE": Mouse Down {
                # "Free Corner Position on GeoStub 1"
                n715 = event-data() -> ()  [unwired: 1 in, 8 out]
                n716 = flat-sequence {
                  frame #0 {
                    n717 = local read "POSITION"() -> (w1276:T3)
                    n718 = Add(x=w1276, y="RELATIVE MOVE") -> (x+y=w1274:T3)
                    n719 = local write "GOTO POSITION"(w1274) -> ()
                  }
                  frame #1 {
                    n720 = local write "RELATIVE MOVE"(T3 {"X"=0.0, "Y"=0.0, "Z"=0.0} ("RELATIVE MOVE")) -> ()
                  }
                }
              }
              event "GOTO SCAN ORIGIN": Mouse Down {
                n721 = event-data() -> ()  [unwired: 1 in, 8 out]
                n722 = local read "SCAN ORIGIN"() -> (w1278:T3)
                n723 = local write "GOTO POSITION"(w1278) -> ()
              }
              event "DEFINE APERTURE": Mouse Down {
                n724 = event-data() -> ()  [unwired: 1 in, 8 out]
                n725 = flat-sequence {
                  frame #0 {
                    n726 = local read "LANDMARKS FOR HOLDERS"() -> (w1279:T14)
                    n727 = local read "SAMPLE HOLDER"() -> (w1282:u16)
                    n728 = local read "POSITION"() -> (w1281:T3)
                    n729 = Replace Array Subset(array=w1279, new element=w1281, index=w1282) -> (w1280:T14)
                    n730 = local write "LANDMARKS FOR HOLDERS"(w1280) -> ()
                  }
                  frame #1 {
                    n731 = local write "DEFINE APERTURE"(FALSE ("DEFINE APERTURE")) -> ()
                  }
                }
              }
              event "GOTO GEOSTUB #1 APERTURE": Value Change {
                n732 = event-data() -> ()  [unwired: 1 in, 6 out]
                n733 = local read "SAMPLE HOLDER"() -> (w1286:u16)
                n734 = local read "LANDMARKS FOR HOLDERS"() -> (w1287:T14)
                n735 = Index Array(array=w1287, index=w1286) -> (element=w1285:T3)
                n736 = local write "GOTO GEOSTUB #1 APERTURE"(FALSE ("GOTO GEOSTUB #1 APERTURE")) -> ()
                n737 = local write "GOTO POSITION"(w1285) -> ()
              }
              event "GOTO LIST POINT": Mouse Down {
                n738 = event-data() -> ()  [unwired: 1 in, 8 out]
                n739 = local read "SCAN LIST ARRAY"() -> (w1291:T2)
                n740 = local read "SCAN ROW"() -> (w1290:i32)
                n741 = Index Array(array=w1291, index=w1290) -> (element=w1289:T39)
                n742 = Unbundle By Name(w1289) -> ("SCAN ORIGIN"=w1288:T3)
                n743 = local write "GOTO POSITION"(w1288) -> ()
              }
              event "GOTO LIST POINT 2": Mouse Down {
                n744 = event-data() -> ()  [unwired: 1 in, 8 out]
                n745 = local read "EXT POINTS ROW"() -> (w1297:i32)
                n746 = local read "TRANS POINT ARRAY"() -> (w1298:T5)
                n747 = Index Array(array=w1298, index=w1297) -> (element=w1299:T40)
                n748 = Unbundle By Name(w1299) -> ("X"=w1295:dbl[unit], "Y"=w1294:dbl[unit], "Z"=w1293:dbl[unit])
                n749 = Bundle By Name(cluster=T3 {"X"=-0.021830232999999998, "Y"=0.017859033000000003, "Z"=0.0008} ("GOTO POSITION"), "X"=w1295, "Y"=w1294, "Z"=w1293) -> (w1292:T3)
                n750 = local write "GOTO POSITION"(w1292) -> ()
              }
              event "SET SCAN FROM LIST": Mouse Down {
                n751 = event-data() -> ()  [unwired: 1 in, 8 out]
                n752 = local read "SCAN LIST ARRAY"() -> (w1312:T2)
                n753 = local read "SCAN ROW"() -> (w1300:i32)
                n754 = Index Array(array=w1312, index=w1300) -> (element=w1316:T39)
                n755 = Unbundle By Name(w1316) -> ("SCAN ORIGIN.X"=w1314:dbl[unit], "SCAN ORIGIN.Y"=w1315:dbl[unit], "SCAN ORIGIN.Z"=w1313:dbl[unit], "PIXEL DEPTH"=w1309:bool, "DOSE NORM"=w1310:i8, "MODE & METHOD"=w1308:cluster{"SCAN MODE":u16, "SCANNING METH":u16}, "Q"=w1307:dbl[unit], "dQ"=w1306:dbl[unit], "DWELL"=w1305:sgl[unit], "dt"=w1304:sgl[unit], "SCANNING"=w1303:T12, "OVERSCAN"=w1302:i32, "LINE PASSES"=w1301:i32)
                n756 = Bundle("X"=w1314, "Y"=w1315, "Z"=w1313) -> (w1311:T3)  [unwired: 1 in]
                n757 = local write "OVERSCAN"(w1302) -> ()
                n758 = local write "LINE PASSES"(w1301) -> ()
                n759 = local write "SCANNING"(w1303) -> ()
                n760 = local write "PIXEL DEPTH"(w1309) -> ()
                n761 = local write "DOSE NORM"(w1310) -> ()
                n762 = local write "MODE & METHOD"(w1308) -> ()
                n763 = local write "Q"(w1307) -> ()
                n764 = local write "dQ"(w1306) -> ()
                n765 = local write "DWELL"(w1305) -> ()
                n766 = local write "dt"(w1304) -> ()
                n767 = local write "GOTO POSITION"(w1311) -> ()
              }
              event "SET FIDUCIAL 1": Mouse Down {
                n768 = event-data() -> ()  [unwired: 1 in, 8 out]
                n769 = local read "POSITION"() -> (w1317:T3)
                n770 = local write "REF#1"(w1317) -> ()
              }
              event "SET FIDUCIAL 2": Mouse Down {
                n771 = event-data() -> ()  [unwired: 1 in, 8 out]
                n772 = local read "POSITION"() -> (w1318:T3)
                n773 = local write "REF#2"(w1318) -> ()
              }
              event "YAP": Mouse Down {
                n774 = event-data() -> ()  [unwired: 1 in, 7 out]
                n775 = flat-sequence {
                  frame #0 {
                    n776 = local write "GOTO POSITION"(T3 {"X"=-0.034219, "Y"=0.011425000000000001, "Z"=-0.00292} ("XYZ STAGE")) -> ()
                  }
                  frame #1 {
                    n777 = Wait (ms)(milliseconds to wait=u32 2000) -> ()  [unwired: 1 out]
                  }
                  frame #2 {
                    n778 = local write "YAP"(FALSE ("YAP")) -> ()
                  }
                }
              }
              event "EXCHANGE": Mouse Down {
                n779 = event-data() -> ()  [unwired: 1 in, 7 out]
                n780 = flat-sequence {
                  frame #0 {
                    n781 = local write "GOTO POSITION"(T3 {"X"=-0.02106, "Y"=-0.017932, "Z"=-0.0010040000000000001} ("XYZ STAGE")) -> ()
                  }
                  frame #1 {
                    n782 = Wait (ms)(milliseconds to wait=u32 2000) -> ()  [unwired: 1 out]
                  }
                  frame #2 {
                    n783 = local write "EXCHANGE"(FALSE ("EXCHANGE")) -> ()
                  }
                }
              }
              event "GOTOF1": Mouse Down {
                n784 = event-data() -> ()  [unwired: 1 in, 8 out]
                n785 = local read "REF#1"() -> (w1327:T3)
                n786 = local write "GOTO POSITION"(w1327) -> ()
              }
              event "GOTOF2": Mouse Down {
                n787 = event-data() -> ()  [unwired: 1 in, 8 out]
                n788 = local read "REF#2"() -> (w1329:T3)
                n789 = local write "GOTO POSITION"(w1329) -> ()
              }
              event "YAG": Mouse Down {
                n790 = event-data() -> ()  [unwired: 1 in, 7 out]
                n791 = flat-sequence {
                  frame #0 {
                    n792 = local write "GOTO POSITION"(T3 {"X"=-0.041100000000000005, "Y"=0.005466, "Z"=-0.00292} ("XYZ STAGE")) -> ()
                  }
                  frame #1 {
                    n793 = Wait (ms)(milliseconds to wait=u32 2000) -> ()  [unwired: 1 out]
                  }
                  frame #2 {
                    n794 = local write "YAG"(FALSE ("YAG")) -> ()
                  }
                }
              }
              event "RUBY": Mouse Down {
                n795 = event-data() -> ()  [unwired: 1 in, 7 out]
                n796 = flat-sequence {
                  frame #0 {
                    n797 = local write "GOTO POSITION"(T3 {"X"=-0.044469, "Y"=0.010784, "Z"=-0.001477} ("POSITION")) -> ()
                  }
                  frame #1 {
                    n798 = Wait (ms)(milliseconds to wait=u32 2000) -> ()  [unwired: 1 out]
                  }
                  frame #2 {
                    n799 = local write "RUBY"(FALSE ("RUBY")) -> ()
                  }
                }
              }
              event "GRID I": Mouse Down {
                # "Grid on slide Zoom1"
                # "grid on geostub 1"
                n800 = event-data() -> ()  [unwired: 1 in, 7 out]
                n801 = flat-sequence {
                  frame #0 {
                    n802 = local read "SAMPLE HOLDER"() -> (w1341:u16)
                    n803 = case shown="0, Default" w1341 {
                      tunnel: [T3 {"X"=-0.034151, "Y"=-0.003799, "Z"=-0.002295} ("XYZ STAGE") T3 {"X"=-0.02182, "Y"=0.017865, "Z"=0.00038} ("XYZ STAGE") T3 {"X"=0.022995, "Y"=0.010199999999999999, "Z"=0.00083} ("XYZ STAGE")] -> w1340
                      frame 0, Default {
                      }
                      frame 1 {
                      }
                      frame 2 {
                      }
                    }
                    n804 = local write "GOTO POSITION"(w1340) -> ()
                  }
                  frame #1 {
                    n805 = Wait (ms)(milliseconds to wait=u32 1000) -> ()  [unwired: 1 out]
                  }
                  frame #2 {
                    n806 = local write "GRID I"(FALSE ("GRID I")) -> ()
                  }
                }
              }
              event "TOMO POINT": Mouse Down {
                n807 = event-data() -> ()  [unwired: 1 in, 7 out]
                n808 = local write "GOTO POSITION"(T3 {"X"=0.0359, "Y"=-0.001, "Z"=-0.0022500000000000003} ("XYZ STAGE")) -> ()
              }
              event "QUARTZ": Mouse Down {
                n809 = event-data() -> ()  [unwired: 1 in, 7 out]
                n810 = flat-sequence {
                  frame #0 {
                    n811 = local read "SAMPLE HOLDER"() -> (w1351:u16)
                    n812 = case shown="0, Default" w1351 {
                      tunnel: [T3 {"X"=-0.035988, "Y"=0.0166, "Z"=-0.003} ("XYZ STAGE") T3 {"X"=-0.039429000000000006, "Y"=-0.010206, "Z"=-0.0005} ("XYZ STAGE") T3 {"X"=0.013375, "Y"=0.016038, "Z"=0.002326} ("XYZ STAGE")] -> w1350
                      frame 0, Default {
                      }
                      frame 1 {
                      }
                      frame 2 {
                      }
                    }
                    n813 = local write "GOTO POSITION"(w1350) -> ()
                  }
                  frame #1 {
                    n814 = Wait (ms)(milliseconds to wait=u32 1000) -> ()  [unwired: 1 out]
                  }
                  frame #2 {
                    n815 = local write "QUARTZ"(FALSE ("QUARTZ")) -> ()
                  }
                }
              }
              event "LEFT": Mouse Down {
                n816 = event-data() -> ()  [unwired: 1 in, 7 out]
                n817 = local read "POSITION"() -> (w1361:T3)
                n818 = local read "DX"() -> (w1358:dbl[unit])
                n819 = Unbundle By Name(w1361) -> ("X"=w1365:dbl[unit], "Y"=w1360:dbl[unit], "Z"=w1359:dbl[unit])
                n820 = Negate(x=w1358) -> (-x=w1357:dbl[unit])
                n821 = Add(x=w1357, y=w1365) -> (x+y=w1363:dbl[unit])
                n822 = Bundle By Name(cluster=w1361, "X"=w1363, "Y"=w1360, "Z"=w1359) -> (w1362:T3)
                n823 = local write "GOTO POSITION"(w1362) -> ()
              }
              event "RIGHT": Mouse Down {
                n824 = event-data() -> ()  [unwired: 1 in, 7 out]
                n825 = local read "POSITION"() -> (w1369:T3)
                n826 = local read "DX"() -> (w1366:dbl[unit])
                n827 = Unbundle By Name(w1369) -> ("X"=w1373:dbl[unit], "Y"=w1368:dbl[unit], "Z"=w1367:dbl[unit])
                n828 = Add(x=w1366, y=w1373) -> (x+y=w1371:dbl[unit])
                n829 = Bundle By Name(cluster=w1369, "X"=w1371, "Y"=w1368, "Z"=w1367) -> (w1370:T3)
                n830 = local write "GOTO POSITION"(w1370) -> ()
              }
              event "DOWN": Mouse Down {
                n831 = event-data() -> ()  [unwired: 1 in, 7 out]
                n832 = local read "POSITION"() -> (w1379:T3)
                n833 = local read "DY"() -> (w1375:dbl[unit])
                n834 = Unbundle By Name(w1379) -> ("X"=w1378:dbl[unit], "Y"=w1380:dbl[unit], "Z"=w1381:dbl[unit])
                n835 = Negate(x=w1375) -> (-x=w1374:dbl[unit])
                n836 = Add(x=w1374, y=w1380) -> (x+y=w1377:dbl[unit])
                n837 = Bundle By Name(cluster=w1379, "X"=w1378, "Y"=w1377, "Z"=w1381) -> (w1376:T3)
                n838 = local write "GOTO POSITION"(w1376) -> ()
              }
              event "UP": Mouse Down {
                n839 = event-data() -> ()  [unwired: 1 in, 7 out]
                n840 = local read "POSITION"() -> (w1387:T3)
                n841 = local read "DY"() -> (w1383:dbl[unit])
                n842 = Unbundle By Name(w1387) -> ("X"=w1386:dbl[unit], "Y"=w1388:dbl[unit], "Z"=w1389:dbl[unit])
                n843 = Add(x=w1383, y=w1388) -> (x+y=w1385:dbl[unit])
                n844 = Bundle By Name(cluster=w1387, "X"=w1386, "Y"=w1385, "Z"=w1389) -> (w1384:T3)
                n845 = local write "GOTO POSITION"(w1384) -> ()
              }
              event "OUT": Mouse Down {
                n846 = event-data() -> ()  [unwired: 1 in, 7 out]
                n847 = local read "POSITION"() -> (w1392:T3)
                n848 = local read "DZ"() -> (w1391:dbl[unit])
                n849 = Unbundle By Name(w1392) -> ("X"=w1396:dbl[unit], "Y"=w1395:dbl[unit], "Z"=w1397:dbl[unit])
                n850 = Add(x=w1397, y=w1391) -> (x+y=w1394:dbl[unit])
                n851 = Bundle By Name(cluster=w1392, "X"=w1396, "Y"=w1395, "Z"=w1394) -> (w1393:T3)
                n852 = local write "GOTO POSITION"(w1393) -> ()
              }
              event "IN": Mouse Down {
                n853 = event-data() -> ()  [unwired: 1 in, 7 out]
                n854 = local read "POSITION"() -> (w1400:T3)
                n855 = local read "DZ"() -> (w1405:dbl[unit])
                n856 = Unbundle By Name(w1400) -> ("X"=w1404:dbl[unit], "Y"=w1403:dbl[unit], "Z"=w1406:dbl[unit])
                n857 = Negate(x=w1405) -> (-x=w1399:dbl[unit])
                n858 = Add(x=w1406, y=w1399) -> (x+y=w1402:dbl[unit])
                n859 = Bundle By Name(cluster=w1400, "X"=w1404, "Y"=w1403, "Z"=w1402) -> (w1401:T3)
                n860 = local write "GOTO POSITION"(w1401) -> ()
              }
              event "WOBBLEZ": Mouse Down {
                n861 = event-data() -> ()  [unwired: 1 in, 7 out]
                n862 = local read "POSITION"() -> (w1409:T3)
                n863 = while {
                  shift-right: [w1411] -> _
                  shift-left: TRUE -> [w1412]
                  tunnel: w1409 -> [w1419]
                  stop <- "WOBBLEZ" continue-if-true
                  n864 = local read "DZ"() -> (w1414:dbl[unit])
                  n865 = Negate(x=w1414) -> (-x=w1415:dbl[unit])
                  n866 = Unbundle By Name(w1419) -> ("X"=w1421:dbl[unit], "Y"=w1420:dbl[unit], "Z"=w1422:dbl[unit])
                  n867 = Select(t=w1415, s=w1412, f=w1414) -> (s? t:f=w1413:dbl[unit])
                  n868 = Wait (ms)(milliseconds to wait=u32 500) -> ()  [unwired: 1 out]
                  n869 = Add(x=w1422, y=w1413) -> (x+y=w1423:dbl[unit])
                  n870 = Bundle(cluster=w1419, "X"=w1421, "Y"=w1420, "Z"=w1423) -> (w1416:T3)
                  n871 = local write "GOTO POSITION"(w1416) -> ()
                  n872 = Not(x=w1412) -> (.not. x?=w1411:bool)
                }
              }
              event "LOAD ROI": Mouse Down {
                n873 = event-data() -> ()  [unwired: 1 in, 8 out]
                n874 = property on="NEW ROI" class="Clust (strict)"() -> ("Value"=w1426:T4)  [unwired: 2 in, 2 out]
                n875 = local read "CURRENT ZOOM CAL"() -> (w1429:dbl)
                n876 = local read "MODE & METHOD"() -> (w1434:cluster{"SCAN MODE":u16, "SCANNING METH":u16})
                n877 = Unbundle By Name(w1426) -> ("Contours"=w1432:T19)
                n878 = local read "IMAGE XCENTRE"() -> (w1428:dbl)
                n879 = local read "IMAGE YCENTRE"() -> (w1427:dbl)
                n880 = local read "BEAM OFFSET"() -> (w1430:cluster{"X":dbl[unit], "Y":dbl[unit]})
                n881 = local read "POSITION"() -> (w1431:T3)
                n882 = Array Size(array=w1432) -> (size(s)=w1424:i32)
                n883 = Equal To 0?(x=w1424) -> (x = 0?=w1425:bool)
                n884 = Unbundle By Name(w1434) -> ("SCAN MODE"=w1433:u16)
                n885 = case shown="False" w1425 {
                  tunnel: w1433 -> [w1442 w1522]
                  tunnel: w1432 -> [w1441 _]
                  tunnel: w1424 -> [w1440 _]
                  tunnel: w1431 -> [w1439 w1523]
                  tunnel: w1430 -> [w1438 _]
                  tunnel: w1429 -> [w1437 _]
                  tunnel: w1428 -> [w1436 _]
                  tunnel: w1427 -> [w1435 _]
                  frame False {
                    n886 = for {
                      N: w1440 -> [_]
                      tunnel: w1439 -> [w1449]
                      tunnel: w1437 -> [w1448]
                      tunnel: w1436 -> [w1447]
                      tunnel: w1435 -> [w1446]
                      tunnel: w1441 -> [w1445] mode=indexing
                      tunnel: w1442 -> [w1444]
                      tunnel: w1438 -> [w1443]
                      n887 = Unbundle By Name(w1445) -> ("ROI Type"=w1450:u32, "Points"=w1451:i32[])
                      n888 = stacked-sequence {
                        tunnel: w1451 -> [w1458 _]
                        tunnel: w1450 -> [w1457 _]
                        tunnel: w1449 -> [w1456 w1488]
                        tunnel: w1448 -> [w1455 _]
                        tunnel: w1447 -> [w1454 _]
                        tunnel: w1446 -> [w1453 _]
                        tunnel: w1443 -> [w1452 w1508]
                        tunnel: w1444 -> [_ w1507]
                        frame #0 {
                          n889 = case shown="1" w1457 {
                            tunnel: w1458 -> [w1468 w1479]
                            tunnel: w1456 -> [w1460 w1476]
                            tunnel: w1455 -> [w1463 w1471]
                            tunnel: w1454 -> [w1462 w1470]
                            tunnel: w1453 -> [w1461 w1469]
                            tunnel: w1452 -> [_ _]
                            frame 1 {
                              # "POINT"
                              n890 = Index Array(array=w1468, index #1=0 ("index"), index #2=1 ("index")) -> (element #1=w1465:i32, element #2=w1464:i32)
                              n891 = call "IMAGE 2 STAGE TRANSLATION.vi"("CENTREY"=w1461, "CENTREX"=w1462, "POSITION"=w1460, "CALIBRATION FACTOR"=w1463, "IMAGE Y"=w1464, "IMAGE X"=w1465) -> ("POINT POSITION"=→"POINT":cluster{dbl[unit], dbl[unit], "Z":dbl[unit]})  [unwired: 3 in, 2 out]
                            }
                            frame 3, Default {
                              # "RECTANGLE"
                              n892 = Index Array(array=w1479, index #1=0 ("index"), index #2=1 ("index"), index #3=2 ("index"), index #4=3 ("index")) -> (element #1=w1478:i32, element #2=w1477:i32, element #3=w1475:i32, element #4=w1474:i32)
                              n893 = call "IMAGE 2 STAGE TRANSLATION.vi"("CENTREY"=w1469, "CENTREX"=w1470, "POSITION"=w1476, "CALIBRATION FACTOR"=w1471, "IMAGE Y"=w1477, "IMAGE X"=w1478) -> ("POINT POSITION"=→"TOP LEFT":cluster{dbl[unit], dbl[unit], "Z":dbl[unit]})  [unwired: 3 in, 2 out]
                              n894 = call "IMAGE 2 STAGE TRANSLATION.vi"("CENTREY"=w1469, "CENTREX"=w1470, "POSITION"=w1476, "CALIBRATION FACTOR"=w1471, "IMAGE Y"=w1474, "IMAGE X"=w1475) -> ("POINT POSITION"=→"BOTTOM RIGHT":cluster{dbl[unit], dbl[unit], "Z":dbl[unit]})  [unwired: 3 in, 2 out]
                            }
                          }
                        }
                        frame #1 {
                          # "XY ELECTRO SCAN"
                          n895 = Unbundle By Name(w1508) -> ()  [unwired: 2 out]
                          n896 = local read "BOTTOM RIGHT"() -> (w1497:T3)
                          n897 = local read "TOP LEFT"() -> (w1494:T3)
                          n898 = Subtract(x=w1494, y=w1497) -> (x-y=w1505:T3)
                          n899 = Unbundle By Name(w1494) -> ("X"=w1493:dbl[unit], "Y"=w1486:dbl[unit])
                          n900 = Absolute Value(x=w1505) -> (abs(x)=w1504:T3)
                          n901 = Unbundle By Name(w1504) -> ("X"=w1496:dbl[unit], "Y"=w1489:dbl[unit])
                          n902 = Divide(x=w1489, y=2.0) -> (x/y=w1485:dbl[unit])
                          n903 = Divide(x=w1496, y=2.0) -> (x/y=w1495:dbl[unit])
                          n904 = node(w1496) -> (w1501:dbl)
                          n905 = node(w1489) -> (w1500:dbl)
                          n906 = Subtract(x=w1493, y=w1495) -> (x-y=w1491:dbl[unit])
                          n907 = Add(x=w1486, y=w1485) -> (x+y=w1484:dbl[unit])
                          n908 = Unbundle By Name(w1488) -> ("Z"=w1487:dbl[unit])
                          n909 = Round To Nearest(number=w1501) -> (nearest integer value=w1503:dbl)
                          n910 = Round To Nearest(number=w1500) -> (nearest integer value=w1502:dbl)
                          n911 = node(w1502) -> (w1498:dbl[unit])
                          n912 = node(w1503) -> (w1499:dbl[unit])
                          n913 = Bundle By Name(cluster=w1488, "X"=w1491, "Y"=w1484, "Z"=w1487) -> (w1492:T3)
                          n914 = local write "SCAN ORIGIN"(w1492) -> ()
                          n915 = case shown="0, Default" w1507 {
                            tunnel: w1499 -> [w1511 w1516]
                            tunnel: w1498 -> [w1510 w1515]
                            frame 0, Default {
                              w1509 = dbl[unit] 2.5e-07  # um
                              n916 = local read "SCANNING"() -> (w1513:T12)
                              n917 = Bundle By Name(cluster=w1513, "X-AMP"=w1511, "Y-AMP"=w1510, "dY"=w1509, "dX"=w1509) -> (w1512:T12)
                              n918 = local write "SCANNING"(w1512) -> ()
                            }
                            frame 2 {
                              w1514 = dbl[unit] 1e-06  # um
                              n919 = local read "SCANNING"() -> (w1518:T12)
                              n920 = Bundle By Name(cluster=w1518, "X-AMP"=w1516, "Y-AMP"=w1515, "dY"=w1514, "dX"=w1514) -> (w1517:T12)
                              n921 = local write "SCANNING"(w1517) -> ()
                            }
                          }
                        }
                      }
                    }
                  }
                  frame True {
                    n922 = local read "BOTTOM RIGHT"() -> (w1524:T3)
                    n923 = local read "TOP LEFT"() -> (w1525:T3)
                    n924 = Subtract(x=w1525, y=w1524) -> (x-y=w1541:T3)
                    n925 = Unbundle By Name(w1525) -> ("X"=w1533:dbl[unit], "Y"=w1528:dbl[unit])
                    n926 = Absolute Value(x=w1541) -> (abs(x)=w1540:T3)
                    n927 = Unbundle By Name(w1540) -> ("X"=w1535:dbl[unit], "Y"=w1530:dbl[unit])
                    n928 = Divide(x=w1530, y=2.0) -> (x/y=w1527:dbl[unit])
                    n929 = Divide(x=w1535, y=2.0) -> (x/y=w1534:dbl[unit])
                    n930 = node(w1535) -> (w1537:dbl)
                    n931 = node(w1530) -> (w1536:dbl)
                    n932 = Subtract(x=w1533, y=w1534) -> (x-y=w1532:dbl[unit])
                    n933 = Add(x=w1528, y=w1527) -> (x+y=w1526:dbl[unit])
                    n934 = Unbundle By Name(w1523) -> ("Z"=w1529:dbl[unit])
                    n935 = Round To Nearest(number=w1537) -> (nearest integer value=w1539:dbl)
                    n936 = Round To Nearest(number=w1536) -> (nearest integer value=w1538:dbl)
                    n937 = node(w1538) -> (w1520:dbl[unit])
                    n938 = node(w1539) -> (w1521:dbl[unit])
                    n939 = Bundle By Name(cluster=w1523, "X"=w1532, "Y"=w1526, "Z"=w1529) -> (w1519:T3)
                    n940 = local write "SCAN ORIGIN"(w1519) -> ()
                    n941 = case shown="2" w1522 {
                      tunnel: w1521 -> [w1547 w1550]
                      tunnel: w1520 -> [w1546 w1549]
                      frame 0, Default {
                        w1543 = dbl[unit] 2.5e-07  # um
                        n942 = local read "SCANNING"() -> (w1545:T12)
                        n943 = Bundle By Name(cluster=w1545, "X-AMP"=w1547, "Y-AMP"=w1546, "dY"=w1543, "dX"=w1543) -> (w1544:T12)
                        n944 = local write "SCANNING"(w1544) -> ()
                      }
                      frame 2 {
                        w1548 = dbl[unit] 1e-06  # um
                        n945 = local read "SCANNING"() -> (w1551:T12)
                        n946 = Bundle By Name(cluster=w1551, "X-AMP"=w1550, "Y-AMP"=w1549, "dY"=w1548, "dX"=w1548) -> (w1552:T12)
                        n947 = local write "SCANNING"(w1552) -> ()
                      }
                    }
                  }
                }
              }
              event "START": Mouse Down {
                n948 = event-data() -> ()  [unwired: 1 in, 8 out]
                n949 = local read "MODE & METHOD"() -> (w1554:cluster{"SCAN MODE":u16, "SCANNING METH":u16})
                n950 = Unbundle By Name(w1554) -> ("SCAN MODE"=w1553:u16)
                n951 = case shown="3" w1553 {
                  tunnel: "X" -> [_ w1566]
                  tunnel: "Y" -> [_ w1565]
                  tunnel: "Z" -> [_ w1564]
                  frame 0, Default {
                    n952 = local write "FARADAY CUP"(FALSE ("FARADAY CUP")) -> ()
                  }
                  frame 3 {
                    n953 = local read "SCAN LIST ARRAY"() -> (w1563:T2)
                    n954 = flat-sequence {
                      tunnel: w1564 -> [w1571]
                      tunnel: w1565 -> [w1572]
                      tunnel: w1566 -> [w1573]
                      tunnel: w1563 -> [w1570]
                      tunnel: [w1573] -> w1562
                      tunnel: [w1572] -> w1561
                      tunnel: [w1571] -> w1560
                      tunnel: [w1569] -> w1559
                      tunnel: w1562 -> [_]
                      tunnel: w1561 -> [_]
                      tunnel: w1560 -> [_]
                      tunnel: w1559 -> [w1585]
                      frame #0 {
                        n955 = local read "SCAN ROW"() -> (w1568:i32)
                        n956 = local write "FARADAY CUP"(FALSE ("FARADAY CUP")) -> ()
                        n957 = Index Array(array=w1570, index=w1568) -> (element=w1569:T39)
                      }
                      frame #1 {
                        n958 = Unbundle By Name(w1585) -> ("SCAN ORIGIN"=w1584:T3, "PIXEL DEPTH"=w1580:bool, "DOSE NORM"=w1579:i8, "MODE & METHOD"=w1578:cluster{"SCAN MODE":u16, "SCANNING METH":u16}, "Q"=w1576:dbl[unit], "dQ"=w1575:dbl[unit], "DWELL"=w1577:sgl[unit], "dt"=w1574:sgl[unit], "SCANNING"=w1583:T12, "OVERSCAN"=w1582:i32, "LINE PASSES"=w1581:i32)
                        n959 = local write "MODE & METHOD"(w1578) -> ()
                        n960 = local write "OVERSCAN"(w1582) -> ()
                        n961 = local write "LINE PASSES"(w1581) -> ()
                        n962 = local write "SCANNING"(w1583) -> ()
                        n963 = local write "SCAN ORIGIN"(w1584) -> ()
                        n964 = local write "PIXEL DEPTH"(w1580) -> ()
                        n965 = local write "DOSE NORM"(w1579) -> ()
                        n966 = local write "Q"(w1576) -> ()
                        n967 = local write "dQ"(w1575) -> ()
                        n968 = local write "DWELL"(w1577) -> ()
                        n969 = local write "dt"(w1574) -> ()
                      }
                      frame #2 {
                        n970 = Wait (ms)(milliseconds to wait=u32 50) -> ()  [unwired: 1 out]
                      }
                      frame #3 {
                        n971 = while {
                          stop <- w1587 stop-if-true
                          n972 = local read "SCAN COMPLETE"() -> (w1587:bool)
                          n973 = Wait (ms)(milliseconds to wait=u32 50) -> ()  [unwired: 1 out]
                        }
                      }
                      frame #4 {
                        n974 = local write "FARADAY CUP"(TRUE ("FARADAY CUP")) -> ()
                      }
                    }
                  }
                }
              }
            }
            n975 = local read "GLOBAL STOP"() -> (w638:bool)
          }
        }
      }
    }
    frame #3 {
    }
  }
